vi "Vibration.vi"(0 "Channel 4":T5={"Frequency"=20, "Signal type"=enum."Sine Wave", "Amplitude"=2.0, "Offset"=0.0, "Phase"=0.0} {"Phase" format="%.2p"; "Offset" format="%0.2p"; "Amplitude" min=-2.0 max=2.0 step=0.1 format="%0.2p"}, 1 "Channel 3":T5={"Frequency"=20, "Signal type"=enum."Sine Wave", "Amplitude"=2.0, "Offset"=0.0, "Phase"=0.0} {"Phase" format="%.2p"; "Offset" format="%0.2p"; "Amplitude" min=-2.0 max=2.0 step=0.1 format="%0.2p"}, 2 "Channel 2":T5={"Frequency"=20, "Signal type"=enum."Sine Wave", "Amplitude"=2.0, "Offset"=0.0, "Phase"=0.0} {"Phase" format="%.2p"; "Offset" format="%0.2p"; "Amplitude" min=-2.0 max=2.0 step=0.1 format="%0.2p"}, 3 "Channel 1":T8={" Frequency"=20, "Signal type"=enum."Sine Wave", "Amplitude"=2.0, "Offset"=0.0, "Phase"=0.0} {"Phase" format="%.2p"; "Offset" format="%0.2p"; "Amplitude" min=-2.0 max=2.0 step=0.1 format="%0.2p"}, 4 "Time(ms)":i32, 5 "Model List":i32(listbox), 6 "Play Button":bool, 7 "Project Name":string, 9 "OK Button":bool, 10 "Remove Project":bool, 11 "Add Project":bool) -> (8 "Tab Control":enum32{"Main", "Project", "Set"}(tab)=enum."Project")   [LabVIEW 2019]
uses:
  Ctrl/UpLoad2.ctl
  Ctrl/Remove.ctl
  Typedef/Test_State.ctl
  Ctrl/left2arrow.ctl
  Ctrl/Right2arrow.ctl
  <vilib>/Utility/miscctls.llb/LVPointTypeDef.ctl
  <vilib>/Utility/miscctls.llb/LVPositionTypeDef.ctl
  Typedef/State.ctl
  Typedef/Data.ctl
  Typedef/Timer State.ctl
  LLB/Message/Ctrl/MsgDataInput.ctl
  LLB/Message/Ctrl/MsgPageSelect.ctl
  LLB/Message/Ctrl/LogType.ctl
  <vilib>/Utility/xml.llb/Read From XML File(string).vi
  LLB/Commonly VI/Main Glb.vi
  Class/Main Process Class/MPC_VirbVision/Panel RefGlb.vi
  SubVIs/GBV_Ref.vi
  <vilib>/Utility/xml.llb/Write to XML File(string).vi
  <vilib>/measure/NI_MABase.lvlib
  <vilib>/Utility/config.llb/NI_LVConfig.lvlib
  <resource>/objmgr/daqmx.rc
  LLB/Commonly VI.lvlib
  LLB/Message/MsgShowAndLog.lvlib
  <vilib>/Utility/config.llb/Read Key (String).vi
panel:
  in  "Reply":bool=TRUE
  in  "SubUI":bool=TRUE
  out "TCP connect":bool
  out "Array":string[](array[string])
  in  "Channel 4 Sample":cluster{"Sample Rate":dbl, "Samples":dbl} {"Samples" format="%#.2f"; "Sample Rate" format="%#.2f"}
  in  "Channel 3 Sample":cluster{"Sample Rate":dbl, "Samples":dbl} {"Samples" format="%#.2f"; "Sample Rate" format="%#.2f"}
  in  "Channel 2 Sample":cluster{"Sample Rate":dbl, "Samples":dbl} {"Samples" format="%#.2f"; "Sample Rate" format="%#.2f"}
  in  "Channel 1 Sample":cluster{"Sample Rate":dbl, "Samples":dbl} {"Samples" format="%#.2f"; "Sample Rate" format="%#.2f"}
  out "DataTable":T1(array[cluster])
  in  "Stop Button":bool
  in  "Center":T2={"Channel 1"={" frequency 1"=25, "signal type 1"=enum."Sine Wave", "amplitude 1"=1.25, "offset"=0, "phase"=0.0}, "Channel 2"={" frequency 1"=25, "signal type 1"=enum."Sine Wave", "amplitude 1"=1.25, "offset"=0, "phase"=90}, "Channel 3"={" frequency 1"=25, "signal type 1"=enum."Sine Wave", "amplitude 1"=1.25, "offset"=0, "phase"=180}, "Channel 4"={" frequency 1"=25, "signal type 1"=enum."Sine Wave", "amplitude 1"=1.25, "offset"=0, "phase"=270}}
  in  "Bump":T3={"Channel 1"={" frequency 1"=25, "signal type 1"=enum."Sine Wave", "amplitude 1"=2.0, "offset"=0, "phase"=0.0}, "Channel 2"={" frequency 1"=25, "signal type 1"=enum."Sine Wave", "amplitude 1"=2.0, "offset"=0, "phase"=0.0}, "Channel 3"={" frequency 1"=25, "signal type 1"=enum."Sine Wave", "amplitude 1"=2.0, "offset"=0, "phase"=0.0}, "Channel 4"={" frequency 1"=25, "signal type 1"=enum."Sine Wave", "amplitude 1"=2.0, "offset"=0, "phase"=0.0}}
  out "Test State":T4
  out "Testing?":bool
  out "Test Setting":waveform(dbl)[](array[waveform])
  in  "Blank Button":bool
  out "Running":bool
  out "Channel 1 Wave (Main)":waveform(dbl)(graph)
  in  "Center":bool
  in  "Bump":bool
  in  "Rightward":bool
  in  "Leftward":bool
  in  "Backward":bool
  in  "Frontward":bool
  out "Channel 2 Wave (Main)":waveform(dbl)(graph)
  out "Channel 3 Wave (Main)":waveform(dbl)(graph)
  out "Channel 4 Wave (Main)":waveform(dbl)(graph)
  in  "Setting(Main)":bool
  in  "Project(Main)":bool
  out "Connect":bool
  out "Current Project":string
  in  "Project List":i32(listbox)
  in  "Setting(Project)":bool
  out "Vibration State":bool
  in  "Simple Test(Project)":bool
  in  "Btn_DelSeqName":bool
  in  "Btn_AddSeqName":bool
  in  "SequenceName":u16(ring) items=["", "GGR", "RGG"]
  in  "TestListTrayRun":bool
  in  "SequenceList":i32(listbox)
  in  "Model Name":string
  in  "Save Button":bool
  in  "Remove":T6
  in  "Add":T7
  out "Channel 4 Wave":waveform(dbl)(graph)
  out "Channel 3 Wave":waveform(dbl)(graph)
  out "Channel 2 Wave":waveform(dbl)(graph)
  out "Channel 1 Wave":waveform(dbl)(graph)
  in  "Project(Setting)":bool
  out "Testing":bool
  out "Test Time(s)":dbl format="%#_2g"
  in  "Sampling rate":dbl=1000.0
  in  "Exit Button":bool
  in  "Simple Test(Setting)":bool
  in  "RemoveSeq":T9
  in  "AddSeq":T10
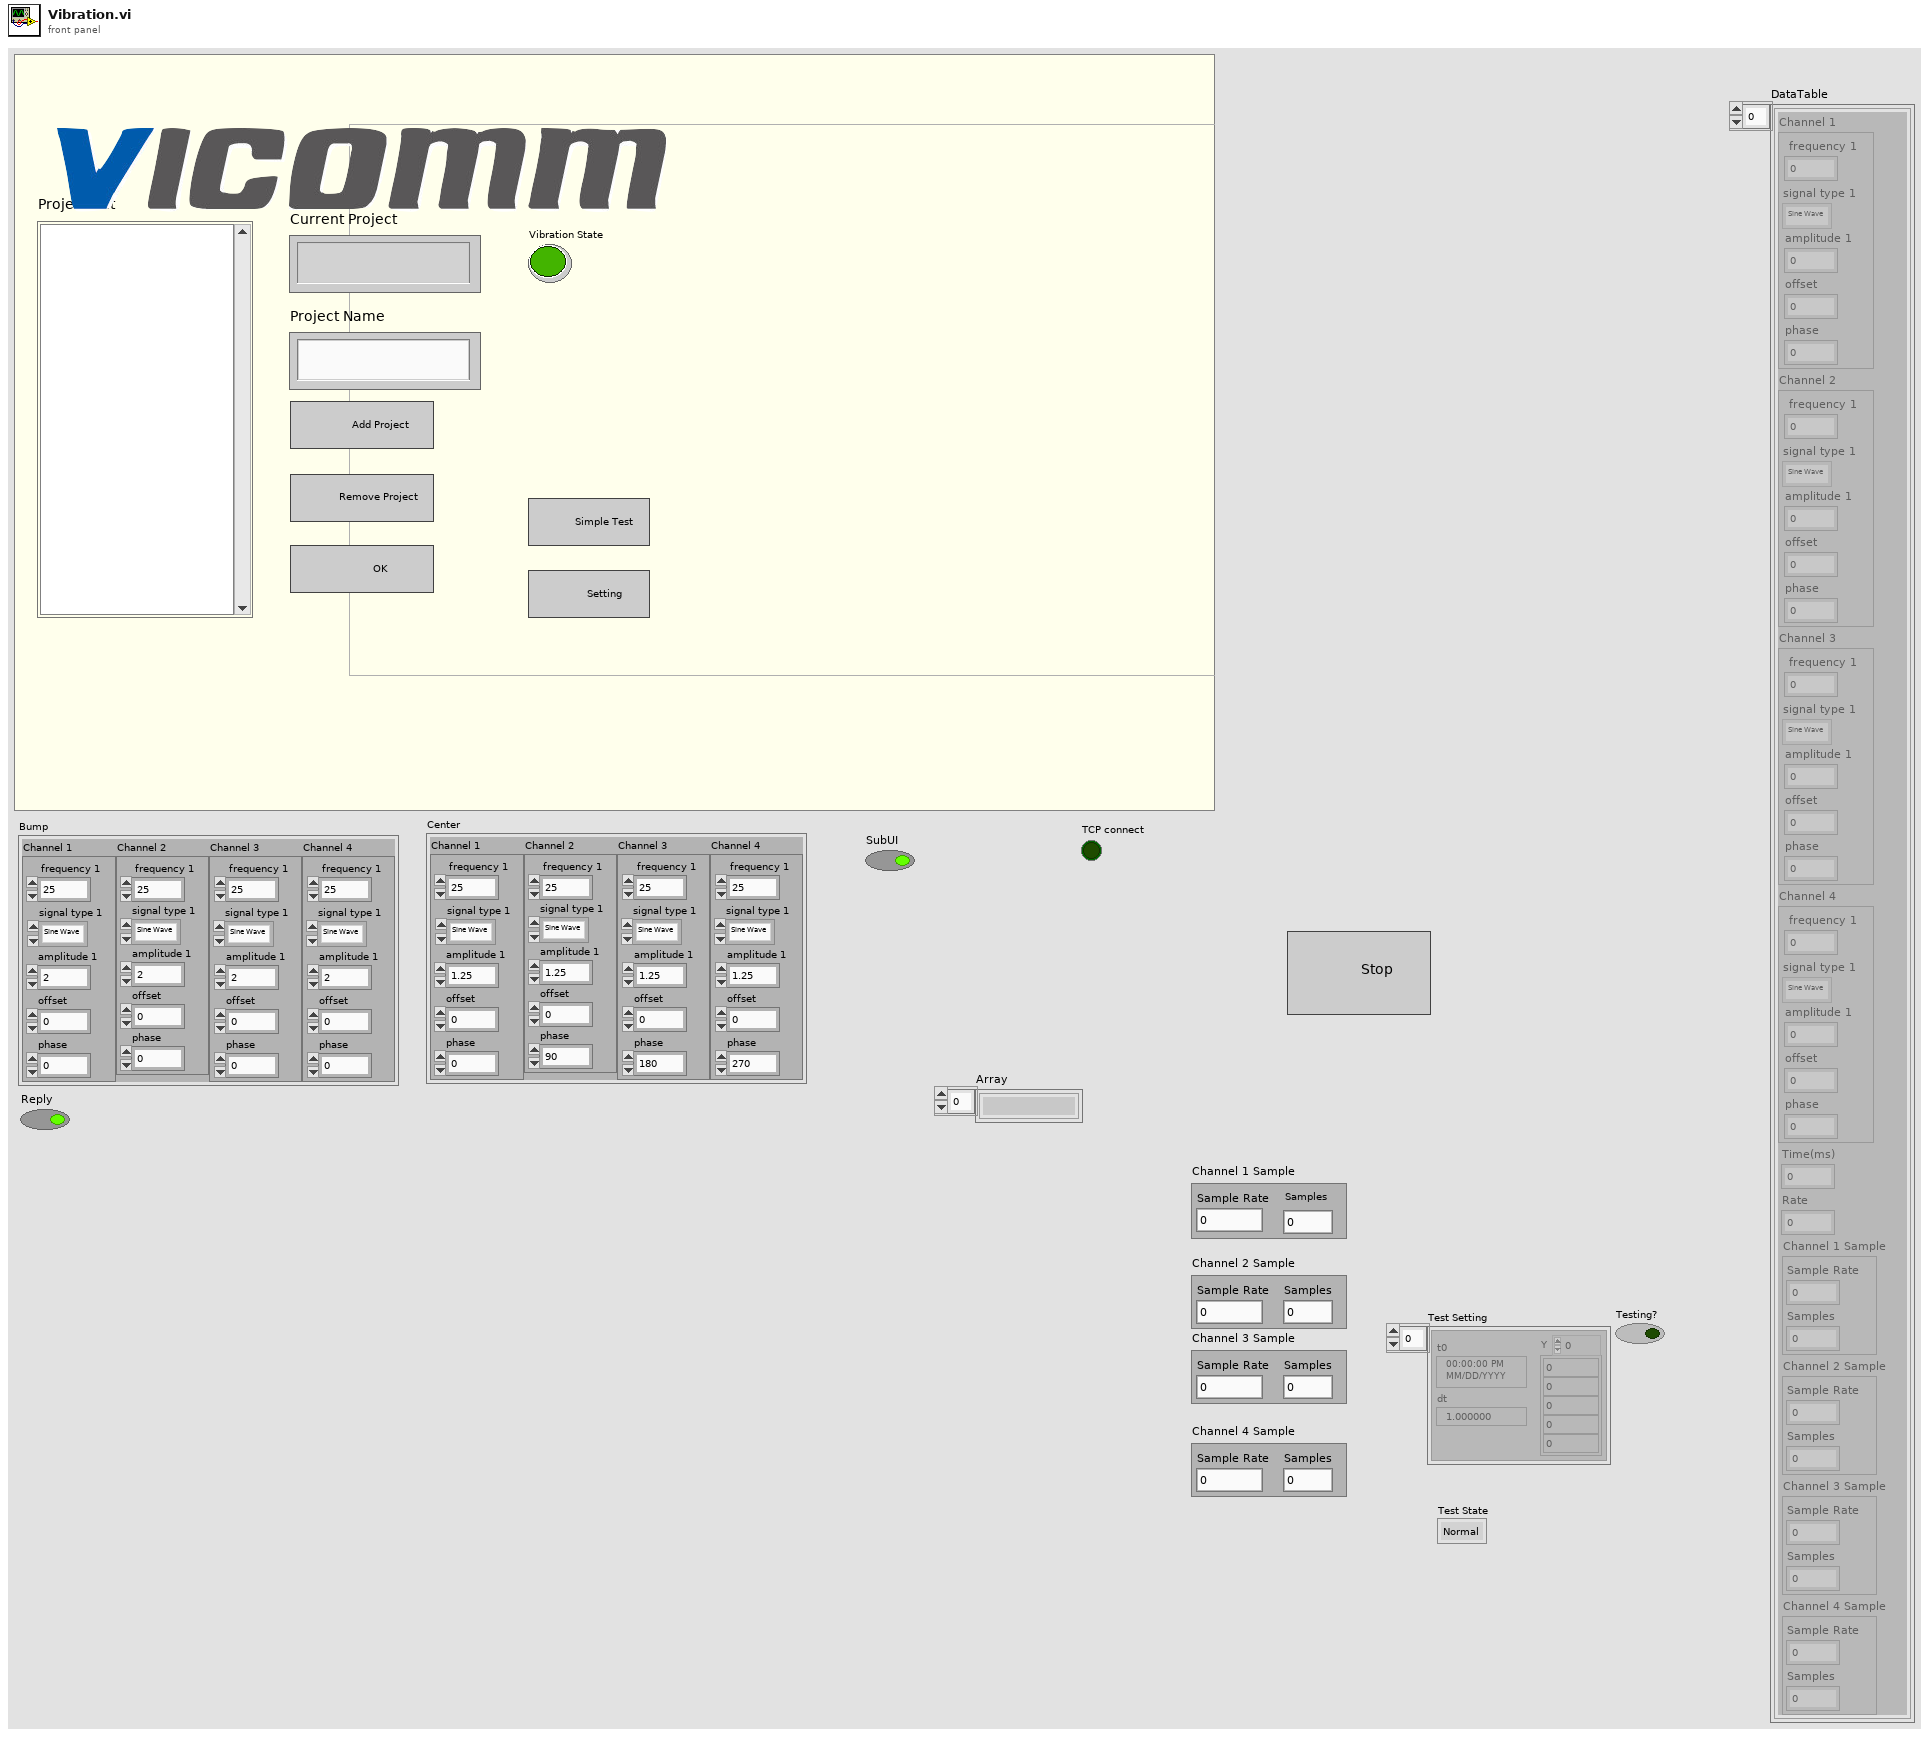
[diagram p1: front panel]
types:
  T1 = cluster{"Channel 1":cluster{" frequency 1":u32, "signal type 1":enum16{"Sine Wave", "Triangle Wave", "Square Wave", "Sawtooth Wave"}, "amplitude 1":dbl, "offset":dbl, "phase":dbl}, "Channel 2":cluster{" frequency 1":u32, "signal type 1":enum16{"Sine Wave", "Triangle Wave", "Square Wave", "Sawtooth Wave"}, "amplitude 1":dbl, "offset":dbl, "phase":dbl}, "Channel 3":cluster{" frequency 1":u32, "signal type 1":enum16{"Sine Wave", "Triangle Wave", "Square Wave", "Sawtooth Wave"}, "amplitude 1":dbl, "offset":dbl, "phase":dbl}, "Channel 4":cluster{" frequency 1":u32, "signal type 1":enum16{"Sine Wave", "Triangle Wave", "Square Wave", "Sawtooth Wave"}, "amplitude 1":dbl, "offset":dbl, "phase":dbl}, "Time(ms)":i32, "Rate":dbl, "Channel 1 Sample":cluster{"Sample Rate":dbl, "Samples":dbl}, "Channel 2 Sample":cluster{"Sample Rate":dbl, "Samples":dbl}, "Channel 3 Sample":cluster{"Sample Rate":dbl, "Samples":dbl}, "Channel 4 Sample":cluster{"Sample Rate":dbl, "Samples":dbl}}[]
  T2 = cluster{"Channel 1":cluster{" frequency 1":i32, "signal type 1":enum16{"Sine Wave", "Triangle Wave", "Square Wave", "Sawtooth Wave"}, "amplitude 1":dbl, "offset":i32, "phase":dbl}, "Channel 2":cluster{" frequency 1":i32, "signal type 1":enum16{"Sine Wave", "Triangle Wave", "Square Wave", "Sawtooth Wave"}, "amplitude 1":dbl, "offset":i32, "phase":i32}, "Channel 3":cluster{" frequency 1":i32, "signal type 1":enum16{"Sine Wave", "Triangle Wave", "Square Wave", "Sawtooth Wave"}, "amplitude 1":dbl, "offset":i32, "phase":i32}, "Channel 4":cluster{" frequency 1":i32, "signal type 1":enum16{"Sine Wave", "Triangle Wave", "Square Wave", "Sawtooth Wave"}, "amplitude 1":dbl, "offset":i32, "phase":i32}}
  T3 = cluster{"Channel 1":cluster{" frequency 1":i32, "signal type 1":enum16{"Sine Wave", "Triangle Wave", "Square Wave", "Sawtooth Wave"}, "amplitude 1":dbl, "offset":i32, "phase":dbl}, "Channel 2":cluster{" frequency 1":i32, "signal type 1":enum16{"Sine Wave", "Triangle Wave", "Square Wave", "Sawtooth Wave"}, "amplitude 1":dbl, "offset":i32, "phase":dbl}, "Channel 3":cluster{" frequency 1":i32, "signal type 1":enum16{"Sine Wave", "Triangle Wave", "Square Wave", "Sawtooth Wave"}, "amplitude 1":dbl, "offset":i32, "phase":dbl}, "Channel 4":cluster{" frequency 1":i32, "signal type 1":enum16{"Sine Wave", "Triangle Wave", "Square Wave", "Sawtooth Wave"}, "amplitude 1":dbl, "offset":i32, "phase":dbl}}
  T4 = typedef "Test_State.ctl" = enum16{"Normal", "Bump", "Center"}
  T5 = cluster{"Frequency":u32, "Signal type":enum16{"Sine Wave", "Triangle Wave", "Square Wave", "Sawtooth Wave"}, "Amplitude":dbl, "Offset":dbl, "Phase":dbl}
  T6 = typedef "Remove.ctl" = bool
  T7 = typedef "UpLoad2.ctl" = bool
  T8 = cluster{" Frequency":u32, "Signal type":enum16{"Sine Wave", "Triangle Wave", "Square Wave", "Sawtooth Wave"}, "Amplitude":dbl, "Offset":dbl, "Phase":dbl}
  T9 = typedef "left2arrow.ctl" = bool
  T10 = typedef "Right2arrow.ctl" = bool
  T11 = cluster{"seconds since 1Jan1904":timestamp, timestamp}
  T12 = enum16{"open", "replace", "create", "open or create", "replace or create", "replace or create with confirmation"}
  T13 = typedef "LVPositionTypeDef.ctl" = cluster{"Left":i32, "Top":i32}
  T14 = typedef "LVPointTypeDef.ctl" = cluster{"Horizontal":i16, "Vertical":i16}
  T15 = typedef "State.ctl" = enum16{"Initalize", "Idle", "Update", "Channel1", "Channel2", "Channel3", "Channel4", "Channel1 Sample", "Channel2 Sample", "Channel3 Sample", "Channel4 Sample", "Waveform", "DAQ Rate", "ModelList", "Add", "Remove", "Set Time", "Test", "Start Time", "Check Time", "Save", "Frontward", "Leftward", "Backward", "Rightward", "Stop", "Center", "Bump", "Add Project", "Remove Project", "Project List", "Project Name", "Project OK", "Response", "Exit"}
  T16 = typedef "Data.ctl" = cluster{"Channel Table":cluster{"Channel 1":cluster{" frequency 1":u32, "signal type 1":enum16{"Sine Wave", "Triangle Wave", "Square Wave", "Sawtooth Wave"}, "amplitude 1":dbl, "offset":dbl, "phase":dbl}, "Channel 2":cluster{" frequency 1":u32, "signal type 1":enum16{"Sine Wave", "Triangle Wave", "Square Wave", "Sawtooth Wave"}, "amplitude 1":dbl, "offset":dbl, "phase":dbl}, "Channel 3":cluster{" frequency 1":u32, "signal type 1":enum16{"Sine Wave", "Triangle Wave", "Square Wave", "Sawtooth Wave"}, "amplitude 1":dbl, "offset":dbl, "phase":dbl}, "Channel 4":cluster{" frequency 1":u32, "signal type 1":enum16{"Sine Wave", "Triangle Wave", "Square Wave", "Sawtooth Wave"}, "amplitude 1":dbl, "offset":dbl, "phase":dbl}, "Time(ms)":i32, "Rate":dbl, "Channel 1 Sample":cluster{"Sample Rate":dbl, "Samples":dbl}, "Channel 2 Sample":cluster{"Sample Rate":dbl, "Samples":dbl}, "Channel 3 Sample":cluster{"Sample Rate":dbl, "Samples":dbl}, "Channel 4 Sample":cluster{"Sample Rate":dbl, "Samples":dbl}}[], "Model List name":string[], "Channel 1 Wave":waveform(dbl), "Channel 2 Wave":waveform(dbl), "Channel 3 Wave":waveform(dbl), "Channel 4 Wave":waveform(dbl), "Testing":bool, "Set Time":i32, "Elapse Time":dbl, "Channel 1":cluster{" frequency 1":u32, "signal type 1":enum16{"Sine Wave", "Triangle Wave", "Square Wave", "Sawtooth Wave"}, "amplitude 1":dbl, "offset":dbl, "phase":dbl}, "Channel 2":cluster{" frequency 1":u32, "signal type 1":enum16{"Sine Wave", "Triangle Wave", "Square Wave", "Sawtooth Wave"}, "amplitude 1":dbl, "offset":dbl, "phase":dbl}, "Channel 3":cluster{" frequency 1":u32, "signal type 1":enum16{"Sine Wave", "Triangle Wave", "Square Wave", "Sawtooth Wave"}, "amplitude 1":dbl, "offset":dbl, "phase":dbl}, "Channel 4":cluster{" frequency 1":u32, "signal type 1":enum16{"Sine Wave", "Triangle Wave", "Square Wave", "Sawtooth Wave"}, "amplitude 1":dbl, "offset":dbl, "phase":dbl}, "ModelList Num":i32, "Stop":bool, "Button":bool, "Button Time":i32, "Elapsed ?":bool, "Channel 1 Wave (Main)":waveform(dbl), "Channel 2 Wave (Main)":waveform(dbl), "Channel 3 Wave (Main)":waveform(dbl), "Channel 4 Wave (Main)":waveform(dbl), "Project List name":string[], "Project Name":string, "Project Path":path, "ProjectList Num":i32, "Project Name(Set)":string, "Rate":dbl, "Channel 1 Sample":cluster{"Sample Rate":dbl, "Samples":dbl}, "Channel 2 Sample":cluster{"Sample Rate":dbl, "Samples":dbl}, "Channel 3 Sample":cluster{"Sample Rate":dbl, "Samples":dbl}, "Channel 4 Sample":cluster{"Sample Rate":dbl, "Samples":dbl}}
  T17 = enum16{"Standard", "Buffered", "CRLF", "Immediate"}
  T18 = typedef "MsgDataInput.ctl" = cluster{"MsgPageSelect":T19, "LogType":T20, "Msg":string, "Time":string}
  T19 = typedef "MsgShowAndLog.lvlib/MsgPageSelect.ctl" = enum16{"System", "Comm", "IO", "Action", "Alarm"}
  T20 = typedef "MsgShowAndLog.lvlib/LogType.ctl" = enum16{"Auto", "Manual", "Handshake", "Error"}
  T21 = enum16{"Initial", "Write", "Read", "Save", "Load", "WrteAll"}
  T22 = enum16{"Initial", "Write", "Read", "Save", "Load", "Add", "Delete"}
  T23 = cluster{" frequency 1":u32, "signal type 1":enum16{"Sine Wave", "Triangle Wave", "Square Wave", "Sawtooth Wave"}, "amplitude 1":dbl, "offset":dbl, "phase":dbl}
  T24 = typedef "Timer State.ctl" = enum16{"Start", "Check"}
  T25 = cluster{"Channel 1":cluster{" frequency 1":i32, "signal type 1":enum16{"Sine Wave", "Triangle Wave", "Square Wave", "Sawtooth Wave"}, "amplitude 1":dbl, "offset":dbl, "phase":dbl}, "Channel 2":cluster{" frequency 1":i32, "signal type 1":enum16{"Sine Wave", "Triangle Wave", "Square Wave", "Sawtooth Wave"}, "amplitude 1":dbl, "offset":dbl, "phase":i32}, "Channel 3":cluster{" frequency 1":i32, "signal type 1":enum16{"Sine Wave", "Triangle Wave", "Square Wave", "Sawtooth Wave"}, "amplitude 1":dbl, "offset":dbl, "phase":dbl}, "Channel 4":cluster{" frequency 1":i32, "signal type 1":enum16{"Sine Wave", "Triangle Wave", "Square Wave", "Sawtooth Wave"}, "amplitude 1":dbl, "offset":dbl, "phase":i32}}
  T26 = enum8{"Enabled", "Disabled", "Disabled and Grayed Out"}
  T27 = cluster{" frequency 1":i32, "signal type 1":enum16{"Sine Wave", "Triangle Wave", "Square Wave", "Sawtooth Wave"}, "amplitude 1":dbl, "offset":i32, "phase":dbl}
  T28 = cluster{" frequency 1":i32, "signal type 1":enum16{"Sine Wave", "Triangle Wave", "Square Wave", "Sawtooth Wave"}, "amplitude 1":dbl, "offset":i32, "phase":i32}
  T29 = cluster{" frequency 1":i32, "signal type 1":enum16{"Sine Wave", "Triangle Wave", "Square Wave", "Sawtooth Wave"}, "amplitude 1":dbl, "offset":i32, "phase":dbl}[]
  T30 = enum16{"Sine Wave", "Triangle Wave", "Square Wave", "Sawtooth Wave"}
  T31 = typedef "NI_LVConfig.lvlib/Config Data RefNum.ctl" = refnum<k1>
  T32 = cluster{"DataTable":cluster{"Channel 1":cluster{" frequency 1":u32, "signal type 1":enum16{"Sine Wave", "Triangle Wave", "Square Wave", "Sawtooth Wave"}, "amplitude 1":dbl, "offset":dbl, "phase":dbl}, "Channel 2":cluster{" frequency 1":u32, "signal type 1":enum16{"Sine Wave", "Triangle Wave", "Square Wave", "Sawtooth Wave"}, "amplitude 1":dbl, "offset":dbl, "phase":dbl}, "Channel 3":cluster{" frequency 1":u32, "signal type 1":enum16{"Sine Wave", "Triangle Wave", "Square Wave", "Sawtooth Wave"}, "amplitude 1":dbl, "offset":dbl, "phase":dbl}, "Channel 4":cluster{" frequency 1":u32, "signal type 1":enum16{"Sine Wave", "Triangle Wave", "Square Wave", "Sawtooth Wave"}, "amplitude 1":dbl, "offset":dbl, "phase":dbl}, "Time(ms)":i32, "Rate":dbl, "Channel 1 Sample":cluster{"Sample Rate":dbl, "Samples":dbl}, "Channel 2 Sample":cluster{"Sample Rate":dbl, "Samples":dbl}, "Channel 3 Sample":cluster{"Sample Rate":dbl, "Samples":dbl}, "Channel 4 Sample":cluster{"Sample Rate":dbl, "Samples":dbl}}[], "Item Names":string[]}
  T33 = cluster{"VirbSeqName":string, "VirbSeqStep":string[]}[]
  T34 = cluster{"Channel 1":cluster{" frequency 1":u32, "signal type 1":enum16{"Sine Wave", "Triangle Wave", "Square Wave", "Sawtooth Wave"}, "amplitude 1":dbl, "offset":dbl, "phase":dbl}, "Channel 2":cluster{" frequency 1":u32, "signal type 1":enum16{"Sine Wave", "Triangle Wave", "Square Wave", "Sawtooth Wave"}, "amplitude 1":dbl, "offset":dbl, "phase":dbl}, "Channel 3":cluster{" frequency 1":u32, "signal type 1":enum16{"Sine Wave", "Triangle Wave", "Square Wave", "Sawtooth Wave"}, "amplitude 1":dbl, "offset":dbl, "phase":dbl}, "Channel 4":cluster{" frequency 1":u32, "signal type 1":enum16{"Sine Wave", "Triangle Wave", "Square Wave", "Sawtooth Wave"}, "amplitude 1":dbl, "offset":dbl, "phase":dbl}, "Time(ms)":i32, "Rate":dbl, "Channel 1 Sample":cluster{"Sample Rate":dbl, "Samples":dbl}, "Channel 2 Sample":cluster{"Sample Rate":dbl, "Samples":dbl}, "Channel 3 Sample":cluster{"Sample Rate":dbl, "Samples":dbl}, "Channel 4 Sample":cluster{"Sample Rate":dbl, "Samples":dbl}}
  T35 = cluster{" frequency 1":u32, "signal type 1":enum16{"Sine Wave", "Triangle Wave", "Square Wave", "Sawtooth Wave"}, "amplitude 1":dbl, "offset":dbl, "phase":dbl}[]
  T36 = cluster{"Channel Table":cluster{"Channel 1":cluster{" frequency 1":u32, "signal type 1":enum16{"Sine Wave", "Triangle Wave", "Square Wave", "Sawtooth Wave"}, "amplitude 1":dbl, "offset":dbl, "phase":dbl}, "Channel 2":cluster{" frequency 1":u32, "signal type 1":enum16{"Sine Wave", "Triangle Wave", "Square Wave", "Sawtooth Wave"}, "amplitude 1":dbl, "offset":dbl, "phase":dbl}, "Channel 3":cluster{" frequency 1":u32, "signal type 1":enum16{"Sine Wave", "Triangle Wave", "Square Wave", "Sawtooth Wave"}, "amplitude 1":dbl, "offset":dbl, "phase":dbl}, "Channel 4":cluster{" frequency 1":u32, "signal type 1":enum16{"Sine Wave", "Triangle Wave", "Square Wave", "Sawtooth Wave"}, "amplitude 1":dbl, "offset":dbl, "phase":dbl}, "Time(ms)":i32, "Rate":dbl, "Channel 1 Sample":cluster{"Sample Rate":dbl, "Samples":dbl}, "Channel 2 Sample":cluster{"Sample Rate":dbl, "Samples":dbl}, "Channel 3 Sample":cluster{"Sample Rate":dbl, "Samples":dbl}, "Channel 4 Sample":cluster{"Sample Rate":dbl, "Samples":dbl}}[], "Model List name":string[]}
  T37 = cluster{" frequency 1":i32, "signal type 1":enum16{"Sine Wave", "Triangle Wave", "Square Wave", "Sawtooth Wave"}, "amplitude 1":dbl, "offset":dbl, "phase":dbl}
  T38 = cluster{" frequency 1":i32, "signal type 1":enum16{"Sine Wave", "Triangle Wave", "Square Wave", "Sawtooth Wave"}, "amplitude 1":dbl, "offset":dbl, "phase":i32}
  T39 = cluster{" frequency 1":i32, "signal type 1":enum16{"Sine Wave", "Triangle Wave", "Square Wave", "Sawtooth Wave"}, "amplitude 1":dbl, "offset":dbl, "phase":dbl}[]
  T40 = cluster{"State":T15, "Channel 1":cluster{" Frequency":u32, "Signal type":enum16{"Sine Wave", "Triangle Wave", "Square Wave", "Sawtooth Wave"}, "Amplitude":dbl, "Offset":dbl, "Phase":dbl}}
  T41 = cluster{"State":T15, "Channel 2":cluster{"Frequency":u32, "Signal type":enum16{"Sine Wave", "Triangle Wave", "Square Wave", "Sawtooth Wave"}, "Amplitude":dbl, "Offset":dbl, "Phase":dbl}}
  T42 = cluster{"State":T15, "Channel 3":cluster{"Frequency":u32, "Signal type":enum16{"Sine Wave", "Triangle Wave", "Square Wave", "Sawtooth Wave"}, "Amplitude":dbl, "Offset":dbl, "Phase":dbl}}
  T43 = cluster{"State":T15, "Channel 4":cluster{"Frequency":u32, "Signal type":enum16{"Sine Wave", "Triangle Wave", "Square Wave", "Sawtooth Wave"}, "Amplitude":dbl, "Offset":dbl, "Phase":dbl}}
  T44 = cluster{"State":T15, "Channel 1 Sample":cluster{"Sample Rate":dbl, "Samples":dbl}}
  T45 = cluster{"State":T15, "Channel 2 Sample":cluster{"Sample Rate":dbl, "Samples":dbl}}
  T46 = cluster{"State":T15, "Channel 3 Sample":cluster{"Sample Rate":dbl, "Samples":dbl}}
  T47 = cluster{"State":T15, "Channel 4 Sample":cluster{"Sample Rate":dbl, "Samples":dbl}}
  T48 = cluster{"RingText.Text":string, "Item Names":string[]}
  T49 = cluster{"VirbSeqName":string, "VirbSeqStep":string[]}
  T50 = cluster{"Bump":refnum<vi>, "Frontward":refnum<vi>, "Leftward":refnum<vi>, "Backward":refnum<vi>, "Rightward":refnum<vi>, "Center":refnum<vi>, "Testing?":refnum<vi>}
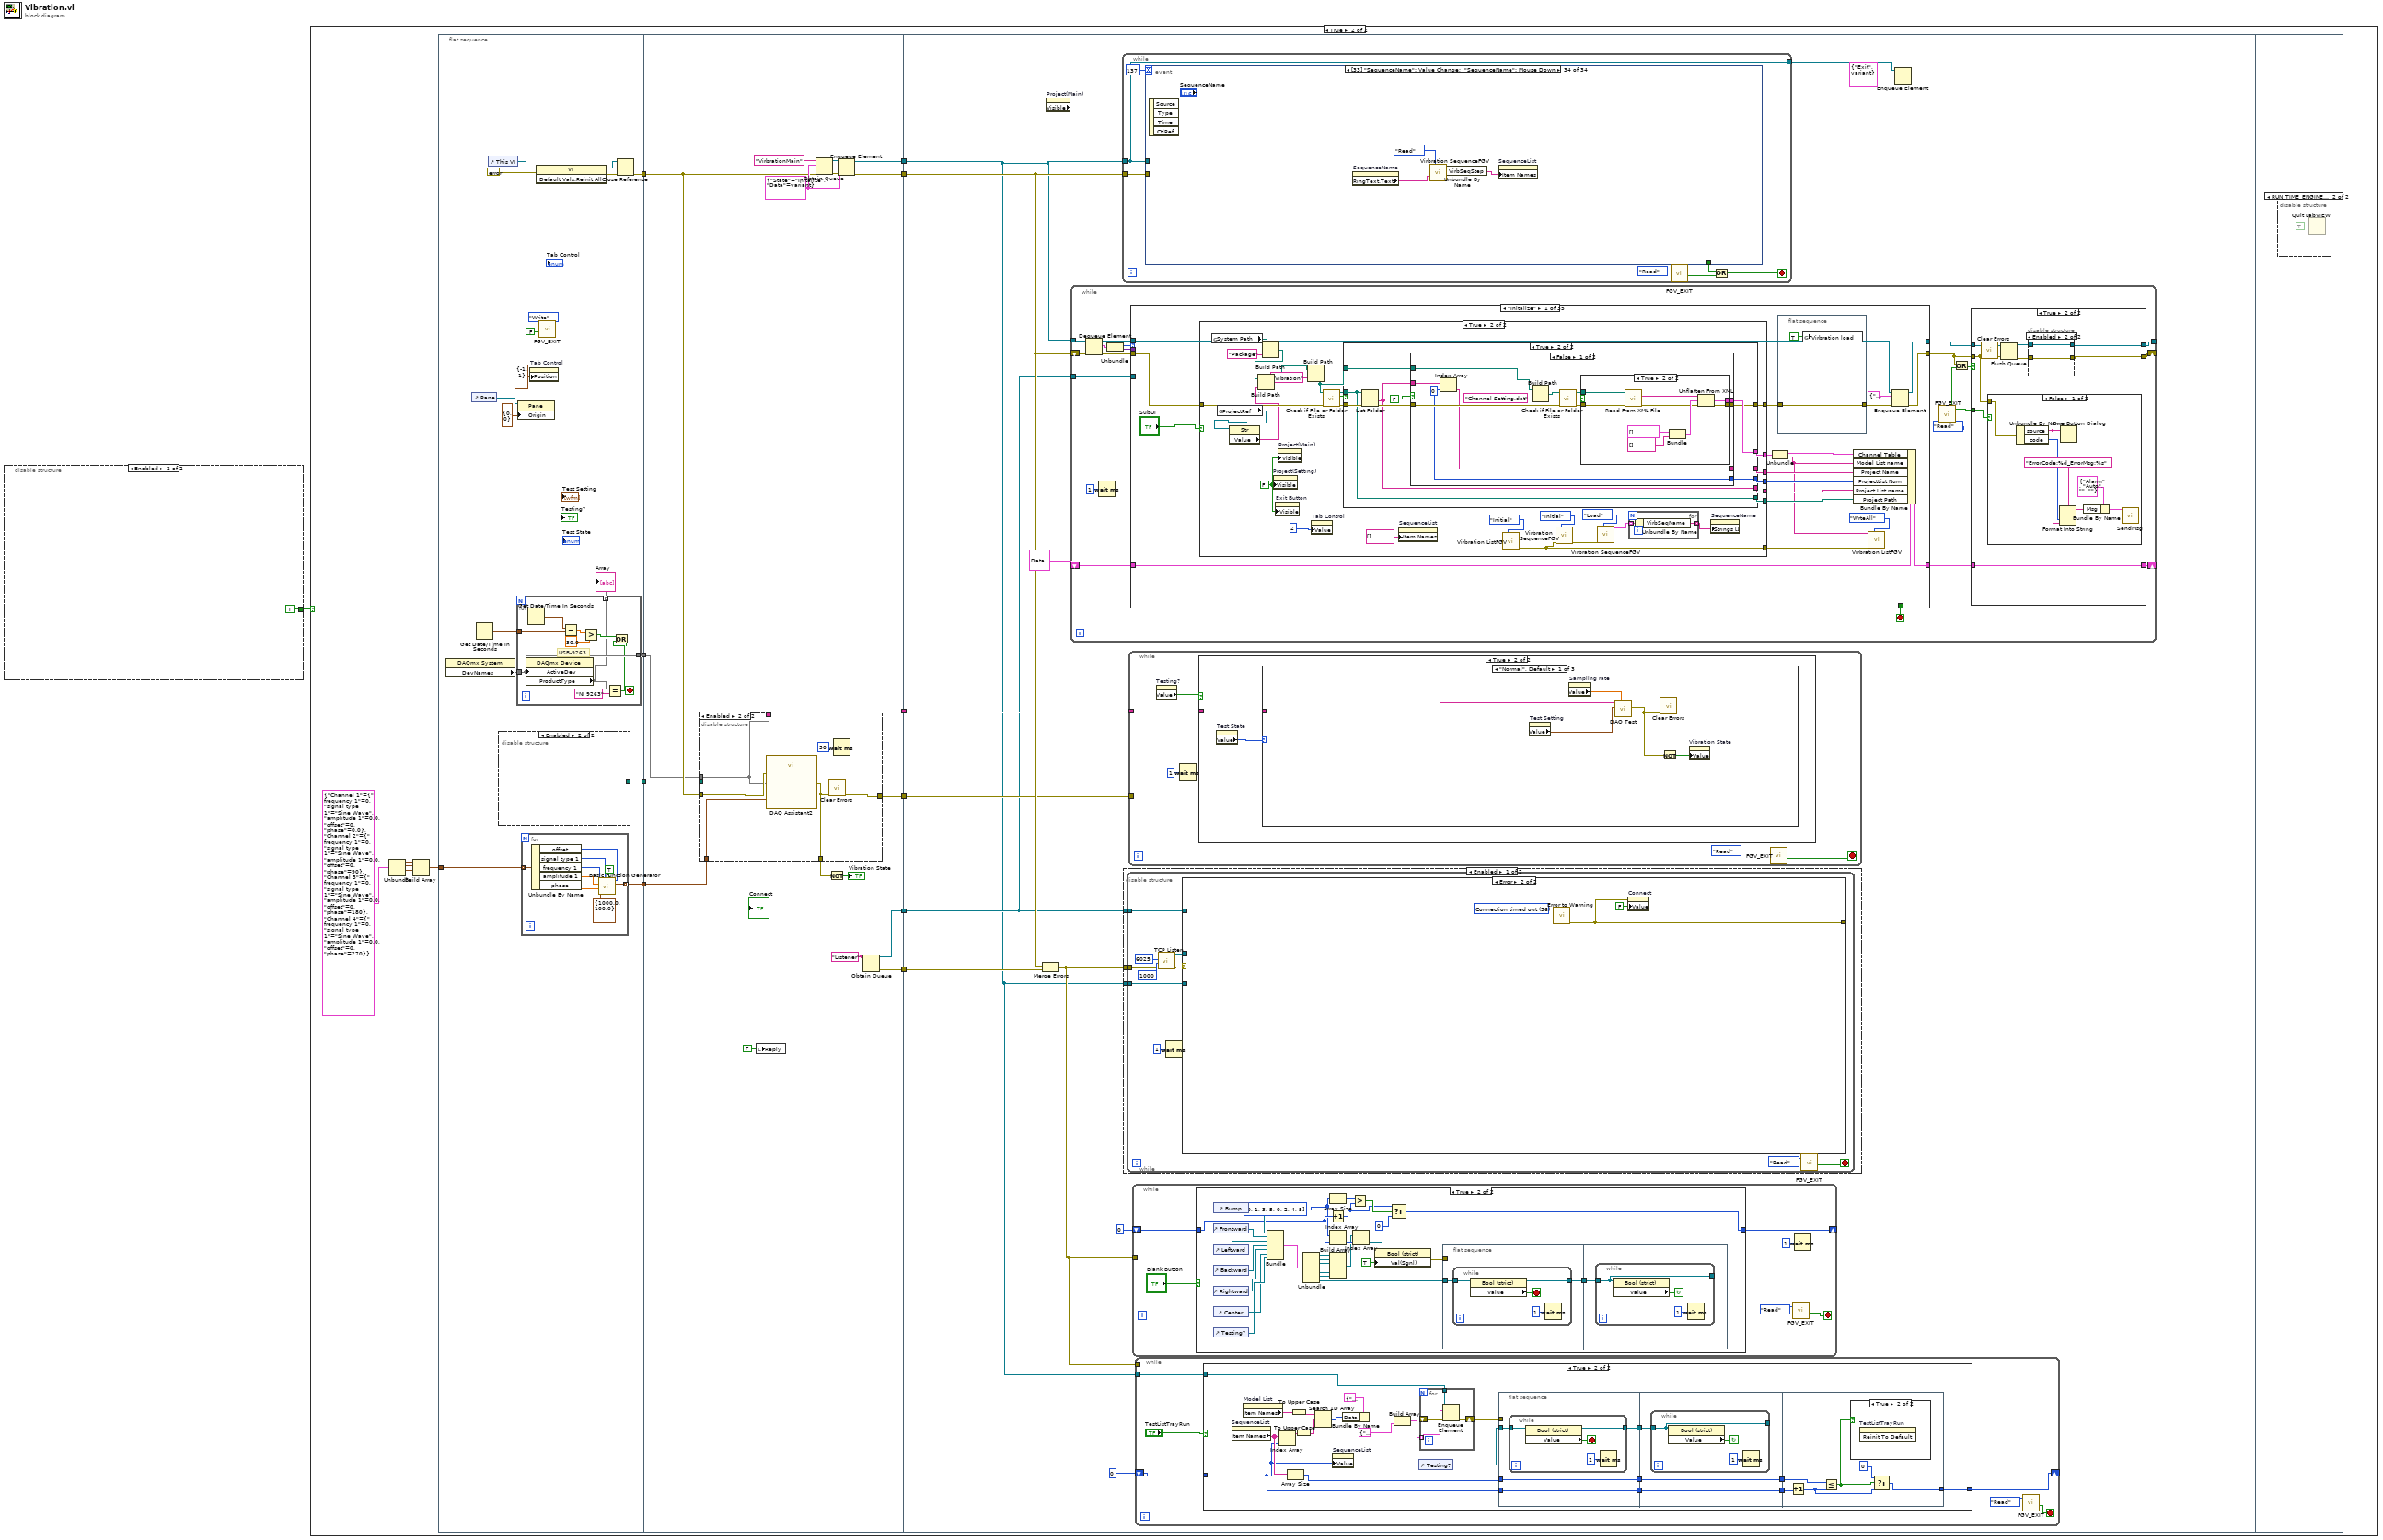
[diagram p0: block diagram]
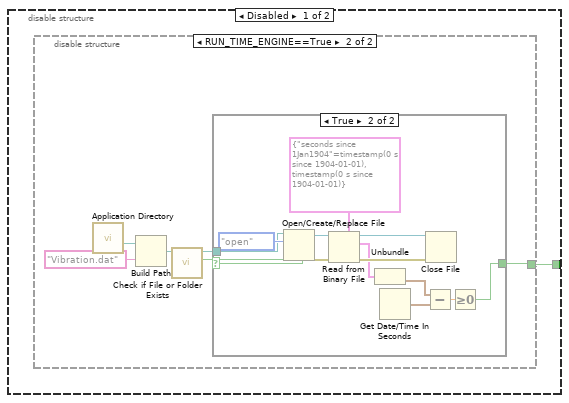
[diagram p2: hidden frame]
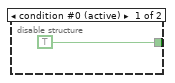
[diagram p3: hidden frame]
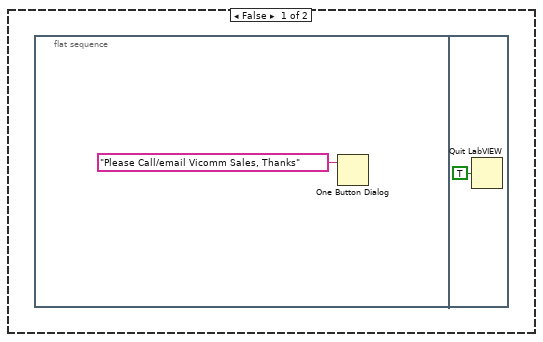
[diagram p5: hidden frame]
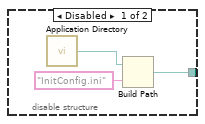
[diagram p6: hidden frame]
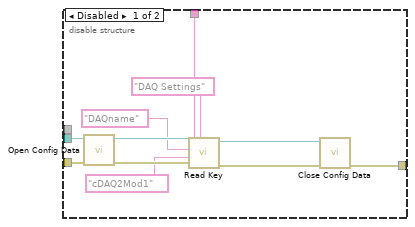
[diagram p7: hidden frame]
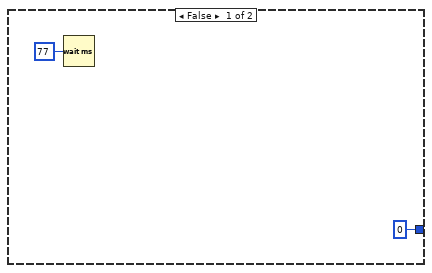
[diagram p8: hidden frame]
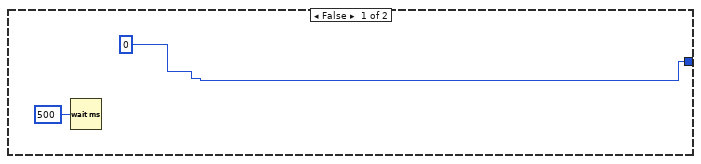
[diagram p10: hidden frame]
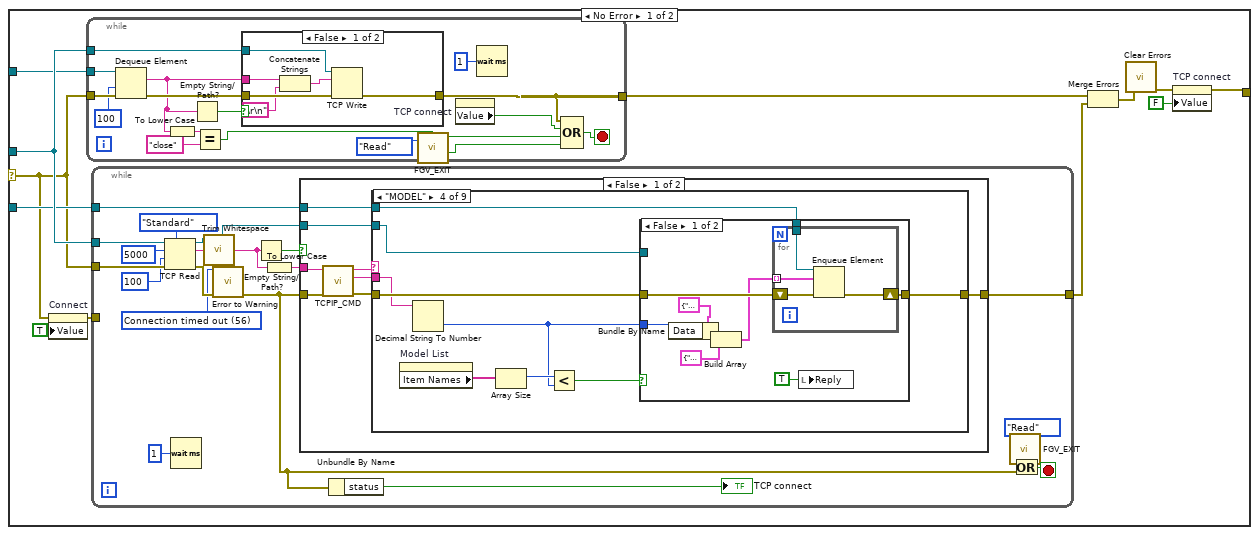
[diagram p11: hidden frame]
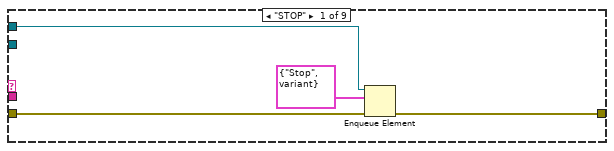
[diagram p12: hidden frame]
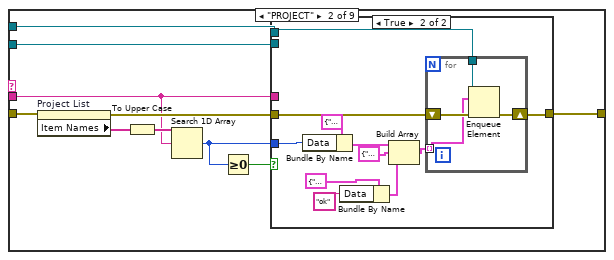
[diagram p13: hidden frame]
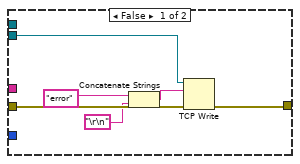
[diagram p14: hidden frame]
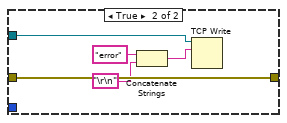
[diagram p16: hidden frame]
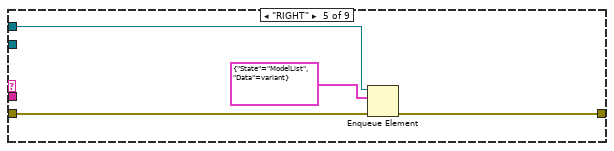
[diagram p17: hidden frame]
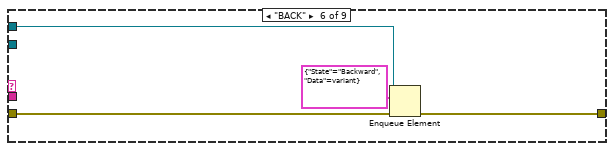
[diagram p18: hidden frame]
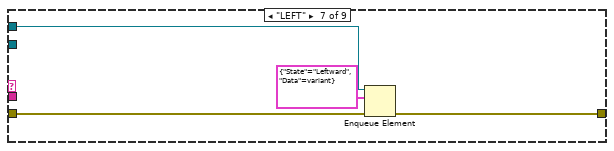
[diagram p19: hidden frame]
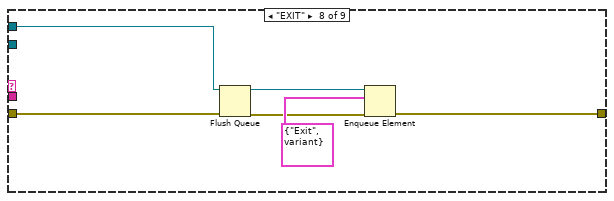
[diagram p20: hidden frame]
diagram:
  n1 = disable-structure shown="Enabled" {
    disable-tunnel: [w2 TRUE] -> w1
    frame Disabled {
      n2 = disable-structure shown="RUN_TIME_ENGINE==True" {
        disable-tunnel: [TRUE w4] -> w2
        frame condition #0 (active) {
        }
        frame condition #1 {
          n3 = call <vilib>:"Application Directory.vi"() -> ("Application Directory"=w9:path)
          n4 = Build Path(base path=w9, name or relative path="Vibration.dat") -> (appended path=w7:path)
          n5 = call <vilib>:"Check if File or Folder Exists.vi"("path"=w7) -> ("file or folder exists?"=w6:bool, "dup path"=w5:path)  [unwired: 8 in, 1 out]
          n6 = case shown="True" w6 {
            selector: w6 -> [w10 _]
            tunnel: w5 -> [_ w11]
            tunnel: [w10 w12] -> w4
            frame False {
            }
            frame True {
              n7 = Open/Create/Replace File(file path (use dialog)=w11, operation (0:open)=T12."open") -> (refnum out=w21:refnum<file>, error out=w20:errorcluster)  [unwired: 4 in, 1 out]
              n8 = Read from Binary File(5:T11 {"seconds since 1Jan1904"=timestamp(0 s since 1904-01-01), timestamp(0 s since 1904-01-01)} ("cluster"), 8:w20, 11:w21) -> (0:w19:errorcluster, 2:w17:T11, 3:w18:refnum<file>)  [unwired: 3 in, 1 out]
              n9 = Unbundle(w17) -> (w15:timestamp)  [unwired: 1 out]
              n10 = Get Date/Time In Seconds() -> (seconds since 1Jan1904=w16:timestamp)
              n11 = Subtract(x=w15, y=w16) -> (x-y=w13:dbl)
              n12 = Close File(refnum=w18, error in=w19) -> ()  [unwired: 2 out]
              n13 = Greater Or Equal To 0?(x=w13) -> (x >= 0?=w12:bool)
            }
          }
        }
      }
    }
    frame Enabled {
    }
  }
  n14 = case shown="True" w1 {
    frame False {
      n15 = flat-sequence {
        frame #0 {
          n16 = One Button Dialog(message="Please Call/email Vicomm Sales, Thanks") -> ()  [unwired: 1 in, 1 out]
        }
        frame #1 {
          n17 = Quit LabVIEW(quit? (T)=TRUE) -> ()
        }
      }
    }
    frame True {
      n18 = Unbundle(T2 {"Channel 1"={" frequency 1"=0, "signal type 1"=enum."Sine Wave", "amplitude 1"=0.0, "offset"=0, "phase"=0.0}, "Channel 2"={" frequency 1"=0, "signal type 1"=enum."Sine Wave", "amplitude 1"=0.0, "offset"=0, "phase"=90}, "Channel 3"={" frequency 1"=0, "signal type 1"=enum."Sine Wave", "amplitude 1"=0.0, "offset"=0, "phase"=180}, "Channel 4"={" frequency 1"=0, "signal type 1"=enum."Sine Wave", "amplitude 1"=0.0, "offset"=0, "phase"=270}} ("Center")) -> ("Channel 1"=w31:T27, "Channel 2"=w30:T28, "Channel 3"=w29:T28, "Channel 4"=w28:T28)
      n19 = Build Array(w31, w30, w29, w28) -> (w27:T29)
      n20 = flat-sequence {
        tunnel: [w55] -> w41
        tunnel: [w51] -> w40
        tunnel: w27 -> [w50]
        tunnel: [w49] -> w39
        tunnel: [w47] -> w26
        tunnel: [w94] -> w38
        tunnel: [w93] -> w37
        tunnel: w41 -> [w89]
        tunnel: [w91] -> w36
        tunnel: [w90] -> w35
        tunnel: w40 -> [w88]
        tunnel: [w87] -> w34
        tunnel: [w86] -> w33
        tunnel: w39 -> [w85]
        tunnel: w26 -> [w82]
        tunnel: w38 -> [w117]
        tunnel: w37 -> [w126]
        tunnel: w36 -> [w121]
        tunnel: w35 -> [w127]
        tunnel: w34 -> [w125]
        tunnel: w33 -> [w124]
        frame #0 {
          # "USB-9263"
          n21 = property class="DAQmx System"() -> ("DevNames"=w48)  [unwired: 2 in, 2 out]
          n22 = control-ref of="Pane"() -> (w44:refnum<vi>)
          n23 = Get Date/Time In Seconds() -> (seconds since 1Jan1904=w46:timestamp)
          n24 = control-ref of="This VI"() -> (w58:refnum<vi>)
          n25 = disable-structure shown="Enabled" {
            disable-tunnel: [w78 _] -> w51
            frame Disabled {
              n26 = call <vilib>:"Application Directory.vi"() -> ("Application Directory"=w80:path)
              n27 = Build Path(base path=w80, name or relative path="InitConfig.ini") -> (appended path=w78:path)
            }
            frame Enabled {
            }
          }
          n28 = for {
            tunnel: w48 -> [w67]
            tunnel: [w67] -> w47
            tunnel: w46 -> [w66]
            tunnel: [w59] -> w45 mode=indexing
            stop <- w60 stop-if-true
            n29 = property class="DAQmx Device"("ActiveDev"=w67) -> ("ProductType"=w59)  [unwired: 2 in, 2 out]
            n30 = Get Date/Time In Seconds() -> (seconds since 1Jan1904=w65:timestamp)
            n31 = Subtract(x=w65, y=w66) -> (x-y=w64:dbl)
            n32 = Greater?(x=w64, y=30.0) -> (0:w62:bool)
            n33 = Equal?(x=w59, y="NI 9263") -> (x = y?=w61:bool)
            n34 = Or(x=w62, y=w61) -> (x .or. y?=w60:bool)
          }
          "Array" <- w45
          n35 = property class="Pane"(reference=w44, "Origin"=T14 {"Horizontal"=0, "Vertical"=0}) -> ()  [unwired: 1 in, 2 out]
          n36 = for {
            tunnel: w50 -> [w69] mode=indexing
            tunnel: [w70] -> w49 mode=indexing
            n37 = Unbundle By Name(w69) -> ("offset"=w71:i32, "signal type 1"=w72:T30, "frequency 1"=w73:i32, "amplitude 1"=w74:dbl, "phase"=w75:dbl)
            n38 = call <vilib>:"Basic Function Generator.vi"("offset"=w71, "reset signal"=TRUE, "sampling info"=cluster{"Fs":dbl, "#s":dbl} {"Fs"=1000.0, "#s"=100.0} ("sampling info 4"), "signal type"=w72, "phase"=w75, "amplitude"=w74, "frequency"=w73) -> ("signal out"=w70:waveform(dbl))  [unwired: 2 in, 2 out]
          }
          n39 = property on="Tab Control" class="TabCtl (strict)"("Position"=T13 {"Left"=-1, "Top"=-1}) -> ()  [unwired: 2 in, 2 out]
          n40 = invoke class="VI" method="Default Vals.Reinit All"(reference=w58, error in=errorcluster {"status"=FALSE, "code"=0, "source"=""} ("error in (no error)")) -> (reference out=w56:refnum<vi>, error out=w57:errorcluster)  [unwired: 1 in, 1 out]
          n41 = call "FGV_EXIT.vi"("Function"=enum16{"Read", "Write"}."Write", "EXIT"=FALSE) -> ()  [unwired: 6 in, 1 out]
          n42 = Close Reference(reference=w56, error in (no error)=w57) -> (error out=w55:errorcluster)
        }
        frame #1 {
          w92 = "Listener" ("name (unnamed)")
          w95 = cluster{"State":T15, "Data":variant} {"State"=enum."Initalize", "Data"=variant}
          n43 = disable-structure shown="Enabled" {
            disable-tunnel: w89 -> [w109 w115]
            disable-tunnel: w88 -> [w108 _]
            disable-tunnel: [w101 w114] -> w87
            disable-tunnel: [w100 w110] -> w86
            disable-tunnel: w82 -> [_ w110]
            disable-tunnel: w85 -> [_ w113]
            disable-tunnel: [_ w112] -> w84
            frame Disabled {
              n44 = call <vilib>:"Open Config Data.vi"("error in (no error)"=w109, "configuration file path"=w108) -> ("error out"=w107:errorcluster, "refnum"=w106:T31)  [unwired: 7 in, 1 out]
              n45 = call-poly <vilib>:"Read Key.vi"("section"="DAQ Settings", "error in (no error)"=w107, "default value"="cDAQ2Mod1", "key"="DAQname", "refnum"=w106) -> ("error out"=w105:errorcluster, "value"=w100:string, "refnum out"=w104:T31)  [unwired: 3 in, 1 out]
              n46 = call <vilib>:"Close Config Data.vi"("error in (no error)"=w105, "refnum"=w104) -> ("error out"=w101:errorcluster)  [unwired: 8 in, 1 out]
            }
            frame Enabled {
              n47 = call "DAQ Assistant2"("data"=w113, "error in"=w115, "device name"=w110) -> ("error out"=w112:errorcluster)  [unwired: 15 in, 1 out]
              n48 = call <vilib>:"Clear Errors.vi"("error in (no error)"=w112) -> ("error out"=w114:errorcluster)  [unwired: 5 in, 1 out]
              n49 = Wait (ms)(milliseconds to wait=u32 50) -> ()  [unwired: 1 out]
            }
          }
          n50 = local write "Reply"(FALSE ("Reply")) -> ()
          n51 = Obtain Queue(name (unnamed)="VirbrationMain", element data type=w95, error in (no error)=w89) -> (queue out=w97:refnum<queue>, error out=w98:errorcluster)  [unwired: 2 in, 1 out]
          n52 = Not(x=w84) -> (.not. x?=→"Vibration State":bool)
          n53 = Enqueue Element(queue=w97, element=w95, error in (no error)=w98) -> (queue out=w94:refnum<queue>, error out=w93:errorcluster)  [unwired: 1 in, 1 out]
          n54 = Obtain Queue(name (unnamed)=w92, element data type=w92) -> (queue out=w91:refnum<queue>, error out=w90:errorcluster)  [unwired: 3 in, 1 out]
        }
        frame #2 {
          n55 = Merge Errors(w126, w127) -> (w118:errorcluster)
          n56 = property on="Project(Main)" class="Bool" props=["Visible"]() -> ()  [unwired: 2 in, 3 out]
          n57 = while {
            tunnel: w117 -> [w473]
            shift-right: [w464] -> _
            shift-left: T16 {"Channel Table"=[], "Model List name"=[], "Channel 1 Wave"={"t0"=timestamp(0 s since 1904-01-01), "dt"=1.0, "Y"=[]}, "Channel 2 Wave"={"t0"=timestamp(0 s since 1904-01-01), "dt"=1.0, "Y"=[]}, "Channel 3 Wave"={"t0"=timestamp(0 s since 1904-01-01), "dt"=1.0, "Y"=[]}, "Channel 4 Wave"={"t0"=timestamp(0 s since 1904-01-01), "dt"=1.0, "Y"=[]}, "Testing"=FALSE, "Set Time"=0, "Elapse Time"=0.0, "Channel 1"={" frequency 1"=20, "signal type 1"=enum."Sine Wave", "amplitude 1"=2.0, "offset"=0.0, "phase"=0.0}, "Channel 2"={" frequency 1"=20, "signal type 1"=enum."Sine Wave", "amplitude 1"=2.0, "offset"=0.0, "phase"=0.0}, "Channel 3"={" frequency 1"=20, "signal type 1"=enum."Sine Wave", "amplitude 1"=2.0, "offset"=0.0, "phase"=0.0}, "Channel 4"={" frequency 1"=20, "signal type 1"=enum."Sine Wave", "amplitude 1"=2.0, "offset"=0.0, "phase"=0.0}, "ModelList Num"=0, "Stop"=FALSE, "Button"=FALSE, "Button Time"=0, "Elapsed ?"=FALSE, "Channel 1 Wave (Main)"={"t0"=timestamp(0 s since 1904-01-01), "dt"=1.0, "Y"=[]}, "Channel 2 Wave (Main)"={"t0"=timestamp(0 s since 1904-01-01), "dt"=1.0, "Y"=[]}, "Channel 3 Wave (Main)"={"t0"=timestamp(0 s since 1904-01-01), "dt"=1.0, "Y"=[]}, "Channel 4 Wave (Main)"={"t0"=timestamp(0 s since 1904-01-01), "dt"=1.0, "Y"=[]}, "Project List name"=[], "Project Name"="", "Project Path"=path "", "ProjectList Num"=0, "Project Name(Set)"="", "Rate"=1000.0, "Channel 1 Sample"={"Sample Rate"=0.0, "Samples"=0.0}, "Channel 2 Sample"={"Sample Rate"=0.0, "Samples"=0.0}, "Channel 3 Sample"={"Sample Rate"=0.0, "Samples"=0.0}, "Channel 4 Sample"={"Sample Rate"=0.0, "Samples"=0.0}} -> [w467]
            tunnel: [w463] -> _
            shift-right: [w462] -> _
            shift-left: w126 -> [w472]
            tunnel: w121 -> [w455]
            stop <- w460 stop-if-true
            n58 = Dequeue Element(queue=w473, error in (no error)=w472) -> (queue out=w471:refnum<queue>, element=w469:cluster{"State":T15, "Data":variant}, error out=w470:errorcluster)  [unwired: 1 in, 1 out]
            n59 = Wait (ms)(milliseconds to wait=u32 1) -> ()  [unwired: 1 out]
            n60 = Unbundle(w469) -> ("State"=w468:T15, "Data"=w461:variant)
            n61 = case shown="\"Initalize\"" w468 {
              tunnel: w471 -> [w514 w653 w736 w760 w778 w796 w814 w832 w850 w868 w886 w888 w910 w971 w1023 w1067 w1078 w1083 w1118 w1129 w1146 w1174 w1203 w1232 w1261 w1290 w1319 w1337 w1350 w1403 w1414 w1425 w1437 w1500 w1503]
              tunnel: w470 -> [w508 w651 w738 w757 w775 w793 w809 w828 w846 w864 w882 w898 w907 w994 w1019 w1064 w1081 w1103 w1119 w1130 w1145 w1171 w1200 w1229 w1258 w1287 w1316 w1335 w1347 w1400 w1406 w1417 w1431 _ w1504]
              tunnel: w467 -> [w517 w648 w721 w753 w767 w784 w803 w822 w840 w858 w876 w892 w901 w990 w1021 w1058 w1070 w1099 w1111 w1126 w1147 w1169 w1198 w1227 w1256 w1285 w1314 w1332 w1344 w1398 w1410 w1421 w1433 w1499 w1505]
              tunnel: [w516 w649 w721 w755 w773 w791 w811 w829 w847 w865 w883 w899 w900 w989 w1020 w1057 w1077 w1106 w1115 w1125 w1147 w1168 w1197 w1226 w1255 w1284 w1313 w1331 w1343 w1397 w1409 w1420 w1434 w1499 w1505] -> w465
              tunnel: [w513 w652 w735 w758 w776 w794 w812 w830 w848 w866 w884 w888 w908 w970 w1022 w1066 w1078 w1101 w1117 w1128 w1146 w1173 w1202 w1231 w1260 w1289 w1318 w1336 w1349 w1402 w1413 w1424 w1436 w1500 w1503] -> w466
              tunnel: [w512 w650 w737 w759 w777 w795 w813 w831 w849 w867 w885 w889 w909 w972 w1018 w1065 w1076 w1102 w1116 w1127 w1145 w1170 w1199 w1228 w1257 w1286 w1315 w1334 w1346 w1399 w1411 w1422 w1435 w1494 w1504] -> w456
              tunnel: w461 -> [_ _ _ w756 w774 w792 w808 w827 w845 w863 w881 w897 w906 w995 _ _ w1080 _ _ _ _ _ _ _ _ _ _ _ _ _ w1407 w1418 _ w1497 _]
              tunnel: [_ _ _ _ _ _ _ _ _ _ _ _ _ _ _ _ _ _ _ _ _ _ _ _ _ _ _ _ _ _ _ _ _ _ w1502] -> w460
              tunnel: w455 -> [_ w640 _ _ _ _ _ _ _ _ _ _ _ _ _ _ _ _ _ _ _ _ _ _ _ _ _ _ _ _ _ _ _ w1498 _]
              frame "Initalize" {
                n62 = case shown="True" "SubUI" {
                  tunnel: [w534 w598] -> w518
                  tunnel: [w533 w597] -> w500
                  tunnel: [w532 w596] -> w511
                  tunnel: [w531 w595] -> w510
                  tunnel: [w530 w578] -> w509
                  tunnel: w508 -> [w529 w594]
                  tunnel: [w524 w590] -> w507
                  tunnel: [_ w575] -> w503
                  frame False {
                    w521 = TRUE ("Visible")
                    n63 = call <vilib>:"Application Directory.vi"() -> ("Application Directory"=w523:path)
                    n64 = property on="Project(Setting)" class="Bool"("Visible"=w521) -> ()  [unwired: 2 in, 2 out]
                    n65 = property on="Exit Button" class="Bool (strict)"("Visible"=w521) -> ()  [unwired: 2 in, 2 out]
                    n66 = Build Path(base path=w523, name or relative path="Vibration") -> (appended path=w527:path)
                    n67 = property on="Project(Main)" class="Bool"("Visible"=w521) -> ()  [unwired: 2 in, 2 out]
                    n68 = call <vilib>:"Check if File or Folder Exists.vi"("error in (no error)"=w529, "path"=w527) -> ("error out"=w528:errorcluster, "file or folder exists?"=w525:bool, "dup path"=w526:path)  [unwired: 7 in]
                    n69 = case shown="True" w525 {
                      tunnel: [_ w546] -> w534
                      tunnel: [w536 w545] -> w533
                      tunnel: [_ w543] -> w532
                      tunnel: [_ w542] -> w531
                      tunnel: [_ w541] -> w530
                      tunnel: w528 -> [w537 w539]
                      tunnel: w526 -> [w535 w538]
                      tunnel: [w535 w538] -> w524
                      frame False {
                        n70 = Create Folder(path (use dialog)=w535, error in=w537) -> (error out=w536:errorcluster)  [unwired: 1 in, 2 out]
                      }
                      frame True {
                        n71 = List Folder(path=w538, error in=w539) -> (folder names=w541:string[], error out=w544:errorcluster)  [unwired: 2 in, 2 out]
                        n72 = Empty Array?(array=w541) -> (empty?=w540:bool)
                        n73 = case shown="False" w540 {
                          tunnel: [w558 _] -> w546
                          tunnel: [w557 w570] -> w545
                          tunnel: w544 -> [w552 w570]
                          tunnel: w541 -> [w550 _]
                          tunnel: [w549 _] -> w543
                          tunnel: w538 -> [w548 _]
                          tunnel: [w547 _] -> w542
                          frame False {
                            w547 = 0
                            n74 = Index Array(array=w550, index=w547) -> (element=w549:string)
                            n75 = Build Path(base path=w548, name or relative path=w549) -> (appended path=w551:path)
                            n76 = Build Path(base path=w551, name or relative path="Channel Setting.dat") -> (appended path=w555:path)
                            n77 = call <vilib>:"Check if File or Folder Exists.vi"("error in (no error)"=w552, "path"=w555) -> ("error out"=w556:errorcluster, "file or folder exists?"=w554:bool, "dup path"=w553:path)  [unwired: 7 in]
                            n78 = case shown="True" w554 {
                              tunnel: [_ w564] -> w558
                              tunnel: [w560 w563] -> w557
                              tunnel: w556 -> [w560 w562]
                              tunnel: w553 -> [_ w561]
                              frame False {
                              }
                              frame True {
                                n79 = call-poly <vilib>:"Read From XML File.vi"("error in (no error)"=w562, "XML File Path"=w561) -> ("error out"=w565:errorcluster, "XML Elements"=w569:string)  [unwired: 7 in, 1 out]
                                n80 = Bundle("DataTable"=T1 [], "Item Names"=string[] []) -> (w566:T32)  [unwired: 1 in]
                                n81 = Unflatten From XML(xml string=w569, type=w566, error in (no error)=w565) -> (value=w564:T32, error out=w563:errorcluster)
                              }
                            }
                          }
                          frame True {
                          }
                        }
                      }
                    }
                  }
                  frame True {
                    w581 = FALSE ("Visible")
                    n82 = global read "Main Glb.vi" "System Path"() -> (w586:path)
                    n83 = global read "Main Glb.vi" "ProjectRef"() -> (w583:refnum<vi>)
                    n84 = property class="Str"(reference=w583) -> ("Value"=w589:string)  [unwired: 1 in, 2 out]
                    n85 = Build Path(base path=w586, name or relative path="Package") -> (appended path=w587:path)
                    n86 = Build Path(base path=w587, name or relative path=w589) -> (appended path=w588:path)
                    n87 = property on="Project(Setting)" class="Bool"("Visible"=w581) -> ()  [unwired: 2 in, 2 out]
                    n88 = property on="Exit Button" class="Bool (strict)"("Visible"=w581) -> ()  [unwired: 2 in, 2 out]
                    n89 = property on="Project(Main)" class="Bool"("Visible"=w581) -> ()  [unwired: 2 in, 2 out]
                    n90 = Build Path(base path=w588, name or relative path="Vibration") -> (appended path=w582:path)
                    n91 = property on="Tab Control" class="TabCtl (strict)"("Value"=2) -> ()  [unwired: 2 in, 2 out]
                    n92 = call <vilib>:"Check if File or Folder Exists.vi"("error in (no error)"=w594, "path"=w582) -> ("error out"=w593:errorcluster, "file or folder exists?"=w591:bool, "dup path"=w592:path)  [unwired: 7 in]
                    n93 = case shown="True" w591 {
                      tunnel: [_ w614] -> w598
                      tunnel: [w601 w613] -> w597
                      tunnel: [_ w611] -> w596
                      tunnel: [_ w610] -> w595
                      tunnel: [_ w609] -> w578
                      tunnel: w593 -> [w604 w608]
                      tunnel: w592 -> [w602 w607]
                      tunnel: [w602 w607] -> w590
                      tunnel: w582 -> [_ w606]
                      frame False {
                        n94 = Create Folder(path (use dialog)=w602, error in=w604) -> (error out=w603:errorcluster)  [unwired: 1 in, 2 out]
                        n95 = call <vilib>:"Clear Errors.vi"("error in (no error)"=w603) -> ("error out"=w601:errorcluster)  [unwired: 5 in, 1 out]
                      }
                      frame True {
                        n96 = List Folder(path=w607, error in=w608) -> (folder names=w609:string[], error out=w612:errorcluster)  [unwired: 2 in, 2 out]
                        n97 = case shown="False" FALSE {
                          tunnel: [w625 _] -> w614
                          tunnel: [w624 w637] -> w613
                          tunnel: w612 -> [w619 w637]
                          tunnel: w609 -> [w618 _]
                          tunnel: [w617 _] -> w611
                          tunnel: [w616 _] -> w610
                          tunnel: w606 -> [w615 _]
                          frame False {
                            w616 = 0
                            n98 = Index Array(array=w618, index=w616) -> (element=w617:string)
                            n99 = Build Path(base path=w615, name or relative path="Channel Setting.dat") -> (appended path=w622:path)
                            n100 = call <vilib>:"Check if File or Folder Exists.vi"("error in (no error)"=w619, "path"=w622) -> ("error out"=w623:errorcluster, "file or folder exists?"=w621:bool, "dup path"=w620:path)  [unwired: 7 in]
                            n101 = case shown="True" w621 {
                              tunnel: [_ w631] -> w625
                              tunnel: [w627 w630] -> w624
                              tunnel: w623 -> [w627 w629]
                              tunnel: w620 -> [_ w628]
                              frame False {
                              }
                              frame True {
                                n102 = call-poly <vilib>:"Read From XML File.vi"("error in (no error)"=w629, "XML File Path"=w628) -> ("error out"=w632:errorcluster, "XML Elements"=w636:string)  [unwired: 7 in, 1 out]
                                n103 = Bundle("DataTable"=T1 [], "Item Names"=string[] []) -> (w633:T32)  [unwired: 1 in]
                                n104 = Unflatten From XML(xml string=w636, type=w633, error in (no error)=w632) -> (value=w631:T32, error out=w630:errorcluster)
                              }
                            }
                          }
                          frame True {
                          }
                        }
                      }
                    }
                    n105 = property on="SequenceList" class="LstBox (strict)"("Item Names"=string[] []) -> ()  [unwired: 2 in, 2 out]
                    n106 = call "Virbration ListFGV.vi"("Action"=T21."Initial") -> ("error out"=w575:errorcluster)  [unwired: 12 in, 2 out]
                    n107 = call "Virbration SequenceFGV.vi"("Action"=T22."Initial", "error in"=w575) -> ("error out"=w573:errorcluster)  [unwired: 11 in, 2 out]
                    n108 = call "Virbration SequenceFGV.vi"("Action"=T22."Load", "error in"=w573) -> ("VirbSeqDataList"=w572:T33)  [unwired: 11 in, 2 out]
                    n109 = for {
                      tunnel: w572 -> [w600] mode=indexing
                      tunnel: [w599] -> w571 mode=indexing
                      n110 = Unbundle By Name(w600) -> ("VirbSeqName"=w599:string)
                    }
                    n111 = property on="SequenceName" class="Ring (strict)"("Strings []"=w571) -> ()  [unwired: 2 in, 2 out]
                  }
                }
                n112 = Unbundle(w518) -> ("DataTable"=w515:T1, "Item Names"=w502:string[])
                n113 = flat-sequence {
                  tunnel: [w520] -> w501
                  tunnel: w500 -> [w520]
                  frame #0 {
                    n114 = global write "Panel RefGlb.vi" "Virbration load"(TRUE ("Virbration load")) -> ()
                  }
                }
                n115 = Bundle By Name(cluster=w517, "Channel Table"=w515, "Model List name"=w502, "Project Name"=w511, "ProjectList Num"=w510, "Project List name"=w509, "Project Path"=w507) -> (w516:T16)
                n116 = call "Virbration ListFGV.vi"("TableIn"=w502, "Action"=T21."WrteAll", "error in"=w503) -> ()  [unwired: 10 in, 3 out]
                n117 = Enqueue Element(queue=w514, element=cluster{"State":T15, "Data":variant} {"State"=enum."Update", "Data"=variant}, error in (no error)=w501) -> (queue out=w513:refnum<queue>, error out=w512:errorcluster)  [unwired: 1 in, 1 out]
              }
              frame "Idle", Default {
                n118 = Unbundle By Name(w648) -> ("Stop"=w645:bool, "Testing"=w641:bool, "Elapsed ?"=w644:bool)
                n119 = Not(x=w645) -> (.not. x?=w646:bool)
                n120 = Not(x=w644) -> (.not. x?=w642:bool)
                n121 = Compound Arithmetic op=AND(w646, w641, w642) -> (w643:bool)
                "Testing" <- w643
                "Running" <- w643
                n122 = Bundle By Name(cluster=w648, "Testing"=w643) -> (w647:T16)
                n123 = property on="Connect" class="Bool (strict)"() -> ("Value"=w639:bool)  [unwired: 2 in, 2 out]
                n124 = case shown="False" w643 {
                  tunnel: w653 -> [w663 w717]
                  tunnel: [w662 w716] -> w652
                  tunnel: w651 -> [w661 w714]
                  tunnel: [w660 w718] -> w650
                  tunnel: w647 -> [w665 w715]
                  tunnel: [w664 w715] -> w649
                  tunnel: w645 -> [w659 _]
                  tunnel: w642 -> [w658 _]
                  tunnel: w641 -> [w657 _]
                  tunnel: w640 -> [w656 _]
                  tunnel: w639 -> [w655 _]
                  tunnel: "Reply" -> [w654 _]
                  frame False {
                    n125 = case shown="False" w659 {
                      tunnel: w665 -> [w670 w711]
                      tunnel: [w669 w710] -> w664
                      tunnel: w663 -> [w676 w713]
                      tunnel: [w675 w713] -> w662
                      tunnel: w661 -> [w674 w712]
                      tunnel: [w673 w712] -> w660
                      tunnel: w658 -> [w671 _]
                      tunnel: w657 -> [w672 _]
                      tunnel: w656 -> [w668 _]
                      tunnel: w655 -> [w667 _]
                      tunnel: w654 -> [w666 _]
                      frame False {
                        n126 = case shown="False" w672 {
                          tunnel: w676 -> [w685 w704]
                          tunnel: [w684 w705] -> w675
                          tunnel: w674 -> [w686 w708]
                          tunnel: [w683 w708] -> w673
                          tunnel: w671 -> [w682 _]
                          tunnel: w670 -> [w681 w707]
                          tunnel: [w680 w707] -> w669
                          tunnel: w668 -> [w679 _]
                          tunnel: w667 -> [w678 _]
                          tunnel: w666 -> [w677 _]
                          frame False {
                            n127 = case shown="False" w682 {
                              tunnel: w686 -> [w695 w703]
                              tunnel: w685 -> [w694 w700]
                              tunnel: [w694 w699] -> w684
                              tunnel: [w695 w703] -> w683
                              tunnel: w681 -> [w693 w702]
                              tunnel: [w691 w702] -> w680
                              tunnel: w679 -> [w690 _]
                              tunnel: w678 -> [w689 _]
                              tunnel: w677 -> [w688 _]
                              frame False {
                                n128 = Bundle By Name(cluster=w693, "Elapsed ?"=FALSE) -> (w691:T16)
                                n129 = And(x=w689, y=w688) -> (x .and. y?=w687:bool)
                                n130 = case shown="True" w687 {
                                tunnel: w690 -> [_ w698]
                                frame False {
                                }
                                frame True {
                                n131 = local write "Reply"(FALSE ("Reply")) -> ()
                                n132 = Enqueue Element(queue=w698, element="ok") -> ()  [unwired: 2 in, 3 out]
                                }
                                }
                              }
                              frame True {
                                n133 = Enqueue Element(queue=w700, element=cluster{"State":T15, "Data":variant} {"State"=enum."Check Time", "Data"=variant}) -> (queue out=w699:refnum<queue>)  [unwired: 2 in, 2 out]
                              }
                            }
                          }
                          frame True {
                            n134 = Enqueue Element(queue=w704, element=cluster{"State":T15, "Data":variant} {"State"=enum."Check Time", "Data"=variant}) -> (queue out=w705:refnum<queue>)  [unwired: 2 in, 2 out]
                          }
                        }
                      }
                      frame True {
                        n135 = Bundle By Name(cluster=w711, "Stop"=FALSE) -> (w710:T16)
                      }
                    }
                  }
                  frame True {
                    n136 = Enqueue Element(queue=w717, element=cluster{"State":T15, "Data":variant} {"State"=enum."Check Time", "Data"=variant}, error in (no error)=w714) -> (queue out=w716:refnum<queue>, error out=w718:errorcluster)  [unwired: 1 in, 1 out]
                  }
                }
              }
              frame "Update" {
                n137 = Unbundle By Name(w721) -> ("ModelList Num"=w724:i32, "Project Name"=→"Current Project":string, "Elapse Time"=→"Test Time(s)":dbl, "Channel 1 Wave"=→"Channel 1 Wave":waveform(dbl), "Channel 2 Wave"=→"Channel 2 Wave":waveform(dbl), "Channel 3 Wave"=→"Channel 3 Wave":waveform(dbl), "Channel 4 Wave"=→"Channel 4 Wave":waveform(dbl), "Channel Table"=→"DataTable":T1, "Model List name"=w742:string[], "Channel 1"=w733:T23, "Channel 2"=w732:T23, "Channel 3"=w731:T23, "Channel 4"=w730:T23, "Set Time"=w729:i32, "Project List name"=w726:string[], "Project Name(Set)"=w725:string)
                n138 = property on="Model List" class="LstBox (strict)"("Item Names"=w742) -> ()  [unwired: 2 in, 2 out]
                n139 = property on="Channel 1" class="Clust (strict)"("Value"=w733) -> ()  [unwired: 2 in, 2 out]
                n140 = property on="Channel 2" class="Clust (strict)"("Value"=w732) -> ()  [unwired: 2 in, 2 out]
                n141 = property on="Channel 3" class="Clust (strict)"("Value"=w731) -> ()  [unwired: 2 in, 2 out]
                n142 = property on="Channel 4" class="Clust (strict)"("Value"=w730) -> ()  [unwired: 2 in, 2 out]
                n143 = property on="Time(ms)" class="DigNum (strict)"("Value"=w729) -> ()  [unwired: 2 in, 2 out]
                n144 = property on="Project List" class="LstBox (strict)"("Item Names"=w726) -> ()  [unwired: 2 in, 2 out]
                n145 = property on="Project Name" class="Str"("Value"=w725) -> ()  [unwired: 2 in, 2 out]
                n146 = property on="Model List" class="LstBox (strict)"("Value"=w724) -> ()  [unwired: 2 in, 2 out]
                n147 = Unbundle By Name(w721) -> ("Rate"=w720:dbl)
                n148 = property on="Sampling rate" class="DigNum (strict)"("Value"=w720) -> ()  [unwired: 2 in, 2 out]
                n149 = Enqueue Element(queue=w736, element=cluster{"State":T15, "Data":variant} {"State"=enum."Idle", "Data"=variant}, error in (no error)=w738) -> (queue out=w735:refnum<queue>, error out=w737:errorcluster)  [unwired: 1 in, 1 out]
              }
              frame "Channel1" {
                n150 = Variant To Data(error in=w757, type=T23 {" frequency 1"=20, "signal type 1"=enum."Sine Wave", "amplitude 1"=2.0, "offset"=0.0, "phase"=0.0} ("Channel 2"), Variant=w756) -> (data=w748:T23, error out=w746:errorcluster)
                n151 = Unbundle By Name(w753) -> ("Channel Table"=w751:T1, "ModelList Num"=w750:i32)
                n152 = Index Array(array=w751, index=w750) -> (element=w749:T34)
                n153 = Bundle By Name(cluster=w749, "Channel 1"=w748) -> (w747:T34)
                n154 = Replace Array Subset(array=w751, new element=w747, index=w750) -> (w752:T1)
                n155 = Bundle By Name(cluster=w753, "Channel 1"=w748, "Channel Table"=w752) -> (w755:T16)
                n156 = Bundle By Name(cluster=cluster{"State":T15, "Data":variant} {"State"=enum."Waveform", "Data"=variant} ("element"), "Data"=1) -> (w743:cluster{"State":T15, "Data":variant})
                n157 = Enqueue Element At Opposite End(queue=w760, element=w743, error in (no error)=w746) -> (queue out=w758:refnum<queue>, error out=w759:errorcluster)  [unwired: 1 in, 1 out]
              }
              frame "Channel2" {
                n158 = Unbundle By Name(w767) -> ("Channel Table"=w771:T1, "ModelList Num"=w770:i32)
                n159 = Variant To Data(error in=w775, type=T23 {" frequency 1"=20, "signal type 1"=enum."Sine Wave", "amplitude 1"=2.0, "offset"=0.0, "phase"=0.0} ("Channel 2"), Variant=w774) -> (data=w766:T23, error out=w764:errorcluster)
                n160 = Index Array(array=w771, index=w770) -> (element=w769:T34)
                n161 = Bundle By Name(cluster=w769, "Channel 2"=w766) -> (w768:T34)
                n162 = Replace Array Subset(array=w771, new element=w768, index=w770) -> (w765:T1)
                n163 = Bundle By Name(cluster=w767, "Channel 2"=w766, "Channel Table"=w765) -> (w773:T16)
                n164 = Bundle By Name(cluster=cluster{"State":T15, "Data":variant} {"State"=enum."Waveform", "Data"=variant} ("element"), "Data"=2) -> (w761:cluster{"State":T15, "Data":variant})
                n165 = Enqueue Element At Opposite End(queue=w778, element=w761, error in (no error)=w764) -> (queue out=w776:refnum<queue>, error out=w777:errorcluster)  [unwired: 1 in, 1 out]
              }
              frame "Channel3" {
                n166 = Unbundle By Name(w784) -> ("Channel Table"=w789:T1, "ModelList Num"=w788:i32)
                n167 = Variant To Data(error in=w793, type=T23 {" frequency 1"=20, "signal type 1"=enum."Sine Wave", "amplitude 1"=2.0, "offset"=0.0, "phase"=0.0} ("Channel 2"), Variant=w792) -> (data=w785:T23, error out=w782:errorcluster)
                n168 = Index Array(array=w789, index=w788) -> (element=w787:T34)
                n169 = Bundle By Name(cluster=w787, "Channel 3"=w785) -> (w786:T34)
                n170 = Replace Array Subset(array=w789, new element=w786, index=w788) -> (w783:T1)
                n171 = Bundle By Name(cluster=w784, "Channel 3"=w785, "Channel Table"=w783) -> (w791:T16)
                n172 = Bundle By Name(cluster=cluster{"State":T15, "Data":variant} {"State"=enum."Waveform", "Data"=variant} ("element"), "Data"=3) -> (w780:cluster{"State":T15, "Data":variant})
                n173 = Enqueue Element At Opposite End(queue=w796, element=w780, error in (no error)=w782) -> (queue out=w794:refnum<queue>, error out=w795:errorcluster)  [unwired: 1 in, 1 out]
              }
              frame "Channel4" {
                n174 = Unbundle By Name(w803) -> ("Channel Table"=w807:T1, "ModelList Num"=w806:i32)
                n175 = Variant To Data(error in=w809, type=T23 {" frequency 1"=20, "signal type 1"=enum."Sine Wave", "amplitude 1"=2.0, "offset"=0.0, "phase"=0.0} ("Channel 2"), Variant=w808) -> (data=w802:T23, error out=w800:errorcluster)
                n176 = Index Array(array=w807, index=w806) -> (element=w805:T34)
                n177 = Bundle By Name(cluster=w805, "Channel 4"=w802) -> (w804:T34)
                n178 = Replace Array Subset(array=w807, new element=w804, index=w806) -> (w801:T1)
                n179 = Bundle By Name(cluster=cluster{"State":T15, "Data":variant} {"State"=enum."Waveform", "Data"=variant} ("element"), "Data"=4) -> (w797:cluster{"State":T15, "Data":variant})
                n180 = Bundle By Name(cluster=w803, "Channel 4"=w802, "Channel Table"=w801) -> (w811:T16)
                n181 = Enqueue Element At Opposite End(queue=w814, element=w797, error in (no error)=w800) -> (queue out=w812:refnum<queue>, error out=w813:errorcluster)  [unwired: 1 in, 1 out]
              }
              frame "Channel1 Sample" {
                n182 = Unbundle By Name(w822) -> ("Channel Table"=w826:T1, "ModelList Num"=w825:i32)
                n183 = Variant To Data(error in=w828, type=cluster{"Sample Rate":dbl, "Samples":dbl} {"Sample Rate"=0.0, "Samples"=0.0} ("Channel 4 Sample 2"), Variant=w827) -> (data=w821:cluster{"Sample Rate":dbl, "Samples":dbl}, error out=w818:errorcluster)
                n184 = Index Array(array=w826, index=w825) -> (element=w824:T34)
                n185 = Bundle By Name(cluster=w824, "Channel 1 Sample"=w821) -> (w823:T34)
                n186 = Replace Array Subset(array=w826, new element=w823, index=w825) -> (w820:T1)
                n187 = Bundle By Name(cluster=cluster{"State":T15, "Data":variant} {"State"=enum."Waveform", "Data"=variant} ("element"), "Data"=1) -> (w815:cluster{"State":T15, "Data":variant})
                n188 = Bundle By Name(cluster=w822, "Channel 1 Sample"=w821, "Channel Table"=w820) -> (w829:T16)
                n189 = Enqueue Element At Opposite End(queue=w832, element=w815, error in (no error)=w818) -> (queue out=w830:refnum<queue>, error out=w831:errorcluster)  [unwired: 1 in, 1 out]
              }
              frame "Channel2 Sample" {
                n190 = Unbundle By Name(w840) -> ("Channel Table"=w844:T1, "ModelList Num"=w843:i32)
                n191 = Variant To Data(error in=w846, type=cluster{"Sample Rate":dbl, "Samples":dbl} {"Sample Rate"=0.0, "Samples"=0.0} ("Channel 4 Sample 2"), Variant=w845) -> (data=w839:cluster{"Sample Rate":dbl, "Samples":dbl}, error out=w836:errorcluster)
                n192 = Index Array(array=w844, index=w843) -> (element=w842:T34)
                n193 = Bundle By Name(cluster=w842, "Channel 2 Sample"=w839) -> (w841:T34)
                n194 = Replace Array Subset(array=w844, new element=w841, index=w843) -> (w838:T1)
                n195 = Bundle By Name(cluster=cluster{"State":T15, "Data":variant} {"State"=enum."Waveform", "Data"=variant} ("element"), "Data"=2) -> (w833:cluster{"State":T15, "Data":variant})
                n196 = Bundle By Name(cluster=w840, "Channel 2 Sample"=w839, "Channel Table"=w838) -> (w847:T16)
                n197 = Enqueue Element At Opposite End(queue=w850, element=w833, error in (no error)=w836) -> (queue out=w848:refnum<queue>, error out=w849:errorcluster)  [unwired: 1 in, 1 out]
              }
              frame "Channel3 Sample" {
                n198 = Unbundle By Name(w858) -> ("Channel Table"=w862:T1, "ModelList Num"=w861:i32)
                n199 = Variant To Data(error in=w864, type=cluster{"Sample Rate":dbl, "Samples":dbl} {"Sample Rate"=0.0, "Samples"=0.0} ("Channel 4 Sample 2"), Variant=w863) -> (data=w857:cluster{"Sample Rate":dbl, "Samples":dbl}, error out=w854:errorcluster)
                n200 = Index Array(array=w862, index=w861) -> (element=w860:T34)
                n201 = Bundle By Name(cluster=w860, "Channel 3 Sample"=w857) -> (w859:T34)
                n202 = Replace Array Subset(array=w862, new element=w859, index=w861) -> (w856:T1)
                n203 = Bundle By Name(cluster=cluster{"State":T15, "Data":variant} {"State"=enum."Waveform", "Data"=variant} ("element"), "Data"=3) -> (w851:cluster{"State":T15, "Data":variant})
                n204 = Bundle By Name(cluster=w858, "Channel 3 Sample"=w857, "Channel Table"=w856) -> (w865:T16)
                n205 = Enqueue Element At Opposite End(queue=w868, element=w851, error in (no error)=w854) -> (queue out=w866:refnum<queue>, error out=w867:errorcluster)  [unwired: 1 in, 1 out]
              }
              frame "Channel4 Sample" {
                n206 = Unbundle By Name(w876) -> ("Channel Table"=w880:T1, "ModelList Num"=w879:i32)
                n207 = Variant To Data(error in=w882, type=cluster{"Sample Rate":dbl, "Samples":dbl} {"Sample Rate"=0.0, "Samples"=0.0} ("Channel 4 Sample 2"), Variant=w881) -> (data=w875:cluster{"Sample Rate":dbl, "Samples":dbl}, error out=w872:errorcluster)
                n208 = Index Array(array=w880, index=w879) -> (element=w878:T34)
                n209 = Bundle By Name(cluster=w878, "Channel 4 Sample"=w875) -> (w877:T34)
                n210 = Replace Array Subset(array=w880, new element=w877, index=w879) -> (w874:T1)
                n211 = Bundle By Name(cluster=cluster{"State":T15, "Data":variant} {"State"=enum."Waveform", "Data"=variant} ("element"), "Data"=4) -> (w869:cluster{"State":T15, "Data":variant})
                n212 = Bundle By Name(cluster=w876, "Channel 4 Sample"=w875, "Channel Table"=w874) -> (w883:T16)
                n213 = Enqueue Element At Opposite End(queue=w886, element=w869, error in (no error)=w872) -> (queue out=w884:refnum<queue>, error out=w885:errorcluster)  [unwired: 1 in, 1 out]
              }
              frame "DAQ Rate" {
                n214 = Unbundle By Name(w892) -> ("Channel Table"=w896:T1, "ModelList Num"=w895:i32)
                n215 = Variant To Data(error in=w898, type=0.0 ("Samples"), Variant=w897) -> (data=w891:dbl, error out=w889:errorcluster)
                n216 = Index Array(array=w896, index=w895) -> (element=w894:T34)
                n217 = Bundle By Name(cluster=w894, "Rate"=w891) -> (w893:T34)
                n218 = Replace Array Subset(array=w896, new element=w893, index=w895) -> (w890:T1)
                n219 = Bundle By Name(cluster=w892, "Rate"=w891, "Channel Table"=w890) -> (w899:T16)
              }
              frame "Waveform" {
                n220 = Variant To Data(error in=w907, type=0, Variant=w906) -> (data=w902:i32, error out=w905:errorcluster)
                n221 = case shown="2" w902 {
                  tunnel: w901 -> [_ w914 w925 w936 w947]
                  tunnel: w901 -> [w911 w922 w933 w944 w955]
                  tunnel: [w911 w921 w932 w943 w954] -> w900
                  frame 0, Default {
                  }
                  frame 1 {
                    n222 = Unbundle By Name(w914) -> ("Channel 1.offset"=w920:dbl, "Channel 1.signal type 1"=w919:T30, "Channel 1.frequency 1"=w918:u32, "Channel 1.amplitude 1"=w917:dbl, "Channel 1.phase"=w916:dbl)  [unwired: 1 out]
                    n223 = call <vilib>:"Basic Function Generator.vi"("offset"=w920, "reset signal"=TRUE, "sampling info"=cluster{"Fs":dbl, "#s":dbl} {"Fs"=1000.0, "#s"=100.0}, "signal type"=w919, "phase"=w916, "amplitude"=w917, "frequency"=w918) -> ("signal out"=w913:waveform(dbl))  [unwired: 2 in, 2 out]
                    n224 = Bundle By Name(cluster=w922, "Channel 1 Wave"=w913) -> (w921:T16)
                  }
                  frame 2 {
                    n225 = Unbundle By Name(w925) -> ("Channel 2.offset"=w931:dbl, "Channel 2.signal type 1"=w930:T30, "Channel 2.frequency 1"=w929:u32, "Channel 2.amplitude 1"=w928:dbl, "Channel 2.phase"=w927:dbl)  [unwired: 1 out]
                    n226 = call <vilib>:"Basic Function Generator.vi"("offset"=w931, "reset signal"=TRUE, "sampling info"=cluster{"Fs":dbl, "#s":dbl} {"Fs"=1000.0, "#s"=100.0}, "signal type"=w930, "phase"=w927, "amplitude"=w928, "frequency"=w929) -> ("signal out"=w924:waveform(dbl))  [unwired: 2 in, 2 out]
                    n227 = Bundle By Name(cluster=w933, "Channel 2 Wave"=w924) -> (w932:T16)
                  }
                  frame 3 {
                    n228 = Unbundle By Name(w936) -> ("Channel 3.offset"=w942:dbl, "Channel 3.signal type 1"=w941:T30, "Channel 3.frequency 1"=w940:u32, "Channel 3.amplitude 1"=w939:dbl, "Channel 3.phase"=w938:dbl)  [unwired: 1 out]
                    n229 = call <vilib>:"Basic Function Generator.vi"("offset"=w942, "reset signal"=TRUE, "sampling info"=cluster{"Fs":dbl, "#s":dbl} {"Fs"=1000.0, "#s"=100.0}, "signal type"=w941, "phase"=w938, "amplitude"=w939, "frequency"=w940) -> ("signal out"=w935:waveform(dbl))  [unwired: 2 in, 2 out]
                    n230 = Bundle By Name(cluster=w944, "Channel 3 Wave"=w935) -> (w943:T16)
                  }
                  frame 4 {
                    n231 = Unbundle By Name(w947) -> ("Channel 4.offset"=w953:dbl, "Channel 4.signal type 1"=w952:T30, "Channel 4.frequency 1"=w951:u32, "Channel 4.amplitude 1"=w950:dbl, "Channel 4.phase"=w949:dbl)  [unwired: 1 out]
                    n232 = call <vilib>:"Basic Function Generator.vi"("offset"=w953, "reset signal"=TRUE, "sampling info"=cluster{"Fs":dbl, "#s":dbl} {"Fs"=1000.0, "#s"=100.0}, "signal type"=w952, "phase"=w949, "amplitude"=w950, "frequency"=w951) -> ("signal out"=w946:waveform(dbl))  [unwired: 2 in, 2 out]
                    n233 = Bundle By Name(cluster=w955, "Channel 4 Wave"=w946) -> (w954:T16)
                  }
                }
                n234 = Enqueue Element At Opposite End(queue=w910, element=cluster{"State":T15, "Data":variant} {"State"=enum."Update", "Data"=variant}, error in (no error)=w905) -> (queue out=w908:refnum<queue>, error out=w909:errorcluster)  [unwired: 1 in, 1 out]
              }
              frame "ModelList" {
                n235 = Unbundle By Name(w990) -> ("Channel Table"=w992:T1)
                n236 = Variant To Data(error in=w994, type=0, Variant=w995) -> (data=w968:i32, error out=w973:errorcluster)
                n237 = Index Array(array=w992, index=w968) -> (element=w991:T34)
                n238 = Unbundle(w991) -> ("Channel 1"=w987:T23, "Channel 2"=w986:T23, "Channel 3"=w985:T23, "Channel 4"=w984:T23, "Time(ms)"=w988:i32, "Rate"=w961:dbl, "Channel 1 Sample"=w966:cluster{"Sample Rate":dbl, "Samples":dbl}, "Channel 2 Sample"=w965:cluster{"Sample Rate":dbl, "Samples":dbl}, "Channel 3 Sample"=w964:cluster{"Sample Rate":dbl, "Samples":dbl}, "Channel 4 Sample"=w963:cluster{"Sample Rate":dbl, "Samples":dbl})
                n239 = Build Array(w966, w965, w964, w963) -> (w962:cluster{"Sample Rate":dbl, "Samples":dbl}[])
                n240 = Build Array(w987, w986, w985, w984) -> (w983:T35)
                n241 = for {
                  tunnel: w983 -> [w998] mode=indexing
                  tunnel: [w999] -> w967 mode=indexing
                  tunnel: [w998] -> w982 mode=indexing
                  tunnel: w962 -> [w997] mode=indexing
                  tunnel: [w997] -> w960 mode=indexing
                  n242 = Unbundle By Name(w998) -> ("offset"=w1000:dbl, "signal type 1"=w1001:T30, "frequency 1"=w1002:u32, "amplitude 1"=w1003:dbl, "phase"=w1004:dbl)
                  n243 = call <vilib>:"Basic Function Generator.vi"("offset"=w1000, "reset signal"=TRUE, "sampling info"=cluster{"Fs":dbl, "#s":dbl} {"Fs"=1000.0, "#s"=100.0}, "signal type"=w1001, "phase"=w1004, "amplitude"=w1003, "frequency"=w1002) -> ("signal out"=w999:waveform(dbl))  [unwired: 2 in, 2 out]
                }
                n244 = Index Array(array=w960) -> (element #1=w959:cluster{"Sample Rate":dbl, "Samples":dbl}, element #2=w958:cluster{"Sample Rate":dbl, "Samples":dbl}, element #3=w957:cluster{"Sample Rate":dbl, "Samples":dbl}, element #4=w956:cluster{"Sample Rate":dbl, "Samples":dbl})  [unwired: 4 in]
                n245 = Index Array(array=w982) -> (element #1=w981:T23, element #2=w976:T23, element #3=w975:T23, element #4=w974:T23)  [unwired: 4 in]
                n246 = Index Array(array=w967) -> (element #1=w980:waveform(dbl), element #2=w979:waveform(dbl), element #3=w978:waveform(dbl), element #4=w977:waveform(dbl))  [unwired: 4 in]
                n247 = Bundle By Name(cluster=w990, "Channel 1 Wave"=w980, "Channel 2 Wave"=w979, "Channel 3 Wave"=w978, "Channel 4 Wave"=w977, "Channel 1"=w981, "Channel 2"=w976, "Channel 3"=w975, "Channel 4"=w974, "Channel 1 Sample"=w959, "Channel 2 Sample"=w958, "Channel 3 Sample"=w957, "Channel 4 Sample"=w956, "Set Time"=w988, "Rate"=w961, "ModelList Num"=w968) -> (w989:T16)
                n248 = Enqueue Element At Opposite End(queue=w971, element=cluster{"State":T15, "Data":variant} {"State"=enum."Update", "Data"=variant}, error in (no error)=w973) -> (queue out=w970:refnum<queue>, error out=w972:errorcluster)  [unwired: 1 in, 1 out]
              }
              frame "Add" {
                n249 = Unbundle By Name(w1021) -> ("Channel Table"=w1008:T1, "Model List name"=w1009:string[])
                n250 = call <vilib>:"Trim Whitespace.vi"("string"="Model Name") -> ("trimmed string"=w1010:string)  [unwired: 1 in]
                n251 = To Upper Case(1:w1009) -> (0:w1013:string[])
                n252 = To Upper Case(1:w1010) -> (0:w1011:string)
                n253 = Search 1D Array(1D array=w1013, element=w1011) -> (index of element=w1016:i32)  [unwired: 1 in]
                n254 = Empty String/Path?(string/path=w1010) -> (empty?=w1014:bool)
                n255 = Greater Or Equal To 0?(x=w1016) -> (x >= 0?=w1015:bool)
                n256 = case shown="False" w1014 {
                  tunnel: w1015 -> [w1031 _]
                  tunnel: w1010 -> [w1030 _]
                  tunnel: [w1029 _] -> w1017
                  tunnel: w1009 -> [w1028 w1042]
                  tunnel: [w1027 w1042] -> w1006
                  tunnel: w1008 -> [w1026 w1041]
                  tunnel: [w1025 w1041] -> w1007
                  frame False {
                    n257 = case shown="False" w1031 {
                      tunnel: w1030 -> [w1036 _]
                      tunnel: ["" _] -> w1029
                      tunnel: w1028 -> [w1037 w1040]
                      tunnel: [w1035 w1040] -> w1027
                      tunnel: w1026 -> [w1034 w1039]
                      tunnel: [w1033 w1039] -> w1025
                      frame False {
                        n258 = Build Array (concatenate)(w1037, w1036) -> (w1035:string[])
                        n259 = Build Array (concatenate)(w1034, T1 [{"Channel 1"={" frequency 1"=0, "signal type 1"=enum."Sine Wave", "amplitude 1"=0.0, "offset"=0.0, "phase"=0.0}, "Channel 2"={" frequency 1"=0, "signal type 1"=enum."Sine Wave", "amplitude 1"=0.0, "offset"=0.0, "phase"=0.0}, "Channel 3"={" frequency 1"=0, "signal type 1"=enum."Sine Wave", "amplitude 1"=0.0, "offset"=0.0, "phase"=0.0}, "Channel 4"={" frequency 1"=0, "signal type 1"=enum."Sine Wave", "amplitude 1"=0.0, "offset"=0.0, "phase"=0.0}, "Time(ms)"=0, "Rate"=1000.0, "Channel 1 Sample"={"Sample Rate"=0.0, "Samples"=0.0}, "Channel 2 Sample"={"Sample Rate"=0.0, "Samples"=0.0}, "Channel 3 Sample"={"Sample Rate"=0.0, "Samples"=0.0}, "Channel 4 Sample"={"Sample Rate"=0.0, "Samples"=0.0}}] ("element")) -> (w1033:T1)
                      }
                      frame True {
                      }
                    }
                  }
                  frame True {
                  }
                }
                n260 = property on="Model Name" class="Str"("Value"=w1017) -> ()  [unwired: 2 in, 2 out]
                n261 = Bundle By Name(cluster=w1021, "Channel Table"=w1007, "Model List name"=w1006) -> (w1020:T16)
                n262 = disable-structure shown="Disabled" {
                  frame Disabled {
                    n263 = Array Size() -> (size(s)=w1047:i32)  [unwired: 1 in]
                    n264 = Decrement(x=w1047) -> (x-1=w1043:i32)
                    n265 = Index Array(index=w1043) -> ()  [unwired: 1 in, 1 out]
                    n266 = Match Pattern(regular expression="Model") -> (after substring=w1045:string)  [unwired: 2 in, 3 out]
                    n267 = Decimal String To Number(string=w1045) -> (number=w1048:i32)  [unwired: 2 in, 1 out]
                    n268 = Increment(x=w1048) -> (x+1=w1049:i32)
                    n269 = Format Into String(format string="Model%d", w1049) -> ()  [unwired: 2 in, 2 out]
                  }
                  frame Enabled {
                  }
                }
                n270 = Enqueue Element At Opposite End(queue=w1023, element=cluster{"State":T15, "Data":variant} {"State"=enum."Update", "Data"=variant}, error in (no error)=w1019) -> (queue out=w1022:refnum<queue>, error out=w1018:errorcluster)  [unwired: 1 in, 1 out]
              }
              frame "Remove" {
                w1051 = cluster{"Sample Rate":dbl, "Samples":dbl} {"Sample Rate"=0.0, "Samples"=0.0} ("Channel 1 Sample")
                w1054 = T23 {" frequency 1"=0, "signal type 1"=enum."Sine Wave", "amplitude 1"=0.0, "offset"=0.0, "phase"=0.0} ("Channel 1")
                w1055 = waveform(dbl) {"t0"=timestamp(0 s since 1904-01-01), "dt"=1.0, "Y"=[]} ("Channel 1 Wave")
                n271 = Unbundle By Name(w1058) -> ("Channel Table"=w1061:T1, "ModelList Num"=w1059:i32, "Model List name"=w1060:string[])
                n272 = Delete From Array(array=w1061, length=1, index=w1059) -> (array with subset deleted=w1056:T1)  [unwired: 1 out]
                n273 = Delete From Array(array=w1060, length=1, index=w1059) -> (array with subset deleted=w1050:string[])  [unwired: 1 out]
                n274 = Bundle By Name(cluster=w1058, "Channel 1 Sample"=w1051, "Channel 2 Sample"=w1051, "Channel 3 Sample"=w1051, "Channel 4 Sample"=w1051, "Rate"=0.0, "Set Time"=0, "Channel 1 Wave"=w1055, "Channel 2 Wave"=w1055, "Channel 3 Wave"=w1055, "Channel 4 Wave"=w1055, "Channel 1"=w1054, "Channel 2"=w1054, "Channel 3"=w1054, "Channel 4"=w1054, "Channel Table"=w1056, "Model List name"=w1050) -> (w1057:T16)
                n275 = Enqueue Element At Opposite End(queue=w1067, element=cluster{"State":T15, "Data":variant} {"State"=enum."Update", "Data"=variant}, error in (no error)=w1064) -> (queue out=w1066:refnum<queue>, error out=w1065:errorcluster)  [unwired: 1 in, 1 out]
              }
              frame "Set Time" {
                n276 = Unbundle By Name(w1070) -> ("Channel Table"=w1075:T1, "ModelList Num"=w1074:i32)
                n277 = Variant To Data(error in=w1081, type=0, Variant=w1080) -> (data=w1071:i32, error out=w1076:errorcluster)
                n278 = Index Array(array=w1075, index=w1074) -> (element=w1073:T34)
                n279 = Bundle By Name(cluster=w1073, "Time(ms)"=w1071) -> (w1072:T34)
                n280 = Replace Array Subset(array=w1075, new element=w1072, index=w1074) -> (w1069:T1)
                n281 = Bundle By Name(cluster=w1070, "Set Time"=w1071, "Channel Table"=w1069) -> (w1077:T16)
              }
              frame "Test" {
                n282 = Flush Queue(queue=w1083) -> (queue out=w1082:refnum<queue>)  [unwired: 1 in, 2 out]
                n283 = Unbundle By Name(w1099) -> ("Channel 1 Wave"=w1098:waveform(dbl), "Channel 2 Wave"=w1097:waveform(dbl), "Channel 3 Wave"=w1096:waveform(dbl), "Channel 4 Wave"=w1095:waveform(dbl), "Rate"=w1089:dbl)
                n284 = Build Array(w1098, w1097, w1096, w1095) -> (w1093:waveform(dbl)[])
                n285 = property on="Test Setting" class="Arr (strict)"("Value"=w1093) -> (error out=w1090:errorcluster)  [unwired: 2 in, 1 out]
                n286 = property on="Sampling rate" class="DigNum (strict)"(error in=w1090, "Value"=w1089) -> (error out=w1087:errorcluster)  [unwired: 1 in, 1 out]
                n287 = Enqueue Element(queue=w1082, element=cluster{"State":T15, "Data":variant} {"State"=enum."Start Time", "Data"=variant}, error in (no error)=w1103) -> (queue out=w1101:refnum<queue>, error out=w1102:errorcluster)  [unwired: 1 in, 1 out]
                n288 = property on="Test Time(s)" class="DigNum (strict)"(error in=w1087, "Value"=0.0 ("Test Time(s)")) -> (error out=w1086:errorcluster)  [unwired: 1 in, 1 out]
                n289 = property on="Test State" class="Enum (strict)"(error in=w1086, "Value"=Test_State."Normal" ("Test State")) -> (error out=w1091:errorcluster)  [unwired: 1 in, 1 out]
                n290 = property on="Testing?" class="Bool (strict)"(error in=w1091, "Value"=TRUE ("Testing?")) -> (error out=w1085:errorcluster)  [unwired: 1 in, 1 out]
                n291 = call "Wait t.vi"("error in"=w1085, "wait(ms)"=u32 50) -> ()  [unwired: 9 in, 1 out]
                n292 = Bundle By Name(cluster=w1099, "Button"=FALSE, "Testing"=TRUE) -> (w1106:T16)
              }
              frame "Start Time" {
                n293 = Unbundle By Name(w1111) -> ("Button Time"=w1109:i32, "Button"=w1110:bool, "Set Time"=w1108:i32)
                n294 = Select(t=w1109, s=w1110, f=w1108) -> (s? t:f=w1107:i32)
                n295 = call "FGV_Timer.vi"("State"=Timer_State."Start", "error in (no error)"=w1119, "Set Time"=w1107) -> ("error out"=w1113:errorcluster)  [unwired: 6 in, 2 out]
                n296 = Bundle By Name(cluster=w1111, "Elapse Time"=0.0) -> (w1115:T16)
                n297 = Enqueue Element(queue=w1118, element=cluster{"State":T15, "Data":variant} {"State"=enum."Check Time", "Data"=variant}, error in (no error)=w1113) -> (queue out=w1117:refnum<queue>, error out=w1116:errorcluster)  [unwired: 1 in, 1 out]
              }
              frame "Check Time" {
                n298 = call "FGV_Timer.vi"("State"=Timer_State."Check", "error in (no error)"=w1130) -> ("error out"=w1124:errorcluster, "Elapsed Time"=w1122:dbl, "Elapsed ?"=w1121:bool)  [unwired: 7 in]
                n299 = global write "GBV_Ref.vi" "Stop"(w1121) -> ()
                n300 = case shown="True" w1121 {
                  frame False {
                  }
                  frame True {
                    n301 = property on="Testing?" class="Bool (strict)"("Value"=FALSE ("Testing?")) -> ()  [unwired: 2 in, 2 out]
                  }
                }
                n302 = Bundle By Name(cluster=w1126, "Elapsed ?"=w1121, "Elapse Time"=w1122) -> (w1125:T16)
                n303 = Enqueue Element(queue=w1129, element=cluster{"State":T15, "Data":variant} {"State"=enum."Update", "Data"=variant}, error in (no error)=w1124) -> (queue out=w1128:refnum<queue>, error out=w1127:errorcluster)  [unwired: 1 in, 1 out]
              }
              frame "Save" {
                n304 = Unbundle By Name(w1147) -> ("Project Path"=w1143:path, "Project List name"=w1144:string[], "ProjectList Num"=w1139:i32, "Channel Table"=w1138:T1, "Model List name"=w1135:string[])
                n305 = local read "SubUI"() -> (w1137:bool)
                n306 = Index Array(array=w1144, index=w1139) -> (element=w1142:string)
                n307 = case shown="False" w1137 {
                  tunnel: w1143 -> [w1153 w1154]
                  tunnel: w1142 -> [w1152 _]
                  tunnel: [w1151 w1154] -> w1141
                  frame False {
                    n308 = Build Path(base path=w1153, name or relative path=w1152) -> (appended path=w1151:path)
                  }
                  frame True {
                  }
                }
                n309 = Bundle("Channel Table"=w1138, "Model List name"=w1135) -> (w1149:T36)  [unwired: 1 in]
                n310 = Flatten To XML(anything=w1149) -> (xml string=w1148:string)
                n311 = Build Path(base path=w1141, name or relative path="Channel Setting.dat") -> (appended path=w1150:path)
                n312 = call "Virbration ListFGV.vi"("TableIn"=w1135, "Action"=T21."WrteAll") -> ("error out"=w1133:errorcluster)  [unwired: 11 in, 2 out]
                n313 = call "Virbration SequenceFGV.vi"("Action"=T22."Save", "error in"=w1133) -> ()  [unwired: 11 in, 3 out]
                n314 = call-poly <vilib>:"Write to XML File.vi"("XML Input"=w1148, "XML File Path"=w1150) -> ()  [unwired: 7 in, 3 out]
              }
              frame "Frontward" {
                n315 = Unbundle(T25 {"Channel 1"={" frequency 1"=60, "signal type 1"=enum."Sine Wave", "amplitude 1"=0.6, "offset"=0.0, "phase"=0.0}, "Channel 2"={" frequency 1"=60, "signal type 1"=enum."Sine Wave", "amplitude 1"=0.0, "offset"=0.0, "phase"=0}, "Channel 3"={" frequency 1"=60, "signal type 1"=enum."Sine Wave", "amplitude 1"=0.0, "offset"=0.0, "phase"=0.0}, "Channel 4"={" frequency 1"=60, "signal type 1"=enum."Sine Wave", "amplitude 1"=0.0, "offset"=0.0, "phase"=0}} ("Front")) -> ("Channel 1"=w1159:T37, "Channel 2"=w1158:T38, "Channel 3"=w1157:T37, "Channel 4"=w1156:T38)
                n316 = Build Array(w1159, w1158, w1157, w1156) -> (w1167:T39)
                n317 = for {
                  tunnel: w1167 -> [w1175] mode=indexing
                  tunnel: [w1176] -> w1166 mode=indexing
                  n318 = Unbundle By Name(w1175) -> ("offset"=w1177:dbl, "signal type 1"=w1178:T30, "frequency 1"=w1179:i32, "amplitude 1"=w1180:dbl, "phase"=w1181:dbl)
                  n319 = call <vilib>:"Basic Function Generator.vi"("offset"=w1177, "reset signal"=TRUE, "sampling info"=cluster{"Fs":dbl, "#s":dbl} {"Fs"=1000.0, "#s"=100.0} ("sampling info 4"), "signal type"=w1178, "phase"=w1181, "amplitude"=w1180, "frequency"=w1179) -> ("signal out"=w1176:waveform(dbl))  [unwired: 2 in, 2 out]
                }
                n320 = Index Array(array=w1166) -> (element #1=w1165:waveform(dbl), element #2=w1164:waveform(dbl), element #3=w1163:waveform(dbl), element #4=w1162:waveform(dbl))  [unwired: 4 in]
                "Channel 2 Wave (Main)" <- w1164
                "Channel 3 Wave (Main)" <- w1163
                "Channel 1 Wave (Main)" <- w1165
                "Channel 4 Wave (Main)" <- w1162
                n321 = Enqueue Element At Opposite End(queue=w1174, element=cluster{"State":T15, "Data":variant} {"State"=enum."Test", "Data"=variant}, error in (no error)=w1171) -> (queue out=w1173:refnum<queue>, error out=w1170:errorcluster)  [unwired: 1 in, 1 out]
                n322 = Bundle By Name(cluster=w1169, "Channel 1 Wave"=w1165, "Channel 2 Wave"=w1164, "Channel 3 Wave"=w1163, "Channel 4 Wave"=w1162, "Set Time"=6000, "Rate"=600.0 ("Elapse Time"), "Channel 1"=w1159, "Channel 2"=w1158, "Channel 3"=w1157, "Channel 4"=w1156) -> (w1168:T16)
              }
              frame "Leftward" {
                n323 = Unbundle(T25 {"Channel 1"={" frequency 1"=60, "signal type 1"=enum."Sine Wave", "amplitude 1"=0.0, "offset"=0.0, "phase"=0.0}, "Channel 2"={" frequency 1"=60, "signal type 1"=enum."Sine Wave", "amplitude 1"=0.0, "offset"=0.0, "phase"=0}, "Channel 3"={" frequency 1"=60, "signal type 1"=enum."Sine Wave", "amplitude 1"=0.0, "offset"=0.0, "phase"=0.0}, "Channel 4"={" frequency 1"=60, "signal type 1"=enum."Sine Wave", "amplitude 1"=0.6, "offset"=0.0, "phase"=0}} ("Front")) -> ("Channel 1"=w1188:T37, "Channel 2"=w1187:T38, "Channel 3"=w1186:T37, "Channel 4"=w1185:T38)
                n324 = Build Array(w1188, w1187, w1186, w1185) -> (w1196:T39)
                n325 = for {
                  tunnel: w1196 -> [w1204] mode=indexing
                  tunnel: [w1205] -> w1195 mode=indexing
                  n326 = Unbundle By Name(w1204) -> ("offset"=w1206:dbl, "signal type 1"=w1207:T30, "frequency 1"=w1208:i32, "amplitude 1"=w1209:dbl, "phase"=w1210:dbl)
                  n327 = call <vilib>:"Basic Function Generator.vi"("offset"=w1206, "reset signal"=TRUE, "sampling info"=cluster{"Fs":dbl, "#s":dbl} {"Fs"=1000.0, "#s"=100.0} ("sampling info 4"), "signal type"=w1207, "phase"=w1210, "amplitude"=w1209, "frequency"=w1208) -> ("signal out"=w1205:waveform(dbl))  [unwired: 2 in, 2 out]
                }
                n328 = Index Array(array=w1195) -> (element #1=w1192:waveform(dbl), element #2=w1191:waveform(dbl), element #3=w1190:waveform(dbl), element #4=w1189:waveform(dbl))  [unwired: 4 in]
                n329 = property on="Channel 3 Wave (Main)" class="WFGraph (strict)"("Value"=w1190) -> ()  [unwired: 2 in, 2 out]
                n330 = property on="Channel 1 Wave (Main)" class="WFGraph (strict)"("Value"=w1192) -> ()  [unwired: 2 in, 2 out]
                n331 = Enqueue Element At Opposite End(queue=w1203, element=cluster{"State":T15, "Data":variant} {"State"=enum."Test", "Data"=variant}, error in (no error)=w1200) -> (queue out=w1202:refnum<queue>, error out=w1199:errorcluster)  [unwired: 1 in, 1 out]
                n332 = property on="Channel 4 Wave (Main)" class="WFGraph (strict)"("Value"=w1189) -> ()  [unwired: 2 in, 2 out]
                n333 = property on="Channel 2 Wave (Main)" class="WFGraph (strict)"("Value"=w1191) -> ()  [unwired: 2 in, 2 out]
                n334 = Bundle By Name(cluster=w1198, "Channel 1 Wave"=w1192, "Channel 2 Wave"=w1191, "Channel 3 Wave"=w1190, "Channel 4 Wave"=w1189, "Set Time"=6000, "Rate"=600.0 ("Elapse Time"), "Channel 1"=w1188, "Channel 2"=w1187, "Channel 3"=w1186, "Channel 4"=w1185) -> (w1197:T16)
              }
              frame "Backward" {
                n335 = Unbundle(T25 {"Channel 1"={" frequency 1"=60, "signal type 1"=enum."Sine Wave", "amplitude 1"=0.0, "offset"=0.0, "phase"=0.0}, "Channel 2"={" frequency 1"=60, "signal type 1"=enum."Sine Wave", "amplitude 1"=0.0, "offset"=0.0, "phase"=0}, "Channel 3"={" frequency 1"=60, "signal type 1"=enum."Sine Wave", "amplitude 1"=0.6, "offset"=0.0, "phase"=0.0}, "Channel 4"={" frequency 1"=60, "signal type 1"=enum."Sine Wave", "amplitude 1"=0.0, "offset"=0.0, "phase"=0}} ("Front")) -> ("Channel 1"=w1217:T37, "Channel 2"=w1216:T38, "Channel 3"=w1215:T37, "Channel 4"=w1214:T38)
                n336 = Build Array(w1217, w1216, w1215, w1214) -> (w1225:T39)
                n337 = for {
                  tunnel: w1225 -> [w1233] mode=indexing
                  tunnel: [w1234] -> w1224 mode=indexing
                  n338 = Unbundle By Name(w1233) -> ("offset"=w1235:dbl, "signal type 1"=w1236:T30, "frequency 1"=w1237:i32, "amplitude 1"=w1238:dbl, "phase"=w1239:dbl)
                  n339 = call <vilib>:"Basic Function Generator.vi"("offset"=w1235, "reset signal"=TRUE, "sampling info"=cluster{"Fs":dbl, "#s":dbl} {"Fs"=1000.0, "#s"=100.0} ("sampling info 4"), "signal type"=w1236, "phase"=w1239, "amplitude"=w1238, "frequency"=w1237) -> ("signal out"=w1234:waveform(dbl))  [unwired: 2 in, 2 out]
                }
                n340 = Index Array(array=w1224) -> (element #1=w1221:waveform(dbl), element #2=w1220:waveform(dbl), element #3=w1219:waveform(dbl), element #4=w1218:waveform(dbl))  [unwired: 4 in]
                n341 = property on="Channel 3 Wave (Main)" class="WFGraph (strict)"("Value"=w1219) -> ()  [unwired: 2 in, 2 out]
                n342 = property on="Channel 1 Wave (Main)" class="WFGraph (strict)"("Value"=w1221) -> ()  [unwired: 2 in, 2 out]
                n343 = Enqueue Element At Opposite End(queue=w1232, element=cluster{"State":T15, "Data":variant} {"State"=enum."Test", "Data"=variant}, error in (no error)=w1229) -> (queue out=w1231:refnum<queue>, error out=w1228:errorcluster)  [unwired: 1 in, 1 out]
                n344 = property on="Channel 4 Wave (Main)" class="WFGraph (strict)"("Value"=w1218) -> ()  [unwired: 2 in, 2 out]
                n345 = property on="Channel 2 Wave (Main)" class="WFGraph (strict)"("Value"=w1220) -> ()  [unwired: 2 in, 2 out]
                n346 = Bundle By Name(cluster=w1227, "Channel 1 Wave"=w1221, "Channel 2 Wave"=w1220, "Channel 3 Wave"=w1219, "Channel 4 Wave"=w1218, "Set Time"=6000, "Rate"=600.0 ("Elapse Time"), "Channel 1"=w1217, "Channel 2"=w1216, "Channel 3"=w1215, "Channel 4"=w1214) -> (w1226:T16)
              }
              frame "Rightward" {
                n347 = Unbundle(T25 {"Channel 1"={" frequency 1"=60, "signal type 1"=enum."Sine Wave", "amplitude 1"=0.0, "offset"=0.0, "phase"=0.0}, "Channel 2"={" frequency 1"=60, "signal type 1"=enum."Sine Wave", "amplitude 1"=0.6, "offset"=0.0, "phase"=0}, "Channel 3"={" frequency 1"=60, "signal type 1"=enum."Sine Wave", "amplitude 1"=0.0, "offset"=0.0, "phase"=0.0}, "Channel 4"={" frequency 1"=60, "signal type 1"=enum."Sine Wave", "amplitude 1"=0.0, "offset"=0.0, "phase"=0}} ("Front")) -> ("Channel 1"=w1245:T37, "Channel 2"=w1246:T38, "Channel 3"=w1244:T37, "Channel 4"=w1243:T38)
                n348 = Build Array(w1245, w1246, w1244, w1243) -> (w1254:T39)
                n349 = for {
                  tunnel: w1254 -> [w1262] mode=indexing
                  tunnel: [w1263] -> w1253 mode=indexing
                  n350 = Unbundle By Name(w1262) -> ("offset"=w1264:dbl, "signal type 1"=w1265:T30, "frequency 1"=w1266:i32, "amplitude 1"=w1267:dbl, "phase"=w1268:dbl)
                  n351 = call <vilib>:"Basic Function Generator.vi"("offset"=w1264, "reset signal"=TRUE, "sampling info"=cluster{"Fs":dbl, "#s":dbl} {"Fs"=1000.0, "#s"=100.0} ("sampling info 4"), "signal type"=w1265, "phase"=w1268, "amplitude"=w1267, "frequency"=w1266) -> ("signal out"=w1263:waveform(dbl))  [unwired: 2 in, 2 out]
                }
                n352 = Index Array(array=w1253) -> (element #1=w1250:waveform(dbl), element #2=w1249:waveform(dbl), element #3=w1248:waveform(dbl), element #4=w1247:waveform(dbl))  [unwired: 4 in]
                n353 = property on="Channel 3 Wave (Main)" class="WFGraph (strict)"("Value"=w1248) -> ()  [unwired: 2 in, 2 out]
                n354 = property on="Channel 1 Wave (Main)" class="WFGraph (strict)"("Value"=w1250) -> ()  [unwired: 2 in, 2 out]
                n355 = Enqueue Element At Opposite End(queue=w1261, element=cluster{"State":T15, "Data":variant} {"State"=enum."Test", "Data"=variant}, error in (no error)=w1258) -> (queue out=w1260:refnum<queue>, error out=w1257:errorcluster)  [unwired: 1 in, 1 out]
                n356 = property on="Channel 4 Wave (Main)" class="WFGraph (strict)"("Value"=w1247) -> ()  [unwired: 2 in, 2 out]
                n357 = property on="Channel 2 Wave (Main)" class="WFGraph (strict)"("Value"=w1249) -> ()  [unwired: 2 in, 2 out]
                n358 = Bundle By Name(cluster=w1256, "Channel 1 Wave"=w1250, "Channel 2 Wave"=w1249, "Channel 3 Wave"=w1248, "Channel 4 Wave"=w1247, "Set Time"=6000, "Rate"=600.0 ("Elapse Time"), "Channel 1"=w1245, "Channel 2"=w1246, "Channel 3"=w1244, "Channel 4"=w1243) -> (w1255:T16)
              }
              frame "Center" {
                n359 = Unbundle(T25 {"Channel 1"={" frequency 1"=60, "signal type 1"=enum."Sine Wave", "amplitude 1"=0.6, "offset"=0.0, "phase"=0.0}, "Channel 2"={" frequency 1"=60, "signal type 1"=enum."Sine Wave", "amplitude 1"=0.6, "offset"=0.0, "phase"=90}, "Channel 3"={" frequency 1"=60, "signal type 1"=enum."Sine Wave", "amplitude 1"=0.6, "offset"=0.0, "phase"=180.0}, "Channel 4"={" frequency 1"=60, "signal type 1"=enum."Sine Wave", "amplitude 1"=0.6, "offset"=0.0, "phase"=270}} ("Front")) -> ("Channel 1"=w1274:T37, "Channel 2"=w1273:T38, "Channel 3"=w1272:T37, "Channel 4"=w1271:T38)
                n360 = Build Array(w1274, w1273, w1272, w1271) -> (w1282:T39)
                n361 = for {
                  tunnel: w1282 -> [w1291] mode=indexing
                  tunnel: [w1292] -> w1281 mode=indexing
                  n362 = Unbundle By Name(w1291) -> ("offset"=w1293:dbl, "signal type 1"=w1294:T30, "frequency 1"=w1295:i32, "amplitude 1"=w1296:dbl, "phase"=w1297:dbl)
                  n363 = call <vilib>:"Basic Function Generator.vi"("offset"=w1293, "reset signal"=TRUE, "sampling info"=cluster{"Fs":dbl, "#s":dbl} {"Fs"=1000.0, "#s"=100.0} ("sampling info 4"), "signal type"=w1294, "phase"=w1297, "amplitude"=w1296, "frequency"=w1295) -> ("signal out"=w1292:waveform(dbl))  [unwired: 2 in, 2 out]
                }
                n364 = Index Array(array=w1281) -> (element #1=w1278:waveform(dbl), element #2=w1277:waveform(dbl), element #3=w1276:waveform(dbl), element #4=w1275:waveform(dbl))  [unwired: 4 in]
                n365 = property on="Channel 3 Wave (Main)" class="WFGraph (strict)"("Value"=w1276) -> ()  [unwired: 2 in, 2 out]
                n366 = property on="Channel 1 Wave (Main)" class="WFGraph (strict)"("Value"=w1278) -> ()  [unwired: 2 in, 2 out]
                n367 = Enqueue Element At Opposite End(queue=w1290, element=cluster{"State":T15, "Data":variant} {"State"=enum."Test", "Data"=variant}, error in (no error)=w1287) -> (queue out=w1289:refnum<queue>, error out=w1286:errorcluster)  [unwired: 1 in, 1 out]
                n368 = property on="Channel 2 Wave (Main)" class="WFGraph (strict)"("Value"=w1277) -> ()  [unwired: 2 in, 2 out]
                n369 = property on="Channel 4 Wave (Main)" class="WFGraph (strict)"("Value"=w1275) -> ()  [unwired: 2 in, 2 out]
                n370 = Bundle By Name(cluster=w1285, "Channel 1 Wave"=w1278, "Channel 2 Wave"=w1277, "Channel 3 Wave"=w1276, "Channel 4 Wave"=w1275, "Set Time"=5000, "Rate"=600.0 ("Elapse Time"), "Channel 1"=w1274, "Channel 2"=w1273, "Channel 3"=w1272, "Channel 4"=w1271) -> (w1284:T16)
              }
              frame "Bump" {
                n371 = Unbundle(T25 {"Channel 1"={" frequency 1"=60, "signal type 1"=enum."Sine Wave", "amplitude 1"=0.6, "offset"=0.0, "phase"=0.0}, "Channel 2"={" frequency 1"=60, "signal type 1"=enum."Sine Wave", "amplitude 1"=0.6, "offset"=0.0, "phase"=0}, "Channel 3"={" frequency 1"=60, "signal type 1"=enum."Sine Wave", "amplitude 1"=0.6, "offset"=0.0, "phase"=0.0}, "Channel 4"={" frequency 1"=60, "signal type 1"=enum."Sine Wave", "amplitude 1"=0.6, "offset"=0.0, "phase"=0}} ("Front")) -> ("Channel 1"=w1304:T37, "Channel 2"=w1303:T38, "Channel 3"=w1302:T37, "Channel 4"=w1301:T38)
                n372 = Build Array(w1304, w1303, w1302, w1301) -> (w1311:T39)
                n373 = for {
                  tunnel: w1311 -> [w1320] mode=indexing
                  tunnel: [w1321] -> w1310 mode=indexing
                  n374 = Unbundle By Name(w1320) -> ("offset"=w1322:dbl, "signal type 1"=w1323:T30, "frequency 1"=w1324:i32, "amplitude 1"=w1325:dbl, "phase"=w1326:dbl)
                  n375 = call <vilib>:"Basic Function Generator.vi"("offset"=w1322, "reset signal"=TRUE, "sampling info"=cluster{"Fs":dbl, "#s":dbl} {"Fs"=1000.0, "#s"=100.0} ("sampling info 4"), "signal type"=w1323, "phase"=w1326, "amplitude"=w1325, "frequency"=w1324) -> ("signal out"=w1321:waveform(dbl))  [unwired: 2 in, 2 out]
                }
                n376 = Index Array(array=w1310) -> (element #1=w1308:waveform(dbl), element #2=w1307:waveform(dbl), element #3=w1306:waveform(dbl), element #4=w1305:waveform(dbl))  [unwired: 4 in]
                n377 = property on="Channel 3 Wave (Main)" class="WFGraph (strict)"("Value"=w1306) -> ()  [unwired: 2 in, 2 out]
                n378 = property on="Channel 1 Wave (Main)" class="WFGraph (strict)"("Value"=w1308) -> ()  [unwired: 2 in, 2 out]
                n379 = Enqueue Element At Opposite End(queue=w1319, element=cluster{"State":T15, "Data":variant} {"State"=enum."Test", "Data"=variant}, error in (no error)=w1316) -> (queue out=w1318:refnum<queue>, error out=w1315:errorcluster)  [unwired: 1 in, 1 out]
                n380 = property on="Channel 4 Wave (Main)" class="WFGraph (strict)"("Value"=w1305) -> ()  [unwired: 2 in, 2 out]
                n381 = property on="Channel 2 Wave (Main)" class="WFGraph (strict)"("Value"=w1307) -> ()  [unwired: 2 in, 2 out]
                n382 = Bundle By Name(cluster=w1314, "Channel 1 Wave"=w1308, "Channel 2 Wave"=w1307, "Channel 3 Wave"=w1306, "Channel 4 Wave"=w1305, "Set Time"=3000, "Rate"=600.0 ("Elapse Time"), "Channel 1"=w1304, "Channel 2"=w1303, "Channel 3"=w1302, "Channel 4"=w1301) -> (w1313:T16)
              }
              frame "Stop" {
                n383 = property on="Testing?" class="Bool (strict)"("Value"=FALSE ("Testing?")) -> ()  [unwired: 2 in, 2 out]
                n384 = Enqueue Element At Opposite End(queue=w1337, element=cluster{"State":T15, "Data":variant} {"State"=enum."Idle", "Data"=variant}, error in (no error)=w1335) -> (queue out=w1336:refnum<queue>, error out=w1334:errorcluster)  [unwired: 1 in, 1 out]
                n385 = Bundle By Name(cluster=w1332, "Stop"=TRUE) -> (w1331:T16)
              }
              frame "Add Project" {
                n386 = Unbundle By Name(w1344) -> ("Project Path"=w1345:path, "Project List name"=w1342:string[], "Project Name(Set)"=w1339:string)
                n387 = Search 1D Array(1D array=w1342, element=w1339) -> (index of element=w1341:i32)  [unwired: 1 in]
                n388 = Greater Or Equal To 0?(x=w1341) -> (x >= 0?=w1340:bool)
                n389 = Empty String/Path?(string/path=w1339) -> (empty?=w1338:bool)
                n390 = case shown="False" w1338 {
                  tunnel: w1345 -> [w1355 _]
                  tunnel: w1344 -> [w1354 w1381]
                  tunnel: [w1353 w1381] -> w1343
                  tunnel: w1340 -> [w1352 _]
                  tunnel: w1339 -> [w1351 _]
                  frame False {
                    n391 = case shown="False" w1352 {
                      tunnel: w1355 -> [w1369 w1380]
                      tunnel: w1354 -> [w1364 w1371]
                      tunnel: [w1368 w1371] -> w1353
                      tunnel: w1351 -> [w1366 w1379]
                      frame False {
                        w1356 = string[] [] ("Item Names")
                        w1357 = T1 [] ("DataTable")
                        n392 = Build Path(base path=w1369, name or relative path=w1366) -> (appended path=w1360:path)
                        n393 = Create Folder(path (use dialog)=w1360) -> (error out=w1370:errorcluster)  [unwired: 2 in, 2 out]
                        n394 = Build Path(base path=w1360, name or relative path="Channel Setting.dat") -> (appended path=w1361:path)
                        n395 = List Folder(path=w1369, error in=w1370) -> (folder names=w1367:string[], error out=w1358:errorcluster)  [unwired: 2 in, 2 out]
                        n396 = Bundle("DataTable"=w1357, "Item Names"=w1356) -> (w1363:T32)  [unwired: 1 in]
                        n397 = Flatten To XML(anything=w1363) -> (xml string=w1365:string)
                        n398 = call-poly <vilib>:"Write to XML File.vi"("error in (no error)"=w1358, "XML Input"=w1365, "XML File Path"=w1361) -> ()  [unwired: 6 in, 3 out]
                        n399 = Bundle By Name(cluster=w1364, "Project List name"=w1367, "Project Name(Set)"="", "Channel Table"=w1357, "Model List name"=w1356) -> (w1368:T16)
                      }
                      frame True {
                        n400 = Unbundle By Name(w1371) -> ("Channel Table"=w1377:T1, "Model List name"=w1376:string[])
                        n401 = Build Path(base path=w1380, name or relative path=w1379) -> (appended path=w1372:path)
                        n402 = Bundle("Channel Table"=w1377, "Model List name"=w1376) -> (w1375:T36)  [unwired: 1 in]
                        n403 = Flatten To XML(anything=w1375) -> (xml string=w1378:string)
                        n404 = Build Path(base path=w1372, name or relative path="Channel Setting.dat") -> (appended path=w1373:path)
                        n405 = call-poly <vilib>:"Write to XML File.vi"("XML Input"=w1378, "XML File Path"=w1373) -> ()  [unwired: 7 in, 3 out]
                      }
                    }
                  }
                  frame True {
                  }
                }
                n406 = Enqueue Element At Opposite End(queue=w1350, element=cluster{"State":T15, "Data":variant} {"State"=enum."Update", "Data"=variant}, error in (no error)=w1347) -> (queue out=w1349:refnum<queue>, error out=w1346:errorcluster)  [unwired: 1 in, 1 out]
              }
              frame "Remove Project" {
                w1382 = cluster{"Sample Rate":dbl, "Samples":dbl} {"Sample Rate"=0.0, "Samples"=0.0} ("Channel 1 Sample")
                w1385 = T23 {" frequency 1"=0, "signal type 1"=enum."Sine Wave", "amplitude 1"=0.0, "offset"=0.0, "phase"=0.0} ("Channel 1")
                w1386 = waveform(dbl) {"t0"=timestamp(0 s since 1904-01-01), "dt"=1.0, "Y"=[]} ("Channel 1 Wave")
                n407 = Unbundle By Name(w1398) -> ("Project Path"=w1392:path, "Project List name"=w1396:string[], "ProjectList Num"=w1395:i32)
                n408 = Index Array(array=w1396, index=w1395) -> (element=w1394:string)
                n409 = Build Path(base path=w1392, name or relative path=w1394) -> (appended path=w1393:path)
                n410 = Delete(path (use dialog)=w1393, entire hierarchy (F)=TRUE) -> (error out=w1391:errorcluster)  [unwired: 3 in, 2 out]
                n411 = List Folder(path=w1392, error in=w1391) -> (folder names=w1390:string[])  [unwired: 2 in, 3 out]
                n412 = Bundle By Name(cluster=w1398, "Rate"=0.0, "Channel 1 Sample"=w1382, "Channel 2 Sample"=w1382, "Channel 3 Sample"=w1382, "Channel 4 Sample"=w1382, "Channel Table"=T1 [] ("DataTable"), "Model List name"=string[] [] ("Item Names"), "Project List name"=w1390, "Channel 1 Wave"=w1386, "Channel 2 Wave"=w1386, "Channel 3 Wave"=w1386, "Channel 4 Wave"=w1386, "Channel 1"=w1385, "Channel 2"=w1385, "Channel 3"=w1385, "Channel 4"=w1385, "Set Time"=0) -> (w1397:T16)
                n413 = Enqueue Element At Opposite End(queue=w1403, element=cluster{"State":T15, "Data":variant} {"State"=enum."Update", "Data"=variant}, error in (no error)=w1400) -> (queue out=w1402:refnum<queue>, error out=w1399:errorcluster)  [unwired: 1 in, 1 out]
              }
              frame "Project List" {
                n414 = Variant To Data(error in=w1406, type=0 ("NewVal"), Variant=w1407) -> (data=w1404:i32, error out=w1405:errorcluster)
                n415 = Bundle By Name(cluster=w1410, "ProjectList Num"=w1404) -> (w1409:T16)
                n416 = Enqueue Element At Opposite End(queue=w1414, element=cluster{"State":T15, "Data":variant} {"State"=enum."Update", "Data"=variant}, error in (no error)=w1405) -> (queue out=w1413:refnum<queue>, error out=w1411:errorcluster)  [unwired: 1 in, 1 out]
              }
              frame "Project Name" {
                n417 = Variant To Data(error in=w1417, type="" ("NewVal"), Variant=w1418) -> (data=w1415:string, error out=w1416:errorcluster)
                n418 = Bundle By Name(cluster=w1421, "Project Name(Set)"=w1415) -> (w1420:T16)
                n419 = Enqueue Element At Opposite End(queue=w1425, element=cluster{"State":T15, "Data":variant} {"State"=enum."Update", "Data"=variant}, error in (no error)=w1416) -> (queue out=w1424:refnum<queue>, error out=w1422:errorcluster)  [unwired: 1 in, 1 out]
              }
              frame "Project OK" {
                n420 = Unbundle By Name(w1433) -> ("Project Path"=w1432:path, "Project List name"=w1428:string[], "ProjectList Num"=w1429:i32)
                n421 = Empty Array?(array=w1428) -> (empty?=w1427:bool)
                n422 = case shown="False" w1427 {
                  tunnel: [w1472 w1492] -> w1434
                  tunnel: w1433 -> [w1458 w1492]
                  tunnel: w1432 -> [w1465 _]
                  tunnel: w1431 -> [w1464 w1493]
                  tunnel: [w1463 w1493] -> w1430
                  tunnel: w1428 -> [w1462 _]
                  tunnel: w1429 -> [w1461 _]
                  frame False {
                    w1455 = 0 ("index")
                    n423 = Index Array(array=w1462, index=w1461) -> (element=w1453:string)
                    n424 = Build Path(base path=w1465, name or relative path=w1453) -> (appended path=w1466:path)
                    n425 = Build Path(base path=w1466, name or relative path="Channel Setting.dat") -> (appended path=w1469:path)
                    n426 = call <vilib>:"Check if File or Folder Exists.vi"("error in (no error)"=w1464, "path"=w1469) -> ("error out"=w1470:errorcluster, "file or folder exists?"=w1468:bool, "dup path"=w1467:path)  [unwired: 7 in]
                    n427 = case shown="True" w1468 {
                      tunnel: [w1482 w1486] -> w1463
                      tunnel: w1470 -> [w1482 w1485]
                      tunnel: w1467 -> [_ w1484]
                      tunnel: [_ w1483] -> w1460
                      frame False {
                      }
                      frame True {
                        n428 = call-poly <vilib>:"Read From XML File.vi"("error in (no error)"=w1485, "XML File Path"=w1484) -> ("error out"=w1487:errorcluster, "XML Elements"=w1491:string)  [unwired: 7 in, 1 out]
                        n429 = Bundle("DataTable"=T1 [], "Item Names"=string[] []) -> (w1488:T32)  [unwired: 1 in]
                        n430 = Unflatten From XML(xml string=w1491, type=w1488, error in (no error)=w1487) -> (value=w1483:T32, error out=w1486:errorcluster)
                      }
                    }
                    n431 = Unbundle(w1460) -> ("DataTable"=w1457:T1, "Item Names"=w1459:string[])
                    n432 = Index Array(array=w1457, index=w1455) -> (element=w1456:T34)
                    n433 = Unbundle(w1456) -> ("Channel 1"=w1451:T23, "Channel 2"=w1450:T23, "Channel 3"=w1449:T23, "Channel 4"=w1448:T23, "Time(ms)"=w1454:i32, "Rate"=w1442:dbl, "Channel 1 Sample"=w1441:cluster{"Sample Rate":dbl, "Samples":dbl}, "Channel 2 Sample"=w1440:cluster{"Sample Rate":dbl, "Samples":dbl}, "Channel 3 Sample"=w1439:cluster{"Sample Rate":dbl, "Samples":dbl}, "Channel 4 Sample"=w1438:cluster{"Sample Rate":dbl, "Samples":dbl})
                    n434 = Build Array(w1451, w1450, w1449, w1448) -> (w1452:T35)
                    n435 = for {
                      tunnel: w1452 -> [w1476] mode=indexing
                      tunnel: [w1477] -> w1447 mode=indexing
                      n436 = Unbundle(w1476) -> ("frequency 1"=w1474:u32, "signal type 1"=w1478:T30, "amplitude 1"=w1475:dbl, "offset"=w1473:dbl, "phase"=w1479:dbl)
                      n437 = call <vilib>:"Basic Function Generator.vi"("offset"=w1473, "reset signal"=TRUE, "sampling info"=cluster{"Fs":dbl, "#s":dbl} {"Fs"=1000.0, "#s"=100.0} ("sampling info 4"), "signal type"=w1478, "phase"=w1479, "amplitude"=w1475, "frequency"=w1474) -> ("signal out"=w1477:waveform(dbl))  [unwired: 2 in, 2 out]
                    }
                    n438 = Index Array(array=w1447) -> (element #1=w1446:waveform(dbl), element #2=w1445:waveform(dbl), element #3=w1444:waveform(dbl), element #4=w1443:waveform(dbl))  [unwired: 4 in]
                    n439 = Bundle By Name(cluster=w1458, "Channel Table"=w1457, "Model List name"=w1459, "Channel 1 Wave"=w1446, "Channel 2 Wave"=w1445, "Channel 3 Wave"=w1444, "Channel 4 Wave"=w1443, "Channel 1"=w1451, "Channel 2"=w1450, "Channel 3"=w1449, "Channel 4"=w1448, "Set Time"=w1454, "Rate"=w1442, "Channel 1 Sample"=w1441, "Channel 2 Sample"=w1440, "Channel 3 Sample"=w1439, "Channel 4 Sample"=w1438, "ModelList Num"=w1455, "Project Name"=w1453) -> (w1472:T16)
                  }
                  frame True {
                  }
                }
                n440 = Enqueue Element At Opposite End(queue=w1437, element=cluster{"State":T15, "Data":variant} {"State"=enum."Update", "Data"=variant}, error in (no error)=w1430) -> (queue out=w1436:refnum<queue>, error out=w1435:errorcluster)  [unwired: 1 in, 1 out]
              }
              frame "Response" {
                n441 = Variant To Data(type="", Variant=w1497) -> (data=w1495:string)  [unwired: 1 in, 1 out]
                n442 = Enqueue Element(queue=w1498, element=w1495) -> (error out=w1494:errorcluster)  [unwired: 2 in, 2 out]
              }
              frame "Exit" {
                w1502 = TRUE
                n443 = call "FGV_EXIT.vi"("Function"=enum16{"Read", "Write"}."Write", "EXIT"=w1502) -> ()  [unwired: 6 in, 1 out]
              }
            }
            n444 = call "FGV_EXIT.vi"("Function"=enum16{"Read", "Write"}."Read") -> ("EXIT out"=w454:bool)  [unwired: 7 in]
            n445 = Or(x=w456, y=w454) -> (x .or. y?=w457:bool)
            n446 = case shown="True" w457 {
              tunnel: w466 -> [w475 w484]
              tunnel: w465 -> [w476 w485]
              tunnel: [w476 w485] -> w464
              tunnel: [w475 w481] -> w463
              tunnel: [w474 w480] -> w462
              tunnel: w456 -> [w474 w478]
              tunnel: w454 -> [_ w477]
              frame False {
              }
              frame True {
                n447 = call <vilib>:"Clear Errors.vi"("error in (no error)"=w478) -> ("error out"=w479:errorcluster)  [unwired: 5 in, 1 out]
                n448 = case shown="False" w477 {
                  tunnel: w478 -> [w486 _]
                  frame False {
                    n449 = Unbundle By Name(w486) -> ("source"=w491:string, "code"=w492:i32)
                    n450 = Format Into String(format string="ErrorCode:%d_ErrorMsg:%s", w492, w491) -> (resulting string=w490:string)  [unwired: 2 in, 1 out]
                    n451 = One Button Dialog(message=w491) -> ()  [unwired: 1 in, 1 out]
                    n452 = Bundle By Name(cluster=T18 {"MsgPageSelect"=enum."Alarm", "LogType"=enum."Auto", "Msg"="", "Time"=""} ("DataIn"), "Msg"=w490) -> (w489:T18)
                    n453 = call "SendMsg.vi"("DataIn"=w489) -> ()  [unwired: 10 in, 1 out]
                  }
                  frame True {
                  }
                }
                n454 = Flush Queue(queue=w484, error in (no error)=w479) -> (queue out=w482:refnum<queue>, error out=w483:errorcluster)  [unwired: 1 out]
                n455 = disable-structure shown="Enabled" {
                  disable-tunnel: w483 -> [w497 w498]
                  disable-tunnel: w482 -> [w496 w499]
                  disable-tunnel: [w495 w499] -> w481
                  disable-tunnel: [w494 w498] -> w480
                  frame Disabled {
                    n456 = Enqueue Element(queue=w496, element=cluster{"State":T15, "Data":variant} {"State"=enum."Exit", "Data"=variant}, error in (no error)=w497) -> (queue out=w495:refnum<queue>, error out=w494:errorcluster)  [unwired: 1 in, 1 out]
                  }
                  frame Enabled {
                  }
                }
              }
            }
          }
          n457 = while {
            tunnel: w117 -> [w1506]
            tunnel: w126 -> [w1511]
            tunnel: [w1506] -> w120
            stop <- w1509 stop-if-true
            n458 = event shown="[33] \"SequenceName\": Value Change;  \"SequenceName\": Mouse Down" {
              selector: _ -> [_ _ _ _ _ _ _ _ _ _ _ _ _ _ _ _ _ _ _ _ _ _ _ _ _ _ _ _ _ _ _ _ _ _]
              dyn-events: _ -> [_ _ _ _ _ _ _ _ _ _ _ _ _ _ _ _ _ _ _ _ _ _ _ _ _ _ _ _ _ _ _ _ _ _]
              timeout: 137 -> [_ _ _ _ _ _ _ _ _ _ _ _ _ _ _ _ _ _ _ _ _ _ _ _ _ _ _ _ _ _ _ _ _ _]
              tunnel: [w1520 w1522 _ _ _ _ _ _ _ _ _ _ _ _ _ _ _ _ _ _ _ _ _ _ _ _ _ _ _ _ _ _ _ _] -> w1512
              tunnel: w1506 -> [_ w1526 w1530 w1535 w1541 w1577 w1609 w1613 w1616 w1624 w1630 w1634 w1638 w1642 w1646 w1650 w1654 w1657 w1660 w1665 w1670 w1674 w1677 _ _ _ w1685 _ _ _ _ _ _ _]
              tunnel: w1511 -> [_ w1527 w1529 w1536 w1540 w1576 w1608 w1614 w1617 w1625 w1631 w1635 w1639 w1643 w1647 w1651 w1655 w1658 w1661 w1666 w1671 w1673 w1678 _ _ _ w1686 _ _ _ _ _ _ _]
              event Timeout {
                n459 = event-data() -> ()  [unwired: 1 in, 3 out]
                n460 = property on="SequenceName" class="Ring (strict)"() -> ("RingText.Text"=w1519:string)  [unwired: 2 in, 2 out]
                n461 = call <vilib>:"Trim Whitespace.vi"("string"=w1519) -> ("trimmed string"=w1518:string)  [unwired: 1 in]
                n462 = String Length(string=w1518) -> (length=w1517:i32)
                n463 = Greater Than 0?(x=w1517) -> (x > 0?=w1516:bool)
                n464 = Select(t=T26."Enabled" ("Disabled"), s=w1516, f=T26."Disabled and Grayed Out" ("Disabled")) -> (s? t:f=w1513:T26)
                n465 = property on="SequenceList" class="LstBox (strict)"("DisabledEnum"=w1513) -> ()  [unwired: 2 in, 2 out]
                n466 = property on="RemoveSeq" class="Bool"("DisabledEnum"=w1513) -> ()  [unwired: 2 in, 2 out]
                n467 = property on="AddSeq" class="Bool"("DisabledEnum"=w1513) -> ()  [unwired: 2 in, 2 out]
                n468 = call "Exit.vi"() -> ("ExitOut"=w1520:bool)  [unwired: 11 in]
              }
              event "Exit Button": Value Change {
                w1522 = TRUE
                n469 = event-data() -> ()  [unwired: 1 in, 2 out]
                n470 = Flush Queue(queue=w1526, error in (no error)=w1527) -> (queue out=w1524:refnum<queue>, error out=w1525:errorcluster)  [unwired: 1 out]
                n471 = Enqueue Element(queue=w1524, element=cluster{"State":T15, "Data":variant} {"State"=enum."Exit", "Data"=variant}, error in (no error)=w1525) -> ()  [unwired: 1 in, 3 out]
                n472 = call "FGV_EXIT.vi"("Function"=enum16{"Read", "Write"}."Write", "EXIT"=w1522) -> ()  [unwired: 6 in, 1 out]
              }
              event "Play Button": Value Change {
                n473 = event-data() -> ()  [unwired: 1 in, 6 out]
                n474 = Enqueue Element(queue=w1530, element=cluster{"State":T15, "Data":variant} {"State"=enum."Test", "Data"=variant}, error in (no error)=w1529) -> ()  [unwired: 1 in, 3 out]
              }
              event "Time(ms)": Value Change {
                n475 = event-data() -> ()  [unwired: 1 in, 1 out]
                n476 = Bundle(cluster=cluster{"State":T15, "Data":variant} {"State"=enum."Initalize", "Data"=variant}, "State"=State."Set Time", "Data"="Time(ms)") -> (w1533:cluster{"State":T15, "Data":variant})
                n477 = Enqueue Element(queue=w1535, element=w1533, error in (no error)=w1536) -> ()  [unwired: 1 in, 3 out]
              }
              event "Channel 1", "Channel 2", "Channel 4", "Channel 3": Value Change {
                n478 = event-data() -> ("CtlRef"=w1546:refnum<vi>)  [unwired: 1 in]
                n479 = property class="Clust (strict)"(reference=w1546) -> ("Label.Text"=w1545:string)  [unwired: 1 in, 2 out]
                n480 = Match Pattern(string=w1545, regular expression="Channel") -> (after substring=w1543:string)  [unwired: 1 in, 3 out]
                n481 = Decimal String To Number(string=w1543) -> (number=w1542:i32)  [unwired: 2 in, 1 out]
                n482 = case shown="1" w1542 {
                  tunnel: w1541 -> [w1549 w1553 w1558 w1563 w1568]
                  tunnel: w1540 -> [w1548 w1554 w1559 w1564 w1569]
                  tunnel: [w1548 w1554 w1559 w1564 w1569] -> w1539
                  tunnel: [w1549 w1553 w1558 w1563 w1568] -> w1538
                  tunnel: [cluster{"State":T15, "Data":variant} {"State"=enum."Update", "Data"=variant} w1551 w1557 w1561 w1567] -> w1537
                  frame 0, Default {
                  }
                  frame 1 {
                    n483 = Bundle("State"=State."Channel1", "Channel 1"="Channel 1") -> (w1551:T40)  [unwired: 1 in]
                  }
                  frame 2 {
                    n484 = Bundle("State"=State."Channel2", "Channel 2"="Channel 2") -> (w1557:T41)  [unwired: 1 in]
                  }
                  frame 3 {
                    n485 = Bundle("State"=State."Channel3", "Channel 3"="Channel 3") -> (w1561:T42)  [unwired: 1 in]
                  }
                  frame 4 {
                    n486 = Bundle("State"=State."Channel4", "Channel 4"="Channel 4") -> (w1567:T43)  [unwired: 1 in]
                  }
                }
                n487 = Enqueue Element(queue=w1538, element=w1537, error in (no error)=w1539) -> ()  [unwired: 1 in, 3 out]
              }
              event "Channel 1 Sample", "Channel 2 Sample", "Channel 3 Sample", "Channel 4 Sample": Value Change {
                n488 = event-data() -> ("CtlRef"=w1581:refnum<vi>)  [unwired: 1 in]
                n489 = property class="Clust (strict)"(reference=w1581) -> ("Label.Text"=w1580:string)  [unwired: 1 in, 2 out]
                n490 = Match Pattern(string=w1580, regular expression="Channel") -> (after substring=w1571:string)  [unwired: 1 in, 3 out]
                n491 = Match Pattern(string=w1571, regular expression="Sample") -> (before substring=w1572:string)  [unwired: 1 in, 3 out]
                n492 = Decimal String To Number(string=w1572) -> (number=w1578:i32)  [unwired: 2 in, 1 out]
                n493 = case shown="4" w1578 {
                  tunnel: w1577 -> [w1584 w1588 w1593 w1598 w1603]
                  tunnel: w1576 -> [w1583 w1589 w1594 w1599 w1604]
                  tunnel: [w1583 w1589 w1594 w1599 w1604] -> w1575
                  tunnel: [w1584 w1588 w1593 w1598 w1603] -> w1574
                  tunnel: [cluster{"State":T15, "Data":variant} {"State"=enum."Update", "Data"=variant} w1586 w1592 w1596 w1602] -> w1573
                  frame 0, Default {
                  }
                  frame 1 {
                    n494 = Bundle("State"=State."Channel1 Sample", "Channel 1 Sample"="Channel 1 Sample") -> (w1586:T44)  [unwired: 1 in]
                  }
                  frame 2 {
                    n495 = Bundle("State"=State."Channel2 Sample", "Channel 2 Sample"="Channel 2 Sample") -> (w1592:T45)  [unwired: 1 in]
                  }
                  frame 3 {
                    n496 = Bundle("State"=State."Channel3 Sample", "Channel 3 Sample"="Channel 3 Sample") -> (w1596:T46)  [unwired: 1 in]
                  }
                  frame 4 {
                    n497 = Bundle("State"=State."Channel4 Sample", "Channel 4 Sample"="Channel 4 Sample") -> (w1602:T47)  [unwired: 1 in]
                  }
                }
                n498 = Enqueue Element(queue=w1574, element=w1573, error in (no error)=w1575) -> ()  [unwired: 1 in, 3 out]
              }
              event "Sampling rate": Value Change {
                n499 = event-data() -> ()  [unwired: 1 in, 1 out]
                n500 = Bundle By Name(cluster=cluster{"State":T15, "Data":variant} {"State"=enum."DAQ Rate", "Data"=variant}, "Data"="Sampling rate") -> (w1605:cluster{"State":T15, "Data":variant})
                n501 = Enqueue Element(queue=w1609, element=w1605, error in (no error)=w1608) -> ()  [unwired: 1 in, 3 out]
              }
              event "Model List": Value Change {
                n502 = event-data() -> ("NewVal"=w1610:i32)  [unwired: 1 in]
                n503 = Bundle By Name(cluster=cluster{"State":T15, "Data":variant} {"State"=enum."ModelList", "Data"=variant}, "Data"=w1610) -> (w1612:cluster{"State":T15, "Data":variant})
                n504 = Enqueue Element(queue=w1613, element=w1612, error in (no error)=w1614) -> ()  [unwired: 1 in, 3 out]
              }
              event Value Change {
                n505 = event-data() -> ()  [unwired: 1 in, 1 out]
                n506 = Enqueue Element(queue=w1616, element=cluster{"State":T15, "Data":variant} {"State"=enum."Add", "Data"=variant}, error in (no error)=w1617) -> ()  [unwired: 1 in, 3 out]
              }
              event Value Change {
                n507 = event-data() -> ()  [unwired: 1 in, 2 out]
                n508 = property on="Model List" class="LstBox (strict)"() -> ("Item Names"=w1623:string[], "Value"=w1622:i32)  [unwired: 2 in, 2 out]
                n509 = Index Array(array=w1623, index=w1622) -> (element=w1620:string)
                n510 = Format Into String(format string="確認是否刪除設定 %s\nCheck Delete Set %s", w1620, w1620) -> (resulting string=w1619:string)  [unwired: 2 in, 1 out]
                n511 = Two Button Dialog(message=w1619) -> (T button?=w1618:bool)  [unwired: 2 in]
                n512 = case shown="True" w1618 {
                  tunnel: w1625 -> [_ w1628]
                  tunnel: w1624 -> [_ w1627]
                  frame False {
                  }
                  frame True {
                    n513 = Enqueue Element(queue=w1627, element=cluster{"State":T15, "Data":variant} {"State"=enum."Remove", "Data"=variant}, error in (no error)=w1628) -> ()  [unwired: 1 in, 3 out]
                  }
                }
              }
              event "Save Button": Value Change {
                n514 = event-data() -> ()  [unwired: 1 in, 2 out]
                n515 = Enqueue Element(queue=w1630, element=cluster{"State":T15, "Data":variant} {"State"=enum."Save", "Data"=variant}, error in (no error)=w1631) -> ()  [unwired: 1 in, 3 out]
              }
              event "Frontward": Value Change {
                n516 = event-data() -> ()  [unwired: 1 in, 2 out]
                n517 = Enqueue Element(queue=w1634, element=cluster{"State":T15, "Data":variant} {"State"=enum."Frontward", "Data"=variant}, error in (no error)=w1635) -> ()  [unwired: 1 in, 3 out]
                n518 = local write "Frontward"(FALSE ("Frontward")) -> ()
              }
              event "Leftward": Value Change {
                n519 = event-data() -> ()  [unwired: 1 in, 2 out]
                n520 = Enqueue Element(queue=w1638, element=cluster{"State":T15, "Data":variant} {"State"=enum."Leftward", "Data"=variant}, error in (no error)=w1639) -> ()  [unwired: 1 in, 3 out]
                n521 = local write "Leftward"(FALSE ("Leftward")) -> ()
              }
              event "Backward": Value Change {
                n522 = event-data() -> ()  [unwired: 1 in, 2 out]
                n523 = Enqueue Element(queue=w1642, element=cluster{"State":T15, "Data":variant} {"State"=enum."Backward", "Data"=variant}, error in (no error)=w1643) -> ()  [unwired: 1 in, 3 out]
                n524 = local write "Backward"(FALSE ("Backward")) -> ()
              }
              event "Rightward": Value Change {
                n525 = event-data() -> ()  [unwired: 1 in, 2 out]
                n526 = Enqueue Element(queue=w1646, element=cluster{"State":T15, "Data":variant} {"State"=enum."Rightward", "Data"=variant}, error in (no error)=w1647) -> ()  [unwired: 1 in, 3 out]
                n527 = local write "Rightward"(FALSE ("Rightward")) -> ()
              }
              event "Center": Value Change {
                n528 = event-data() -> ()  [unwired: 1 in, 6 out]
                n529 = Enqueue Element(queue=w1650, element=cluster{"State":T15, "Data":variant} {"State"=enum."Center", "Data"=variant}, error in (no error)=w1651) -> ()  [unwired: 1 in, 3 out]
                n530 = local write "Center"(FALSE ("Center")) -> ()
              }
              event "Bump": Value Change {
                n531 = event-data() -> ()  [unwired: 1 in, 6 out]
                n532 = Enqueue Element(queue=w1654, element=cluster{"State":T15, "Data":variant} {"State"=enum."Bump", "Data"=variant}, error in (no error)=w1655) -> ()  [unwired: 1 in, 3 out]
                n533 = local write "Bump"(FALSE ("Bump")) -> ()
              }
              event "Add Project": Value Change {
                n534 = event-data() -> ()  [unwired: 1 in, 6 out]
                n535 = Enqueue Element(queue=w1657, element=cluster{"State":T15, "Data":variant} {"State"=enum."Add Project", "Data"=variant}, error in (no error)=w1658) -> ()  [unwired: 1 in, 3 out]
              }
              event "Remove Project": Value Change {
                n536 = event-data() -> ()  [unwired: 1 in, 6 out]
                n537 = Enqueue Element(queue=w1660, element=cluster{"State":T15, "Data":variant} {"State"=enum."Remove Project", "Data"=variant}, error in (no error)=w1661) -> ()  [unwired: 1 in, 3 out]
              }
              event "Project Name": Value Change {
                n538 = event-data() -> ("NewVal"=w1662:string)  [unwired: 1 in]
                n539 = Bundle By Name(cluster=cluster{"State":T15, "Data":variant} {"State"=enum."Project Name", "Data"=variant}, "Data"=w1662) -> (w1663:cluster{"State":T15, "Data":variant})
                n540 = Enqueue Element(queue=w1665, element=w1663, error in (no error)=w1666) -> ()  [unwired: 1 in, 3 out]
              }
              event "Project List": Value Change {
                n541 = event-data() -> ("NewVal"=w1667:i32)  [unwired: 1 in, 5 out]
                n542 = Bundle By Name(cluster=cluster{"State":T15, "Data":variant} {"State"=enum."Project List", "Data"=variant}, "Data"=w1667) -> (w1668:cluster{"State":T15, "Data":variant})
                n543 = Enqueue Element(queue=w1670, element=w1668, error in (no error)=w1671) -> ()  [unwired: 1 in, 3 out]
              }
              event "OK Button": Value Change {
                n544 = event-data() -> ()  [unwired: 1 in, 6 out]
                n545 = Enqueue Element(queue=w1674, element=cluster{"State":T15, "Data":variant} {"State"=enum."Project OK", "Data"=variant}, error in (no error)=w1673) -> ()  [unwired: 1 in, 3 out]
              }
              event "Stop Button": Value Change {
                n546 = event-data() -> ()  [unwired: 1 in, 2 out]
                n547 = Enqueue Element(queue=w1677, element=cluster{"State":T15, "Data":variant} {"State"=enum."Stop", "Data"=variant}, error in (no error)=w1678) -> ()  [unwired: 1 in, 3 out]
                n548 = global write "GBV_Ref.vi" "Stop"(TRUE ("Stop")) -> ()
              }
              event "Project(Main)": Value Change {
                n549 = event-data() -> ()  [unwired: 1 in, 6 out]
                n550 = property on="Tab Control" class="TabCtl (strict)"("Value"=enum32{"Main", "Project", "Set"}."Project" ("Tab Control")) -> ()  [unwired: 2 in, 2 out]
              }
              event "Setting(Main)": Value Change {
                n551 = event-data() -> ()  [unwired: 1 in, 6 out]
                n552 = property on="Tab Control" class="TabCtl (strict)"("Value"=enum32{"Main", "Project", "Set"}."Set" ("Tab Control")) -> ()  [unwired: 2 in, 2 out]
              }
              event "Simple Test(Project)": Value Change {
                n553 = event-data() -> ()  [unwired: 1 in, 6 out]
                n554 = property on="Tab Control" class="TabCtl (strict)"("Value"=enum32{"Main", "Project", "Set"}."Main" ("Tab Control")) -> ()  [unwired: 2 in, 2 out]
              }
              event "Setting(Project)": Value Change {
                n555 = event-data() -> ()  [unwired: 1 in, 2 out]
                n556 = Bundle By Name(cluster=cluster{"State":T15, "Data":variant} {"State"=enum."ModelList", "Data"=variant} ("element"), "Data"=0) -> (w1683:cluster{"State":T15, "Data":variant})
                n557 = property on="Tab Control" class="TabCtl (strict)"("Value"=enum32{"Main", "Project", "Set"}."Set" ("Tab Control")) -> ()  [unwired: 2 in, 2 out]
                n558 = Enqueue Element(queue=w1685, element=w1683, error in (no error)=w1686) -> ()  [unwired: 1 in, 3 out]
              }
              event "Project(Setting)": Value Change {
                n559 = event-data() -> ()  [unwired: 1 in, 1 out]
                n560 = property on="Tab Control" class="TabCtl (strict)"("Value"=enum32{"Main", "Project", "Set"}."Project" ("Tab Control")) -> ()  [unwired: 2 in, 2 out]
              }
              event "Simple Test(Setting)": Value Change {
                n561 = event-data() -> ()  [unwired: 1 in, 6 out]
                n562 = property on="Tab Control" class="TabCtl (strict)"("Value"=enum32{"Main", "Project", "Set"}."Main" ("Tab Control")) -> ()  [unwired: 2 in, 2 out]
              }
              event Value Change {
                n563 = event-data() -> ()  [unwired: 1 in, 6 out]
                n564 = flat-sequence {
                  tunnel: [w1691] -> w1690
                  tunnel: w1690 -> [w1698]
                  frame #0 {
                    n565 = property on="SequenceList" class="LstBox (strict)"() -> ("Item Names"=w1692:string[])  [unwired: 2 in, 2 out]
                    n566 = property on="Model List" class="LstBox (strict)"() -> ("Item Names"=w1694:string[], "Value"=w1695:i32)  [unwired: 2 in, 2 out]
                    n567 = Index Array(array=w1694, index=w1695) -> (element=w1693:string)
                    n568 = Build Array (concatenate)(w1692, w1693) -> (w1691:string[])
                    n569 = property on="SequenceList" class="LstBox (strict)"("Item Names"=w1691) -> ()  [unwired: 2 in, 2 out]
                  }
                  frame #1 {
                    n570 = property on="SequenceName" class="Ring (strict)"() -> ("RingText.Text"=w1696:string)  [unwired: 2 in, 2 out]
                    n571 = Bundle("RingText.Text"=w1696, w1698) -> (w1697:cluster{"RingText.Text":string, string[]})  [unwired: 1 in]
                    n572 = call "Virbration SequenceFGV.vi"("Action"=T22."Write", "VirbSeqData"=w1697, "DataIn"=w1696) -> ()  [unwired: 10 in, 3 out]
                  }
                }
              }
              event "Btn_AddSeqName": Value Change {
                n573 = event-data() -> ()  [unwired: 1 in, 6 out]
                n574 = call "Prompt User for Input"() -> ("名稱/Name"=w1700:string, "OK"=w1701:bool)  [unwired: 17 in, 1 out]
                n575 = case shown="True" w1701 {
                  tunnel: w1700 -> [_ w1702]
                  frame False {
                  }
                  frame True {
                    n576 = property on="SequenceName" class="Ring (strict)"() -> ("Strings []"=w1704:string[])  [unwired: 2 in, 2 out]
                    n577 = for {
                      tunnel: w1704 -> [w1718] mode=indexing
                      tunnel: w1702 -> [w1717]
                      tunnel: [w1716] -> w1703
                      stop <- w1716 stop-if-true
                      n578 = Equal?(x=w1718, y=w1717) -> (x = y?=w1716:bool)
                    }
                    n579 = case shown="False" w1703 {
                      tunnel: w1702 -> [w1705 _]
                      frame False {
                        n580 = property on="SequenceName" class="Ring (strict)"() -> ("Strings []"=w1708:string[])  [unwired: 2 in, 2 out]
                        n581 = Build Array (concatenate)(w1708, w1705) -> (w1707:string[])
                        n582 = call "Virbration SequenceFGV.vi"("Action"=T22."Add", "DataIn"=w1705) -> ()  [unwired: 11 in, 3 out]
                        n583 = property on="SequenceName" class="Ring (strict)"("Strings []"=w1707) -> ()  [unwired: 2 in, 2 out]
                      }
                      frame True {
                        n584 = Unbundle By Name(errorcluster {"status"=TRUE, "code"=10500, "source"="震動盤Sequence名稱重複/Project Name Repeat"} ("error constant")) -> ("source"=w1711:string, "code"=w1710:i32)
                        n585 = Format Into String(format string="ErrorCode:%d_ErrorMsg:%s", w1710, w1711) -> (resulting string=w1712:string)  [unwired: 2 in, 1 out]
                        n586 = One Button Dialog(message=w1711) -> ()  [unwired: 1 in, 1 out]
                        n587 = Bundle By Name(cluster=T18 {"MsgPageSelect"=enum."Alarm", "LogType"=enum."Auto", "Msg"="", "Time"=""} ("DataIn"), "Msg"=w1712) -> (w1713:T18)
                        n588 = call "SendMsg.vi"("DataIn"=w1713) -> ()  [unwired: 10 in, 1 out]
                      }
                    }
                  }
                }
              }
              event "Btn_DelSeqName": Value Change {
                n589 = event-data() -> ()  [unwired: 1 in, 6 out]
                n590 = property on="SequenceName" class="Ring (strict)"() -> ("RingText.Text"=w1720:string, "Value"=w1719:u16)  [unwired: 2 in, 2 out]
                n591 = Format Into String(format string="是否刪除排程:%s?\nMake Sure Delete Sequence:%s", w1720, w1720) -> (resulting string=w1722:string)  [unwired: 2 in, 1 out]
                n592 = Two Button Dialog(message=w1722) -> (T button?=w1721:bool)  [unwired: 2 in]
                n593 = case shown="True" w1721 {
                  tunnel: w1720 -> [_ w1728]
                  tunnel: w1719 -> [_ w1725]
                  frame False {
                  }
                  frame True {
                    n594 = property on="SequenceName" class="Ring (strict)"() -> ("Strings []"=w1727:string[])  [unwired: 2 in, 2 out]
                    n595 = call "Virbration SequenceFGV.vi"("Action"=T22."Delete", "DataIn"=w1728) -> ()  [unwired: 11 in, 3 out]
                    n596 = Delete From Array(array=w1727, length=1, index=w1725) -> (array with subset deleted=w1726:string[])  [unwired: 1 out]
                    n597 = property on="SequenceName" class="Ring (strict)"("Strings []"=w1726) -> ()  [unwired: 2 in, 2 out]
                  }
                }
              }
              event Value Change {
                n598 = event-data() -> ()  [unwired: 1 in, 6 out]
                n599 = flat-sequence {
                  tunnel: [w1731] -> w1730
                  tunnel: w1730 -> [w1735]
                  frame #0 {
                    n600 = property on="SequenceList" class="LstBox (strict)"() -> ("Item Names"=w1734:string[], "Value"=w1733:i32)  [unwired: 2 in, 2 out]
                    n601 = Delete From Array(array=w1734, length=1, index=w1733) -> (array with subset deleted=w1731:string[])  [unwired: 1 out]
                    n602 = property on="SequenceList" class="LstBox (strict)"("Item Names"=w1731) -> ()  [unwired: 2 in, 2 out]
                  }
                  frame #1 {
                    n603 = property on="SequenceName" class="Ring (strict)"() -> ("RingText.Text"=w1737:string)  [unwired: 2 in, 2 out]
                    n604 = Bundle("RingText.Text"=w1737, "Item Names"=w1735) -> (w1738:T48)  [unwired: 1 in]
                    n605 = call "Virbration SequenceFGV.vi"("Action"=T22."Write", "VirbSeqData"=w1738, "DataIn"=w1737) -> ()  [unwired: 10 in, 3 out]
                  }
                }
              }
              event "SequenceName": Value Change; "SequenceName": Mouse Down {
                n606 = event-data() -> ()  [unwired: 1 in, 4 out]
                n607 = property on="SequenceName" class="Ring (strict)"() -> ("RingText.Text"=w1741:string)  [unwired: 2 in, 2 out]
                n608 = call "Virbration SequenceFGV.vi"("Action"=T22."Read", "DataIn"=w1741) -> ("VirbSeqData"=w1740:T49)  [unwired: 11 in, 2 out]
                n609 = Unbundle By Name(w1740) -> ("VirbSeqStep"=w1739:string[])
                n610 = property on="SequenceList" class="LstBox (strict)"("Item Names"=w1739) -> ()  [unwired: 2 in, 2 out]
              }
            }
            n611 = call "FGV_EXIT.vi"("Function"=enum16{"Read", "Write"}."Read") -> ("EXIT out"=w1507:bool)  [unwired: 7 in]
            n612 = Or(x=w1512, y=w1507) -> (x .or. y?=w1509:bool)
          }
          n613 = disable-structure shown="Enabled" {
            disable-tunnel: w121 -> [w229 _]
            disable-tunnel: w118 -> [w228 _]
            disable-tunnel: w117 -> [w227 _]
            frame Enabled {
              n614 = while {
                tunnel: w229 -> [w239]
                tunnel: w228 -> [w232]
                tunnel: w227 -> [w230]
                stop <- w237 stop-if-true
                n615 = call <vilib>:"TCP Listen.vi"("error in (no error)"=w232, "timeout ms (wait forever: -1)"=1000, "port"=u16 6025) -> ("error out"=w235:errorcluster, "connection ID"=w234:refnum<k5>)  [unwired: 4 in, 3 out]
                n616 = Wait (ms)(milliseconds to wait=u32 1) -> ()  [unwired: 1 out]
                n617 = case shown="Error" w235 {
                  selector: w235 -> [w241 w398]
                  tunnel: [w245 w396] -> _
                  tunnel: w234 -> [w251 _]
                  tunnel: w239 -> [w250 _]
                  tunnel: w230 -> [w247 _]
                  frame No Error {
                    n618 = property on="Connect" class="Bool (strict)"(error in=w241, "Value"=TRUE ("Connect")) -> (error out=w240:errorcluster)  [unwired: 1 in, 1 out]
                    n619 = while {
                      tunnel: w241 -> [w387]
                      tunnel: w251 -> [w386]
                      tunnel: w250 -> [w385]
                      tunnel: [w379] -> w249
                      stop <- w378 stop-if-true
                      n620 = Dequeue Element(queue=w385, timeout in ms (-1)=100, error in (no error)=w387) -> (element=w375:string, error out=w388:errorcluster)  [unwired: 2 out]
                      n621 = To Lower Case(string=w375) -> (all lower case string=w374:string)
                      n622 = Empty String/Path?(string/path=w375) -> (empty?=w380:bool)
                      n623 = Equal?(x=w374, y="close") -> (x = y?=w377:bool)
                      n624 = case shown="False" w380 {
                        tunnel: w375 -> [w394 _]
                        tunnel: w388 -> [w393 w395]
                        tunnel: w386 -> [w392 _]
                        tunnel: [w391 w395] -> w379
                        frame False {
                          n625 = Concatenate Strings(w394, "\r\n") -> (w390:string)
                          n626 = TCP Write(connection ID=w392, data in=w390, error in (no error)=w393) -> (error out=w391:errorcluster)  [unwired: 1 in, 2 out]
                        }
                        frame True {
                        }
                      }
                      n627 = call "FGV_EXIT.vi"("Function"=enum16{"Read", "Write"}."Read") -> ("EXIT out"=w381:bool)  [unwired: 7 in]
                      n628 = property on="TCP connect" class="Bool (strict)"() -> ("Value"=w373:bool)  [unwired: 2 in, 2 out]
                      n629 = Wait (ms)(milliseconds to wait=u32 1) -> ()  [unwired: 1 out]
                      n630 = Compound Arithmetic op=OR(w379, w373, w377, w381) -> (w378:bool)
                    }
                    n631 = while {
                      tunnel: w251 -> [w270]
                      tunnel: w241 -> [w269]
                      tunnel: [w261] -> w248
                      tunnel: w247 -> [w257]
                      tunnel: w240 -> [_]
                      stop <- w256 stop-if-true
                      w266 = 56 items=["No Error", "Argument Error", "Memory Full", "Out of Zone", "End of File", "File Already Open", "Generic File IO Error", "File Not Found", "File Permission Error", "Disk Full", "Duplicate Path", "Too Many Files Open", "Not Enabled", "Resource File Not Found", "Cannot Add Resource", "Resource Not Found", "Image Not Found", "Image Memory Error", "Pen Does Not Exist", "Config Bad Type", "Config Token Not Found", "Config Parse Error", "Config Memory Error", "Bad External Code Format", "Bad External Code Offset", "External Code Not Present", "Null Window", "Destroy Window Mixup", "Null Menu", "Print Aborted", "Bad Print Record", "Print Driver Error", "Windows Error During Print", "Memory Error During Print", "Print Dialog Error", "Generic Print Error", "Invalid Device Refnum", "Device Not Found", "Device Parameter Error", "Device Unit Error", "Can't Open Device", "Device Call Aborted", "Generic Error", "Cancelled By User", "Object ID Too Low", "Object ID Too High", "Object Not In Heap", "Unknown Heap", "Bad DefProc ID", "DefProc Not In Table", "Message Out Of Range", "Null Method", "Unknown Message", "Manager Call Not Supported", "Bad address", "Connection In progress", "Connection timed out", "Connection is already in progress", "Network attribute not supported", "Network error", "Address in use", "System out of memory", "Connection aborted", "Connection refused", "Connection is not connected", "Connection is already connected", "Connection closed", "Initialize error (interapplication manager)", "Bad occurrence", "Wait on unbound occurrence handler", "Occurrence queue overflow", "Bad path", "Semaphore not signaled", "Unrecognized type (interapplication manager)"] ("1st Error to Convert")
                      n632 = TCP Read(connection ID=w270, bytes to read=5000, error in (no error)=w269, 7:T17."Standard" ("mode (standard)"), 9:100 ("timeout ms (25000)")) -> (connection ID out=w252:refnum<k5>, data out=w268:string, error out=w267:errorcluster)
                      n633 = Wait (ms)(milliseconds to wait=u32 1) -> ()  [unwired: 1 out]
                      n634 = call <vilib>:"Trim Whitespace.vi"("string"=w268) -> ("trimmed string"=w259:string)  [unwired: 1 in]
                      n635 = call <vilib>:"Error to Warning.vi"("1st Error to Convert"=w266, "error in"=w267) -> ("warning out"=w254:errorcluster)  [unwired: 13 in]
                      n636 = Empty String/Path?(string/path=w259) -> (empty?=w265:bool)
                      n637 = To Lower Case(string=w259) -> (all lower case string=w258:string)
                      n638 = case shown="False" w265 {
                        tunnel: w254 -> [w275 w372]
                        tunnel: [w279 w372] -> w261
                        tunnel: w258 -> [w277 _]
                        tunnel: w257 -> [w278 _]
                        tunnel: w252 -> [w272 _]
                        frame False {
                          n639 = call "TCPIP_CMD.vi"("error in (no error)"=w275, "CMD"=w277) -> ("error out"=w274:errorcluster, "Output"=w273:string, "State"=w276:string)  [unwired: 7 in]
                          n640 = case shown="\"MODEL\"" w276 {
                            tunnel: w274 -> [w282 w291 w315 w324 w346 w350 w353 w358 w371]
                            tunnel: [w281 w292 w315 w323 w345 w349 w352 w359 w371] -> w279
                            tunnel: w278 -> [w280 w293 _ w322 w344 w347 w351 w356 _]
                            tunnel: w273 -> [_ w285 _ w321 _ _ _ _ _]
                            tunnel: w272 -> [_ w286 _ w316 _ _ _ _ w370]
                            frame "STOP" {
                              n641 = Enqueue Element(queue=w280, element=cluster{"State":T15, "Data":variant} {"State"=enum."Stop", "Data"=variant}, error in (no error)=w282) -> (error out=w281:errorcluster)  [unwired: 1 in, 2 out]
                            }
                            frame "PROJECT" {
                              n642 = property on="Project List" class="LstBox (strict)"(error in=w291) -> (error out=w287:errorcluster, "Item Names"=w290:string[])  [unwired: 1 in, 1 out]
                              n643 = To Upper Case(1:w290) -> (0:w289:string[])
                              n644 = Search 1D Array(1D array=w289, element=w285) -> (index of element=w284:i32)  [unwired: 1 in]
                              n645 = Greater Or Equal To 0?(x=w284) -> (x >= 0?=w288:bool)
                              n646 = case shown="True" w288 {
                                tunnel: w293 -> [_ w310]
                                tunnel: [w298 w309] -> w292
                                tunnel: w287 -> [w299 w308]
                                tunnel: w286 -> [w297 _]
                                tunnel: w285 -> [_ _]
                                tunnel: w284 -> [_ w306]
                                frame False {
                                n647 = Concatenate Strings("error", "\r\n") -> (w296:string)
                                n648 = TCP Write(connection ID=w297, data in=w296, error in (no error)=w299) -> (error out=w298:errorcluster)  [unwired: 1 in, 2 out]
                                }
                                frame True {
                                n649 = Bundle By Name(cluster=cluster{"State":T15, "Data":variant} {"State"=enum."Project List", "Data"=variant}, "Data"=w306) -> (w305:cluster{"State":T15, "Data":variant})
                                n650 = Bundle By Name(cluster=cluster{"State":T15, "Data":variant} {"State"=enum."Response", "Data"=variant}, "Data"="ok") -> (w301:cluster{"State":T15, "Data":variant})
                                n651 = Build Array(w305, cluster{"State":T15, "Data":variant} {"State"=enum."Project OK", "Data"=variant}, w301) -> (w303:cluster{"State":T15, "Data":variant}[])
                                n652 = for {
                                tunnel: w310 -> [w314]
                                shift-right: [w313] -> w309
                                shift-left: w308 -> [w312]
                                tunnel: w303 -> [w311] mode=indexing
                                n653 = Enqueue Element(queue=w314, element=w311, error in (no error)=w312) -> (error out=w313:errorcluster)  [unwired: 1 in, 2 out]
                                }
                                }
                              }
                            }
                            frame Default {
                            }
                            frame "MODEL" {
                              n654 = property on="Model List" class="LstBox (strict)"() -> ("Item Names"=w320:string[])  [unwired: 2 in, 2 out]
                              n655 = Decimal String To Number(string=w321) -> (number=w318:i32)  [unwired: 2 in, 1 out]
                              n656 = Array Size(array=w320) -> (size(s)=w319:i32)
                              n657 = Less?(x=w319, y=w318) -> (x < y?=w317:bool)
                              n658 = case shown="False" w317 {
                                tunnel: w324 -> [w333 w342]
                                tunnel: [w332 w342] -> w323
                                tunnel: w322 -> [w331 _]
                                tunnel: w318 -> [w329 _]
                                tunnel: w316 -> [_ w339]
                                frame False {
                                n659 = Bundle By Name(cluster=cluster{"State":T15, "Data":variant} {"State"=enum."ModelList", "Data"=variant}, "Data"=w329) -> (w328:cluster{"State":T15, "Data":variant})
                                n660 = Build Array(w328, cluster{"State":T15, "Data":variant} {"State"=enum."Test", "Data"=variant}) -> (w326:cluster{"State":T15, "Data":variant}[])
                                n661 = for {
                                tunnel: w331 -> [w335]
                                shift-right: [w336] -> w332
                                shift-left: w333 -> [w337]
                                tunnel: w326 -> [w334] mode=indexing
                                n662 = Enqueue Element(queue=w335, element=w334, error in (no error)=w337) -> (error out=w336:errorcluster)  [unwired: 1 in, 2 out]
                                }
                                n663 = local write "Reply"(TRUE ("Reply")) -> ()
                                }
                                frame True {
                                n664 = Concatenate Strings("error" ("string"), "\r\n") -> (w341:string)
                                n665 = TCP Write(connection ID=w339, data in=w341) -> ()  [unwired: 2 in, 3 out]
                                }
                              }
                            }
                            frame "RIGHT" {
                              n666 = Enqueue Element(queue=w344, element=cluster{"State":T15, "Data":variant} {"State"=enum."ModelList", "Data"=variant}, error in (no error)=w346) -> (error out=w345:errorcluster)  [unwired: 1 in, 2 out]
                            }
                            frame "BACK" {
                              n667 = Enqueue Element(queue=w347, element=cluster{"State":T15, "Data":variant} {"State"=enum."Backward", "Data"=variant}, error in (no error)=w350) -> (error out=w349:errorcluster)  [unwired: 1 in, 2 out]
                            }
                            frame "LEFT" {
                              n668 = Enqueue Element(queue=w351, element=cluster{"State":T15, "Data":variant} {"State"=enum."Leftward", "Data"=variant}, error in (no error)=w353) -> (error out=w352:errorcluster)  [unwired: 1 in, 2 out]
                            }
                            frame "EXIT" {
                              n669 = Flush Queue(queue=w356, error in (no error)=w358) -> (queue out=w355:refnum<queue>, error out=w357:errorcluster)  [unwired: 1 out]
                              n670 = Enqueue Element(queue=w355, element=cluster{"State":T15, "Data":variant} {"State"=enum."Exit", "Data"=variant}, error in (no error)=w357) -> (error out=w359:errorcluster)  [unwired: 1 in, 2 out]
                            }
                            frame "CHECK" {
                              n671 = local read "Vibration State"() -> (w364:bool)
                              n672 = local read "Testing"() -> (w367:bool)
                              n673 = Select(t="busy", s=w367, f="idle") -> (s? t:f=w363:string)
                              n674 = Select(t=w363, s=w364, f="disconnect") -> (s? t:f=w361:string)
                              n675 = Concatenate Strings(w361, "\r\n") -> (w368:string)
                              n676 = TCP Write(connection ID=w370, data in=w368) -> ()  [unwired: 2 in, 3 out]
                            }
                          }
                        }
                        frame True {
                          # "Wait CMD"
                        }
                      }
                      n677 = Unbundle By Name(w254) -> ("status"=→"TCP connect":bool)
                      n678 = call "FGV_EXIT.vi"("Function"=enum16{"Read", "Write"}."Read") -> ("EXIT out"=w255:bool)  [unwired: 7 in]
                      n679 = Or(x=w255, y=w254) -> (x .or. y?=w256:bool)
                    }
                    n680 = Merge Errors(w249, w248) -> (w246:errorcluster)
                    n681 = call <vilib>:"Clear Errors.vi"("error in (no error)"=w246) -> ("error out"=w243:errorcluster)  [unwired: 5 in, 1 out]
                    n682 = property on="TCP connect" class="Bool (strict)"(error in=w243, "Value"=FALSE ("TCP connect")) -> (error out=w245:errorcluster)  [unwired: 1 in, 1 out]
                  }
                  frame Error {
                    w399 = 56 items=["No Error", "Argument Error", "Memory Full", "Out of Zone", "End of File", "File Already Open", "Generic File IO Error", "File Not Found", "File Permission Error", "Disk Full", "Duplicate Path", "Too Many Files Open", "Not Enabled", "Resource File Not Found", "Cannot Add Resource", "Resource Not Found", "Image Not Found", "Image Memory Error", "Pen Does Not Exist", "Config Bad Type", "Config Token Not Found", "Config Parse Error", "Config Memory Error", "Bad External Code Format", "Bad External Code Offset", "External Code Not Present", "Null Window", "Destroy Window Mixup", "Null Menu", "Print Aborted", "Bad Print Record", "Print Driver Error", "Windows Error During Print", "Memory Error During Print", "Print Dialog Error", "Generic Print Error", "Invalid Device Refnum", "Device Not Found", "Device Parameter Error", "Device Unit Error", "Can't Open Device", "Device Call Aborted", "Generic Error", "Cancelled By User", "Object ID Too Low", "Object ID Too High", "Object Not In Heap", "Unknown Heap", "Bad DefProc ID", "DefProc Not In Table", "Message Out Of Range", "Null Method", "Unknown Message", "Manager Call Not Supported", "Bad address", "Connection In progress", "Connection timed out", "Connection is already in progress", "Network attribute not supported", "Network error", "Address in use", "System out of memory", "Connection aborted", "Connection refused", "Connection is not connected", "Connection is already connected", "Connection closed", "Initialize error (interapplication manager)", "Bad occurrence", "Wait on unbound occurrence handler", "Occurrence queue overflow", "Bad path", "Semaphore not signaled", "Unrecognized type (interapplication manager)"] ("1st Error to Convert")
                    n683 = call <vilib>:"Error to Warning.vi"("1st Error to Convert"=w399, "error in"=w398) -> ("warning out"=w396:errorcluster)  [unwired: 13 in]
                    n684 = property on="Connect" class="Bool (strict)"(error in=w396, "Value"=FALSE ("Connect")) -> ()  [unwired: 1 in, 2 out]
                  }
                }
                n685 = call "FGV_EXIT.vi"("Function"=enum16{"Read", "Write"}."Read") -> ("EXIT out"=w237:bool)  [unwired: 7 in]
              }
            }
            frame Disabled {
            }
          }
          n686 = while {
            tunnel: w125 -> [_]
            tunnel: w124 -> [w400]
            stop <- w403 stop-if-true
            n687 = property on="Testing?" class="Bool (strict)"() -> ("Value"=w402:bool)  [unwired: 2 in, 2 out]
            n688 = Wait (ms)(milliseconds to wait=u32 1) -> ()  [unwired: 1 out]
            n689 = case shown="True" w402 {
              tunnel: w400 -> [_ w405]
              frame False {
              }
              frame True {
                n690 = property on="Test State" class="Enum (strict)"() -> ("Value"=w406:T4)  [unwired: 2 in, 2 out]
                n691 = case shown="\"Normal\", Default" w406 {
                  tunnel: w405 -> [w411 w412 w433]
                  frame "Normal", Default {
                    n692 = property on="Test Setting" class="Arr (strict)"() -> ("Value"=w410:waveform(dbl)[])  [unwired: 2 in, 2 out]
                    n693 = property on="Sampling rate" class="DigNum (strict)"() -> ("Value"=w407:dbl)  [unwired: 2 in, 2 out]
                    n694 = call "DAQ Test.vi"("rate"=w407, "data"=w410, "device name"=w411) -> ("error out"=w409:errorcluster)  [unwired: 7 in, 1 out]
                    n695 = call <vilib>:"Clear Errors.vi"("error in (no error)"=w409) -> ()  [unwired: 5 in, 2 out]
                    n696 = Not(x=w409) -> (.not. x?=w408:bool)
                    n697 = property on="Vibration State" class="Bool (strict)"("Value"=w408) -> ()  [unwired: 2 in, 2 out]
                  }
                  frame "Bump" {
                    n698 = Unbundle("Bump") -> ("Channel 1"=w422:T27, "Channel 2"=w421:T27, "Channel 3"=w420:T27, "Channel 4"=w419:T27)
                    n699 = Build Array(w422, w421, w420, w419) -> (w418:T29)
                    n700 = for {
                      tunnel: w418 -> [w424] mode=indexing
                      tunnel: [w425] -> w413 mode=indexing
                      n701 = Unbundle By Name(w424) -> ("offset"=w426:i32, "signal type 1"=w427:T30, "frequency 1"=w428:i32, "amplitude 1"=w429:dbl, "phase"=w430:dbl)
                      n702 = call <vilib>:"Basic Function Generator.vi"("offset"=w426, "reset signal"=TRUE, "sampling info"=cluster{"Fs":dbl, "#s":dbl} {"Fs"=1000.0, "#s"=100.0} ("sampling info 4"), "signal type"=w427, "phase"=w430, "amplitude"=w429, "frequency"=w428) -> ("signal out"=w425:waveform(dbl))  [unwired: 2 in, 2 out]
                    }
                    n703 = Index Array(array=w413) -> (element #1=w417:waveform(dbl), element #2=w416:waveform(dbl), element #3=w415:waveform(dbl), element #4=w414:waveform(dbl))  [unwired: 4 in]
                    n704 = property on="Channel 1 Wave (Main)" class="WFGraph (strict)"("Value"=w417) -> ()  [unwired: 2 in, 2 out]
                    n705 = property on="Channel 2 Wave (Main)" class="WFGraph (strict)"("Value"=w416) -> ()  [unwired: 2 in, 2 out]
                    n706 = property on="Channel 3 Wave (Main)" class="WFGraph (strict)"("Value"=w415) -> ()  [unwired: 2 in, 2 out]
                    n707 = property on="Channel 4 Wave (Main)" class="WFGraph (strict)"("Value"=w414) -> ()  [unwired: 2 in, 2 out]
                    n708 = call "DAQ Assistant"("data"=w413, "device name"=w412) -> ()  [unwired: 16 in, 2 out]
                  }
                  frame "Center" {
                    n709 = Unbundle("Center") -> ("Channel 1"=w443:T27, "Channel 2"=w442:T28, "Channel 3"=w441:T28, "Channel 4"=w440:T28)
                    n710 = Build Array(w443, w442, w441, w440) -> (w439:T29)
                    n711 = for {
                      tunnel: w439 -> [w445] mode=indexing
                      tunnel: [w446] -> w434 mode=indexing
                      n712 = Unbundle By Name(w445) -> ("offset"=w447:i32, "signal type 1"=w448:T30, "frequency 1"=w449:i32, "amplitude 1"=w450:dbl, "phase"=w451:dbl)
                      n713 = call <vilib>:"Basic Function Generator.vi"("offset"=w447, "reset signal"=TRUE, "sampling info"=cluster{"Fs":dbl, "#s":dbl} {"Fs"=1000.0, "#s"=100.0} ("sampling info 4"), "signal type"=w448, "phase"=w451, "amplitude"=w450, "frequency"=w449) -> ("signal out"=w446:waveform(dbl))  [unwired: 2 in, 2 out]
                    }
                    n714 = Index Array(array=w434) -> (element #1=w438:waveform(dbl), element #2=w437:waveform(dbl), element #3=w436:waveform(dbl), element #4=w435:waveform(dbl))  [unwired: 4 in]
                    n715 = property on="Channel 1 Wave (Main)" class="WFGraph (strict)"("Value"=w438) -> ()  [unwired: 2 in, 2 out]
                    n716 = property on="Channel 2 Wave (Main)" class="WFGraph (strict)"("Value"=w437) -> ()  [unwired: 2 in, 2 out]
                    n717 = property on="Channel 3 Wave (Main)" class="WFGraph (strict)"("Value"=w436) -> ()  [unwired: 2 in, 2 out]
                    n718 = property on="Channel 4 Wave (Main)" class="WFGraph (strict)"("Value"=w435) -> ()  [unwired: 2 in, 2 out]
                    n719 = call "DAQ Assistant5"("data"=w434, "device name"=w433) -> ()  [unwired: 16 in, 2 out]
                  }
                }
              }
            }
            n720 = call "FGV_EXIT.vi"("Function"=enum16{"Read", "Write"}."Read") -> ("EXIT out"=w403:bool)  [unwired: 7 in]
          }
          n721 = while {
            tunnel: w118 -> [_]
            shift-right: [w181] -> _
            shift-left: 0 -> [w182]
            stop <- w183 stop-if-true
            n722 = case shown="True" "Blank Button" {
              tunnel: w182 -> [_ w195]
              tunnel: [0 w196] -> w181
              frame False {
                n723 = Wait (ms)(milliseconds to wait=u32 500) -> ()  [unwired: 1 out]
              }
              frame True {
                w189 = i32[] [0, 1, 3, 5, 0, 2, 4, 5]
                n724 = control-ref of="Bump"() -> (w210:refnum<vi>)
                n725 = control-ref of="Frontward"() -> (w211:refnum<vi>)
                n726 = control-ref of="Leftward"() -> (w212:refnum<vi>)
                n727 = control-ref of="Backward"() -> (w213:refnum<vi>)
                n728 = control-ref of="Rightward"() -> (w214:refnum<vi>)
                n729 = control-ref of="Center"() -> (w215:refnum<vi>)
                n730 = control-ref of="Testing?"() -> (w216:refnum<vi>)
                n731 = Bundle("Bump"=w210, "Frontward"=w211, "Leftward"=w212, "Backward"=w213, "Rightward"=w214, "Center"=w215, "Testing?"=w216) -> (w197:T50)  [unwired: 1 in]
                n732 = Unbundle(w197) -> ("Bump"=w198:refnum<vi>, "Frontward"=w203:refnum<vi>, "Leftward"=w202:refnum<vi>, "Backward"=w201:refnum<vi>, "Rightward"=w200:refnum<vi>, "Center"=w199:refnum<vi>, "Testing?"=w206:refnum<vi>)
                n733 = Array Size(array=w189) -> (size(s)=w207:i32)
                n734 = Increment(x=w195) -> (x+1=w190:i32)
                n735 = Index Array(array=w189, index=w195) -> (element=w205:i32)
                n736 = Build Array(w198, w203, w202, w201, w200, w199) -> (w204:refnum<vi>[])
                n737 = Greater?(x=w207, y=w190) -> (0:w208:bool)
                n738 = Index Array(array=w204, index=w205) -> (element=w194:refnum<vi>)
                n739 = property class="Bool (strict)"(reference=w194, "Val(Sgnl)"=TRUE ("Value (Signaling)")) -> (error out=w193:errorcluster)  [unwired: 1 in, 1 out]
                n740 = Select(t=w190, s=w208, f=0 ("t")) -> (s? t:f=w196:i32)
                n741 = flat-sequence {
                  tunnel: w193 -> [_]
                  tunnel: w206 -> [w218]
                  tunnel: [w217] -> w209
                  tunnel: w209 -> [w223]
                  frame #0 {
                    n742 = while {
                      tunnel: w218 -> [w222]
                      tunnel: [w219] -> w217
                      stop <- w221 stop-if-true
                      n743 = property class="Bool (strict)"(reference=w222) -> (reference out=w219:refnum<vi>, "Value"=w221:bool)  [unwired: 1 in, 1 out]
                      n744 = Wait (ms)(milliseconds to wait=u32 1) -> ()  [unwired: 1 out]
                    }
                  }
                  frame #1 {
                    n745 = while {
                      tunnel: [w224] -> _
                      tunnel: w223 -> [w224]
                      stop <- w226 continue-if-true
                      n746 = property class="Bool (strict)"(reference=w224) -> ("Value"=w226:bool)  [unwired: 1 in, 2 out]
                      n747 = Wait (ms)(milliseconds to wait=u32 1) -> ()  [unwired: 1 out]
                    }
                  }
                }
              }
            }
            n748 = call "FGV_EXIT.vi"("Function"=enum16{"Read", "Write"}."Read") -> ("EXIT out"=w183:bool)  [unwired: 7 in]
            n749 = Wait (ms)(milliseconds to wait=u32 1) -> ()  [unwired: 1 out]
          }
          n750 = while {
            tunnel: w118 -> [_]
            tunnel: w117 -> [w131]
            shift-right: [w128] -> _
            shift-left: 0 -> [w129]
            stop <- w132 stop-if-true
            n751 = case shown="True" "TestListTrayRun" {
              tunnel: w131 -> [_ w149]
              tunnel: w129 -> [_ w136]
              tunnel: [0 w140] -> w128
              frame False {
                n752 = Wait (ms)(milliseconds to wait=u32 77) -> ()  [unwired: 1 out]
              }
              frame True {
                n753 = property on="SequenceList" class="LstBox (strict)"() -> ("Item Names"=w146:string[])  [unwired: 2 in, 2 out]
                n754 = property on="Model List" class="LstBox (strict)"() -> ("Item Names"=w139:string[])  [unwired: 2 in, 2 out]
                n755 = Index Array(array=w146, index=w136) -> (element=w152:string)
                n756 = Array Size(array=w146) -> (size(s)=w143:i32)
                n757 = To Upper Case(1:w139) -> (0:w154:string[])
                n758 = To Upper Case(1:w152) -> (0:w151:string)
                n759 = Search 1D Array(1D array=w154, element=w151) -> (index of element=w153:i32)  [unwired: 1 in]
                n760 = property on="SequenceList" class="LstBox (strict)"("Value"=w136) -> ()  [unwired: 2 in, 2 out]
                n761 = Bundle By Name(cluster=cluster{"State":T15, "Data":variant} {"State"=enum."ModelList", "Data"=variant}, "Data"=w153) -> (w155:cluster{"State":T15, "Data":variant})
                n762 = Build Array(w155, cluster{"State":T15, "Data":variant} {"State"=enum."Test", "Data"=variant}) -> (w150:cluster{"State":T15, "Data":variant}[])
                n763 = control-ref of="Testing?"() -> (w148:refnum<vi>)
                n764 = for {
                  tunnel: w149 -> [w160]
                  shift-right: [w159] -> w147
                  shift-left: _ -> [w158]
                  tunnel: w150 -> [w157] mode=indexing
                  n765 = Enqueue Element(queue=w160, element=w157, error in (no error)=w158) -> (error out=w159:errorcluster)  [unwired: 1 in, 2 out]
                }
                n766 = flat-sequence {
                  tunnel: w148 -> [w164]
                  tunnel: [w163] -> w156
                  tunnel: w147 -> [_]
                  tunnel: [w162] -> w144
                  tunnel: w143 -> [w162]
                  tunnel: [w161] -> w141
                  tunnel: w136 -> [w161]
                  tunnel: w156 -> [w171]
                  tunnel: [w170] -> w145
                  tunnel: w144 -> [w170]
                  tunnel: [w169] -> w142
                  tunnel: w141 -> [w169]
                  tunnel: w145 -> [w179]
                  tunnel: w142 -> [w180]
                  tunnel: [w177] -> w140
                  frame #0 {
                    n767 = while {
                      tunnel: w164 -> [w168]
                      tunnel: [w165] -> w163
                      stop <- w167 stop-if-true
                      n768 = property class="Bool (strict)"(reference=w168) -> (reference out=w165:refnum<vi>, "Value"=w167:bool)  [unwired: 1 in, 1 out]
                      n769 = Wait (ms)(milliseconds to wait=u32 1) -> ()  [unwired: 1 out]
                    }
                  }
                  frame #1 {
                    n770 = while {
                      tunnel: [w172] -> _
                      tunnel: w171 -> [w172]
                      stop <- w174 continue-if-true
                      n771 = property class="Bool (strict)"(reference=w172) -> ("Value"=w174:bool)  [unwired: 1 in, 2 out]
                      n772 = Wait (ms)(milliseconds to wait=u32 1) -> ()  [unwired: 1 out]
                    }
                  }
                  frame #2 {
                    n773 = Increment(x=w180) -> (x+1=w176:i32)
                    n774 = Less Or Equal?(x=w179, y=w176) -> (x <= y?=w175:bool)
                    n775 = case shown="True" w175 {
                      frame False {
                      }
                      frame True {
                        n776 = invoke on="TestListTrayRun" class="Bool (strict)" method="Reinit To Default"() -> ()  [unwired: 3 in, 3 out]
                      }
                    }
                    n777 = Select(t=0, s=w175, f=w176) -> (s? t:f=w177:i32)
                  }
                }
              }
            }
            n778 = call "FGV_EXIT.vi"("Function"=enum16{"Read", "Write"}."Read") -> ("EXIT out"=w132:bool)  [unwired: 7 in]
          }
          n779 = Enqueue Element(queue=w120, element=cluster{"State":T15, "Data":variant} {"State"=enum."Exit", "Data"=variant}) -> ()  [unwired: 2 in, 3 out]
        }
        frame #3 {
          n780 = disable-structure shown="RUN_TIME_ENGINE==True" {
            frame condition #0 (active) {
            }
            frame condition #1 {
              n781 = Quit LabVIEW(quit? (T)=TRUE) -> ()
            }
          }
        }
      }
    }
  }
